vi "TCE.vi"() -> (11 "placeholder image":T1(plugin-control))   [LabVIEW 2022 SP3]
uses:
  DataCluster_TCAL.ctl
  <vilib>/vision/Image Controls.llb/IMAQ Image.ctl
  TCE_Config.ctl
  <vilib>/Utility/file.llb/Read Delimited Spreadsheet (string).vi
  <vilib>/Utility/file.llb/Write Delimited Spreadsheet (string).vi
  <vilib>/Analysis/NI_AALBase.lvlib
panel:
  out "FreezeFract Concatinated":dbl[](array[numeric])
  in  "Correct Data":bool
  out "Offset Applied?":bool
  out "recentPaths":path[](array[path])=[path "D:/OneDrive/OneDrive - Aarhus Universitet/Data/D20_4/Result Data.csv"]
  out "version":string="version 0.0.0.1" caption="Version"
  out "Title":string="Thermal Camera Evaluation" caption="Version"
  in  "Remove_Correction":bool
  out "Offsets":dbl[](array[numeric])
  in  "Calc_All":bool
  in  "Well":i32=251
  in  "ImageIdx":u32(slide)=98 scale=0.0..527.0
  in  "Path":path
  out "MeltTemps":dbl[](array[numeric])=[-5.408275862068933, -5.766551724137912, -5.134827586206882, -4.684827586206836, -7.485172413793066, -5.2834482758620425, -5.345517241379298, -6.320689655172373, -3.992413793103424, -3.7082758620689447, -3.4782758620689265, -5.388275862068895, -5.597241379310333, -4.740689655172389, -4.031034482758571, -4.187241379310308, -6.245172413793114, -4.773793103448213, -4.427586206896535, -3.742413793103424, -4.568965517241338, -5.621379310344764, -4.7503448275861615, -5.029999999999973, -5.895517241379309, -4.551379310344771, -4.0196551724137635, -4.698965517241334, -4.126551724137926, -2.993448275862022, -4.383448275862065, -4.888965517241331, -5.901724137931012, -8.037586206896549, -3.918275862068924, -4.438620689655181, -5.749655172413782, -4.38241379310341, -4.932758620689583, -4.997586206896528, -4.125862068965489, -3.4279310344827536, -5.144482758620654, -2.891379310344803, -2.92999999999995, -3.1620689655172214, -3.216206896551739, -4.3248275862068795, -1.3320689655172373, -2.026551724137903, 0.5675862068965785, -0.5103448275861524, 0.4782758620689833, -1.9634482758620493, -0.1275862068965239, -0.1651724137930728, -0.9937931034482403, -0.6210344827586027, 0.2934482758620902, 0.6917241379310894, 1.3537931034483108, -1.852758620689599, -1.3782758620689037, 1.2606896551724844, -0.0275862068965012, -2.2548275862068294, -1.0710344827585914, -1.4565517241379098, -0.7220689655172237, -0.853793103448254, -0.2686206896551653, -0.5562068965517142, 0.0324137931034443, -0.2768965517241213, 1.1982758620689538, 1.2775862068966148, -0.6427586206896194, 0.5986206896552062, -0.3313793103448006, -0.6034482758620356, -2.0755172413792593, -2.182758620689583, -1.6548275862068635, -0.7234482758620402, -0.6872413793103078, -0.9086206896551516, -0.5427586206895967, -0.0527586206895876, 1.211379310344853, 0.2365517241379393, -0.526551724137903, -0.1537931034482085, 1.1865517241379848, 0.7089655172413813, -1.8837931034482267, 0.5872413793103988, -2.0686206896551766, -2.519310344827545, -2.2079310344827263, -2.2441379310344587, -2.0355172413792957, -2.3782758620689037, -2.0879310344827218, -1.998965517241345, -2.0948275862068613, -2.1227586206896376, -2.195517241379264, -1.969655172413752, -2.0175862068965102, -2.061724137931037, -2.028275862068938, -1.7403448275861706, -2.1765517241378802, -2.432758620689583, -2.186551724137928, -2.063448275862015, -2.331724137931019, -2.1351724137931, -2.0499999999999545, -2.1537931034482085, -2.235172413793066, -2.213793103448211, -2.082758620689617, -2.1703448275861774, -2.0434482758620334, -2.173448275862029, -1.9048275862068635, -1.683793103448238, -1.8931034482758378, -2.165172413793073, -2.068965517241338, -2.1862068965517096, -2.161034482758623, -2.085517241379307, -2.0631034482758537, -2.134137931034445, -2.104827586206852, -2.1775862068965353, -2.2255172413792934, -2.161724137931003, -2.0251724137930864, -2.0106896551724276, -2.211379310344796, -1.9093103448275315, -2.3158620689654867, -1.9827586206895944, -2.258275862068899, -2.2927586206895967, -2.0868965517241236, -2.0810344827585823, -2.17931034482757, -2.134137931034445, -2.151379310344794, -2.101034482758621, -2.2465517241379303, -2.339999999999975, -2.061379310344819, -2.082413793103399, -2.220689655172407, -2.0658620689654867, -2.1337931034482267, -2.0158620689654754, -2.1179310344827513, -2.1999999999999886, -2.130344827586157, -2.0489655172413563, -2.0534482758620243, -2.0851724137930887, -2.1079310344827036, -2.0241379310344882, -2.0693103448275565, -2.1348275862068817, -2.1431034482758378, -2.0268965517241213, -2.0317241379310076, -1.6172413793103146, -2.02103448275858, -2.331724137931019, -2.4068965517241168, -2.2337931034482494, -2.383103448275847, -2.1417241379310212, -2.1768965517240986, -2.2579310344827377, -2.1786206896551334, -2.032068965517226, -2.1162068965517165, -2.2706896551724185, -1.9220689655172123, -2.174482758620684, -2.11206896551721, -2.0858620689654686, -0.1458620689654708, -0.1541379310344837, -0.0103448275861524, -0.2106896551724162, -0.2299999999999613, -0.243448275862022, -0.2624137931034056, -0.2906896551724003, -0.3306896551724208, -0.3089655172413472, -0.2099999999999795, -0.276551724137903, -0.15896551724137, -0.0637931034482335, -0.2572413793103578, 0.1706896551724526, -0.0779310344827309, -0.0958620689654595, 0.0658620689655436, -0.1041379310344723, -0.4631034482758308, -0.1158620689654981, -0.1268965517240872, -0.3313793103448006, -0.2803448275861911, -0.1562068965517369, -0.06793103448274, -0.131379310344812, -0.0282758620689378, 0.0079310344827945, 0.0748275862069363, 0.2665517241379689, 0.0537931034482995, -0.2062068965516914, -0.1179310344827513, -0.3424137931033897, -0.0275862068965012, -0.2003448275861501, -0.1096551724137953, -0.0944827586206429, -0.4137931034482563, -0.5093103448275542, 0.0627586206896922, -0.1789655172413518, -0.0096551724137726, 0.0068965517241395, -0.0334482758620425, 0.2120689655172896, -0.1099999999999568, -0.2282758620689265, -0.1213793103447642, -0.1482758620689424, -0.2106896551724162, -0.0927586206896081, -0.1093103448275201, -0.076206896551696, -0.1593103448275315, -0.0886206896551585, -0.1924137931034124, -0.0558620689654958, -0.0313793103447892, -0.0799999999999841, -0.1262068965517074, 0.2117241379310713, -0.1141379310344632, -0.1796551724137885, -0.2003448275861501, -0.0327586206896058, 0.0655172413793252, -0.1886206896551812, -0.0327586206896058, -0.1424137931034011, -0.2406896551723889, -0.034827586206859, -0.1527586206896103, -0.1848275862068363, -0.0313793103447892, -0.0158620689654754, -0.0372413793103306, 0.2079310344827832, -0.2451724137931137, -0.6586206896551516, -0.0858620689654686, -0.2462068965517119, -0.2631034482758423, -0.0217241379310167, -0.2486206896551266, 0.0455172413793434, -0.2441379310344587, -0.1786206896551334, -0.230689655172398, -0.0131034482758423, -0.2613793103448074, -0.4093103448275315, -0.0124137931034056, 0.1572413793103919, 0.0, 0.0, 0.0, 1.7110344827586346, 1.5944827586206998, 1.9227586206896488, 0.1648275862069113, 1.3268965517241327, 0.0, 0.0, 0.0, 1.441379310344871, 0.8996551724138158, 2.017586206896567, 1.1068965517241622, 2.3413793103448484, 1.119655172413843, 1.9251724137931205, 1.484482758620743, 1.7410344827586641, 1.624137931034511, 1.9227586206896488, 1.88793103448279, 1.3758620689655459, -0.8037931034482426, 1.6562068965517938, 1.90758620689661, 2.0327586206896626, 1.5831034482758923, 2.1006896551724594, 2.216206896551796, 2.153448275862104, 1.9158620689655093, 2.1862068965517665, 1.9189655172414175, 2.0968965517241713, 1.4434482758620675, 1.914482758620693, 1.868620689655188, 1.9841379310345246, 2.0734482758621198, 1.9231034482759242, 1.7982758620689765, 1.852068965517276, 2.086551724137962, 2.055172413793173, 1.9510344827586437, 2.1220689655172578, 2.108620689655197, 2.3431034482758832, 0.0, 1.7272413793103851, 2.039655172413859, 1.9255172413793389, 2.2200000000000273, 1.5868965517241804, 1.914482758620693, 1.9610344827586343, 2.145517241379366, 1.9279310344828102, 1.8203448275862115, 2.199310344827609, 2.312413793103474, 2.407931034482772, 2.4206896551724526, 1.8224137931034647, 2.3637931034483017, 1.6882758620689629, 1.8193103448276133, 1.7324137931034898, 2.3037931034482995, 1.794137931034527, 2.011034482758646, 2.0013793103448734, 1.7558620689655413, 1.8893103448276065, 2.1520689655172873, 1.9962068965517685, 2.3103448275862206, 2.1217241379310963, 1.863103448275922, 1.9231034482759242, 1.5434482758620902, 1.6648275862069113, 1.8944827586207111, 1.63793103448279, 1.8379310344827786, 1.948620689655229, 2.157241379310392, 1.835517241379364, 1.950344827586207, 2.018275862069004, 1.9565517241379666, 1.7651724137931524, 2.068965517241395, 2.168275862068981]
  out "FreezeArray":bool[](array[boolean])=[TRUE, TRUE, TRUE, TRUE, TRUE, TRUE, TRUE, TRUE, TRUE, TRUE, TRUE, TRUE, TRUE, TRUE, TRUE, TRUE, TRUE, TRUE, TRUE, TRUE, TRUE, TRUE, TRUE, TRUE, TRUE, TRUE, TRUE, TRUE, TRUE, TRUE, TRUE, TRUE, TRUE, TRUE, TRUE, TRUE, TRUE, TRUE, TRUE, TRUE, TRUE, TRUE, TRUE, TRUE, TRUE, TRUE, TRUE, TRUE, TRUE, TRUE, TRUE, TRUE, TRUE, TRUE, TRUE, TRUE, TRUE, TRUE, TRUE, TRUE, TRUE, TRUE, TRUE, TRUE, TRUE, TRUE, TRUE, TRUE, TRUE, TRUE, TRUE, TRUE, TRUE, TRUE, TRUE, TRUE, TRUE, TRUE, TRUE, TRUE, TRUE, TRUE, TRUE, TRUE, TRUE, TRUE, TRUE, TRUE, TRUE, TRUE, TRUE, TRUE, TRUE, TRUE, TRUE, TRUE, TRUE, TRUE, TRUE, TRUE, TRUE, TRUE, TRUE, TRUE, TRUE, TRUE, TRUE, TRUE, TRUE, TRUE, TRUE, TRUE, TRUE, TRUE, TRUE, TRUE, TRUE, TRUE, TRUE, TRUE, TRUE, TRUE, TRUE, TRUE, TRUE, TRUE, TRUE, TRUE, TRUE, TRUE, TRUE, TRUE, TRUE, TRUE, TRUE, TRUE, TRUE, TRUE, TRUE, TRUE, TRUE, TRUE, TRUE, TRUE, TRUE, TRUE, TRUE, TRUE, TRUE, TRUE, TRUE, TRUE, TRUE, TRUE, TRUE, TRUE, TRUE, TRUE, TRUE, TRUE, TRUE, TRUE, TRUE, TRUE, TRUE, TRUE, TRUE, TRUE, TRUE, TRUE, TRUE, TRUE, TRUE, TRUE, TRUE, TRUE, TRUE, TRUE, TRUE, TRUE, TRUE, TRUE, TRUE, TRUE, TRUE, TRUE, TRUE, TRUE, TRUE, TRUE, TRUE, TRUE, TRUE, TRUE, TRUE, TRUE, TRUE, TRUE, TRUE, TRUE, TRUE, TRUE, TRUE, TRUE, TRUE, TRUE, TRUE, TRUE, TRUE, TRUE, TRUE, TRUE, TRUE, TRUE, TRUE, TRUE, TRUE, TRUE, TRUE, TRUE, TRUE, TRUE, TRUE, TRUE, TRUE, TRUE, TRUE, TRUE, TRUE, TRUE, TRUE, TRUE, TRUE, TRUE, TRUE, TRUE, TRUE, TRUE, TRUE, TRUE, TRUE, TRUE, TRUE, TRUE, TRUE, TRUE, TRUE, TRUE, TRUE, TRUE, TRUE, TRUE, TRUE, TRUE, TRUE, TRUE, TRUE, TRUE, TRUE, TRUE, TRUE, TRUE, TRUE, TRUE, TRUE, TRUE, TRUE, TRUE, TRUE, TRUE, TRUE, TRUE, TRUE, TRUE, TRUE, TRUE, TRUE, TRUE, TRUE, TRUE, TRUE, TRUE, TRUE, TRUE, TRUE, TRUE, TRUE, TRUE, FALSE, FALSE, FALSE, TRUE, TRUE, TRUE, TRUE, TRUE, FALSE, FALSE, FALSE, TRUE, TRUE, TRUE, TRUE, TRUE, TRUE, TRUE, TRUE, TRUE, TRUE, TRUE, TRUE, TRUE, TRUE, TRUE, TRUE, TRUE, TRUE, TRUE, TRUE, TRUE, TRUE, TRUE, TRUE, TRUE, TRUE, TRUE, TRUE, TRUE, TRUE, TRUE, TRUE, TRUE, TRUE, TRUE, TRUE, TRUE, TRUE, TRUE, FALSE, TRUE, TRUE, TRUE, TRUE, TRUE, TRUE, TRUE, TRUE, TRUE, TRUE, TRUE, TRUE, TRUE, TRUE, TRUE, TRUE, TRUE, TRUE, TRUE, TRUE, TRUE, TRUE, TRUE, TRUE, TRUE, TRUE, TRUE, TRUE, TRUE, TRUE, TRUE, TRUE, TRUE, TRUE, TRUE, TRUE, TRUE, TRUE, TRUE, TRUE, TRUE, TRUE, TRUE, TRUE, TRUE]
  out "ThermTemps":dbl[](array[numeric])
  out "PartitionArray":string[](array[string])=["A, MQ unfiltered", "A, MQ unfiltered", "A, MQ unfiltered", "A, MQ unfiltered", "A, MQ unfiltered", "A, MQ unfiltered", "A, MQ unfiltered", "A, MQ unfiltered", "A, MQ unfiltered", "A, MQ unfiltered", "A, MQ unfiltered", "A, MQ unfiltered", "A, MQ unfiltered", "A, MQ unfiltered", "A, MQ unfiltered", "A, MQ unfiltered", "A, MQ unfiltered", "A, MQ unfiltered", "A, MQ unfiltered", "A, MQ unfiltered", "A, MQ unfiltered", "A, MQ unfiltered", "A, MQ unfiltered", "A, MQ unfiltered", "A, MQ unfiltered", "A, MQ unfiltered", "A, MQ unfiltered", "A, MQ unfiltered", "A, MQ unfiltered", "A, MQ unfiltered", "A, MQ unfiltered", "A, MQ unfiltered", "A, MQ unfiltered", "A, MQ unfiltered", "A, MQ unfiltered", "A, MQ unfiltered", "A, MQ unfiltered", "A, MQ unfiltered", "A, MQ unfiltered", "A, MQ unfiltered", "A, MQ unfiltered", "A, MQ unfiltered", "A, MQ unfiltered", "A, MQ unfiltered", "A, MQ unfiltered", "A, MQ unfiltered", "A, MQ unfiltered", "A, MQ unfiltered", "B, D2O unfiltered", "B, D2O unfiltered", "B, D2O unfiltered", "B, D2O unfiltered", "B, D2O unfiltered", "B, D2O unfiltered", "B, D2O unfiltered", "B, D2O unfiltered", "B, D2O unfiltered", "B, D2O unfiltered", "B, D2O unfiltered", "B, D2O unfiltered", "B, D2O unfiltered", "B, D2O unfiltered", "B, D2O unfiltered", "B, D2O unfiltered", "B, D2O unfiltered", "B, D2O unfiltered", "B, D2O unfiltered", "B, D2O unfiltered", "B, D2O unfiltered", "B, D2O unfiltered", "B, D2O unfiltered", "B, D2O unfiltered", "B, D2O unfiltered", "B, D2O unfiltered", "B, D2O unfiltered", "B, D2O unfiltered", "B, D2O unfiltered", "B, D2O unfiltered", "B, D2O unfiltered", "B, D2O unfiltered", "B, D2O unfiltered", "B, D2O unfiltered", "B, D2O unfiltered", "B, D2O unfiltered", "B, D2O unfiltered", "B, D2O unfiltered", "B, D2O unfiltered", "B, D2O unfiltered", "B, D2O unfiltered", "B, D2O unfiltered", "B, D2O unfiltered", "B, D2O unfiltered", "B, D2O unfiltered", "B, D2O unfiltered", "B, D2O unfiltered", "B, D2O unfiltered", "C, 1mg/ml Snomax in MQ", "C, 1mg/ml Snomax in MQ", "C, 1mg/ml Snomax in MQ", "C, 1mg/ml Snomax in MQ", "C, 1mg/ml Snomax in MQ", "C, 1mg/ml Snomax in MQ", "C, 1mg/ml Snomax in MQ", "C, 1mg/ml Snomax in MQ", "C, 1mg/ml Snomax in MQ", "C, 1mg/ml Snomax in MQ", "C, 1mg/ml Snomax in MQ", "C, 1mg/ml Snomax in MQ", "C, 1mg/ml Snomax in MQ", "C, 1mg/ml Snomax in MQ", "C, 1mg/ml Snomax in MQ", "C, 1mg/ml Snomax in MQ", "C, 1mg/ml Snomax in MQ", "C, 1mg/ml Snomax in MQ", "C, 1mg/ml Snomax in MQ", "C, 1mg/ml Snomax in MQ", "C, 1mg/ml Snomax in MQ", "C, 1mg/ml Snomax in MQ", "C, 1mg/ml Snomax in MQ", "C, 1mg/ml Snomax in MQ", "C, 1mg/ml Snomax in MQ", "C, 1mg/ml Snomax in MQ", "C, 1mg/ml Snomax in MQ", "C, 1mg/ml Snomax in MQ", "C, 1mg/ml Snomax in MQ", "C, 1mg/ml Snomax in MQ", "C, 1mg/ml Snomax in MQ", "C, 1mg/ml Snomax in MQ", "C, 1mg/ml Snomax in MQ", "C, 1mg/ml Snomax in MQ", "C, 1mg/ml Snomax in MQ", "C, 1mg/ml Snomax in MQ", "C, 1mg/ml Snomax in MQ", "C, 1mg/ml Snomax in MQ", "C, 1mg/ml Snomax in MQ", "C, 1mg/ml Snomax in MQ", "C, 1mg/ml Snomax in MQ", "C, 1mg/ml Snomax in MQ", "C, 1mg/ml Snomax in MQ", "C, 1mg/ml Snomax in MQ", "C, 1mg/ml Snomax in MQ", "C, 1mg/ml Snomax in MQ", "C, 1mg/ml Snomax in MQ", "C, 1mg/ml Snomax in MQ", "C, 1mg/ml Snomax in MQ", "C, 1mg/ml Snomax in MQ", "C, 1mg/ml Snomax in MQ", "C, 1mg/ml Snomax in MQ", "C, 1mg/ml Snomax in MQ", "C, 1mg/ml Snomax in MQ", "C, 1mg/ml Snomax in MQ", "C, 1mg/ml Snomax in MQ", "C, 1mg/ml Snomax in MQ", "C, 1mg/ml Snomax in MQ", "C, 1mg/ml Snomax in MQ", "C, 1mg/ml Snomax in MQ", "C, 1mg/ml Snomax in MQ", "C, 1mg/ml Snomax in MQ", "C, 1mg/ml Snomax in MQ", "C, 1mg/ml Snomax in MQ", "C, 1mg/ml Snomax in MQ", "C, 1mg/ml Snomax in MQ", "C, 1mg/ml Snomax in MQ", "C, 1mg/ml Snomax in MQ", "C, 1mg/ml Snomax in MQ", "C, 1mg/ml Snomax in MQ", "C, 1mg/ml Snomax in MQ", "C, 1mg/ml Snomax in MQ", "C, 1mg/ml Snomax in MQ", "C, 1mg/ml Snomax in MQ", "C, 1mg/ml Snomax in MQ", "C, 1mg/ml Snomax in MQ", "C, 1mg/ml Snomax in MQ", "C, 1mg/ml Snomax in MQ", "C, 1mg/ml Snomax in MQ", "C, 1mg/ml Snomax in MQ", "C, 1mg/ml Snomax in MQ", "C, 1mg/ml Snomax in MQ", "C, 1mg/ml Snomax in MQ", "C, 1mg/ml Snomax in MQ", "C, 1mg/ml Snomax in MQ", "C, 1mg/ml Snomax in MQ", "C, 1mg/ml Snomax in MQ", "C, 1mg/ml Snomax in MQ", "C, 1mg/ml Snomax in MQ", "C, 1mg/ml Snomax in MQ", "C, 1mg/ml Snomax in MQ", "C, 1mg/ml Snomax in MQ", "C, 1mg/ml Snomax in MQ", "C, 1mg/ml Snomax in MQ", "C, 1mg/ml Snomax in MQ", "C, 1mg/ml Snomax in MQ", "D, 1mg/ml Snomax in 1:1 MQ:D2O", "D, 1mg/ml Snomax in 1:1 MQ:D2O", "D, 1mg/ml Snomax in 1:1 MQ:D2O", "D, 1mg/ml Snomax in 1:1 MQ:D2O", "D, 1mg/ml Snomax in 1:1 MQ:D2O", "D, 1mg/ml Snomax in 1:1 MQ:D2O", "D, 1mg/ml Snomax in 1:1 MQ:D2O", "D, 1mg/ml Snomax in 1:1 MQ:D2O", "D, 1mg/ml Snomax in 1:1 MQ:D2O", "D, 1mg/ml Snomax in 1:1 MQ:D2O", "D, 1mg/ml Snomax in 1:1 MQ:D2O", "D, 1mg/ml Snomax in 1:1 MQ:D2O", "D, 1mg/ml Snomax in 1:1 MQ:D2O", "D, 1mg/ml Snomax in 1:1 MQ:D2O", "D, 1mg/ml Snomax in 1:1 MQ:D2O", "D, 1mg/ml Snomax in 1:1 MQ:D2O", "D, 1mg/ml Snomax in 1:1 MQ:D2O", "D, 1mg/ml Snomax in 1:1 MQ:D2O", "D, 1mg/ml Snomax in 1:1 MQ:D2O", "D, 1mg/ml Snomax in 1:1 MQ:D2O", "D, 1mg/ml Snomax in 1:1 MQ:D2O", "D, 1mg/ml Snomax in 1:1 MQ:D2O", "D, 1mg/ml Snomax in 1:1 MQ:D2O", "D, 1mg/ml Snomax in 1:1 MQ:D2O", "D, 1mg/ml Snomax in 1:1 MQ:D2O", "D, 1mg/ml Snomax in 1:1 MQ:D2O", "D, 1mg/ml Snomax in 1:1 MQ:D2O", "D, 1mg/ml Snomax in 1:1 MQ:D2O", "D, 1mg/ml Snomax in 1:1 MQ:D2O", "D, 1mg/ml Snomax in 1:1 MQ:D2O", "D, 1mg/ml Snomax in 1:1 MQ:D2O", "D, 1mg/ml Snomax in 1:1 MQ:D2O", "D, 1mg/ml Snomax in 1:1 MQ:D2O", "D, 1mg/ml Snomax in 1:1 MQ:D2O", "D, 1mg/ml Snomax in 1:1 MQ:D2O", "D, 1mg/ml Snomax in 1:1 MQ:D2O", "D, 1mg/ml Snomax in 1:1 MQ:D2O", "D, 1mg/ml Snomax in 1:1 MQ:D2O", "D, 1mg/ml Snomax in 1:1 MQ:D2O", "D, 1mg/ml Snomax in 1:1 MQ:D2O", "D, 1mg/ml Snomax in 1:1 MQ:D2O", "D, 1mg/ml Snomax in 1:1 MQ:D2O", "D, 1mg/ml Snomax in 1:1 MQ:D2O", "D, 1mg/ml Snomax in 1:1 MQ:D2O", "D, 1mg/ml Snomax in 1:1 MQ:D2O", "D, 1mg/ml Snomax in 1:1 MQ:D2O", "D, 1mg/ml Snomax in 1:1 MQ:D2O", "D, 1mg/ml Snomax in 1:1 MQ:D2O", "D, 1mg/ml Snomax in 1:1 MQ:D2O", "D, 1mg/ml Snomax in 1:1 MQ:D2O", "D, 1mg/ml Snomax in 1:1 MQ:D2O", "D, 1mg/ml Snomax in 1:1 MQ:D2O", "D, 1mg/ml Snomax in 1:1 MQ:D2O", "D, 1mg/ml Snomax in 1:1 MQ:D2O", "D, 1mg/ml Snomax in 1:1 MQ:D2O", "D, 1mg/ml Snomax in 1:1 MQ:D2O", "D, 1mg/ml Snomax in 1:1 MQ:D2O", "D, 1mg/ml Snomax in 1:1 MQ:D2O", "D, 1mg/ml Snomax in 1:1 MQ:D2O", "D, 1mg/ml Snomax in 1:1 MQ:D2O", "D, 1mg/ml Snomax in 1:1 MQ:D2O", "D, 1mg/ml Snomax in 1:1 MQ:D2O", "D, 1mg/ml Snomax in 1:1 MQ:D2O", "D, 1mg/ml Snomax in 1:1 MQ:D2O", "D, 1mg/ml Snomax in 1:1 MQ:D2O", "D, 1mg/ml Snomax in 1:1 MQ:D2O", "D, 1mg/ml Snomax in 1:1 MQ:D2O", "D, 1mg/ml Snomax in 1:1 MQ:D2O", "D, 1mg/ml Snomax in 1:1 MQ:D2O", "D, 1mg/ml Snomax in 1:1 MQ:D2O", "D, 1mg/ml Snomax in 1:1 MQ:D2O", "D, 1mg/ml Snomax in 1:1 MQ:D2O", "D, 1mg/ml Snomax in 1:1 MQ:D2O", "D, 1mg/ml Snomax in 1:1 MQ:D2O", "D, 1mg/ml Snomax in 1:1 MQ:D2O", "D, 1mg/ml Snomax in 1:1 MQ:D2O", "D, 1mg/ml Snomax in 1:1 MQ:D2O", "D, 1mg/ml Snomax in 1:1 MQ:D2O", "D, 1mg/ml Snomax in 1:1 MQ:D2O", "D, 1mg/ml Snomax in 1:1 MQ:D2O", "D, 1mg/ml Snomax in 1:1 MQ:D2O", "D, 1mg/ml Snomax in 1:1 MQ:D2O", "D, 1mg/ml Snomax in 1:1 MQ:D2O", "D, 1mg/ml Snomax in 1:1 MQ:D2O", "D, 1mg/ml Snomax in 1:1 MQ:D2O", "D, 1mg/ml Snomax in 1:1 MQ:D2O", "D, 1mg/ml Snomax in 1:1 MQ:D2O", "D, 1mg/ml Snomax in 1:1 MQ:D2O", "D, 1mg/ml Snomax in 1:1 MQ:D2O", "D, 1mg/ml Snomax in 1:1 MQ:D2O", "D, 1mg/ml Snomax in 1:1 MQ:D2O", "D, 1mg/ml Snomax in 1:1 MQ:D2O", "D, 1mg/ml Snomax in 1:1 MQ:D2O", "D, 1mg/ml Snomax in 1:1 MQ:D2O", "D, 1mg/ml Snomax in 1:1 MQ:D2O", "D, 1mg/ml Snomax in 1:1 MQ:D2O", "E, 1mg/ml Snomax in D2O", "E, 1mg/ml Snomax in D2O", "E, 1mg/ml Snomax in D2O", "E, 1mg/ml Snomax in D2O", "E, 1mg/ml Snomax in D2O", "E, 1mg/ml Snomax in D2O", "E, 1mg/ml Snomax in D2O", "E, 1mg/ml Snomax in D2O", "E, 1mg/ml Snomax in D2O", "E, 1mg/ml Snomax in D2O", "E, 1mg/ml Snomax in D2O", "E, 1mg/ml Snomax in D2O", "E, 1mg/ml Snomax in D2O", "E, 1mg/ml Snomax in D2O", "E, 1mg/ml Snomax in D2O", "E, 1mg/ml Snomax in D2O", "E, 1mg/ml Snomax in D2O", "E, 1mg/ml Snomax in D2O", "E, 1mg/ml Snomax in D2O", "E, 1mg/ml Snomax in D2O", "E, 1mg/ml Snomax in D2O", "E, 1mg/ml Snomax in D2O", "E, 1mg/ml Snomax in D2O", "E, 1mg/ml Snomax in D2O", "E, 1mg/ml Snomax in D2O", "E, 1mg/ml Snomax in D2O", "E, 1mg/ml Snomax in D2O", "E, 1mg/ml Snomax in D2O", "E, 1mg/ml Snomax in D2O", "E, 1mg/ml Snomax in D2O", "E, 1mg/ml Snomax in D2O", "E, 1mg/ml Snomax in D2O", "E, 1mg/ml Snomax in D2O", "E, 1mg/ml Snomax in D2O", "E, 1mg/ml Snomax in D2O", "E, 1mg/ml Snomax in D2O", "E, 1mg/ml Snomax in D2O", "E, 1mg/ml Snomax in D2O", "E, 1mg/ml Snomax in D2O", "E, 1mg/ml Snomax in D2O", "E, 1mg/ml Snomax in D2O", "E, 1mg/ml Snomax in D2O", "E, 1mg/ml Snomax in D2O", "E, 1mg/ml Snomax in D2O", "E, 1mg/ml Snomax in D2O", "E, 1mg/ml Snomax in D2O", "E, 1mg/ml Snomax in D2O", "E, 1mg/ml Snomax in D2O", "E, 1mg/ml Snomax in D2O", "E, 1mg/ml Snomax in D2O", "E, 1mg/ml Snomax in D2O", "E, 1mg/ml Snomax in D2O", "E, 1mg/ml Snomax in D2O", "E, 1mg/ml Snomax in D2O", "E, 1mg/ml Snomax in D2O", "E, 1mg/ml Snomax in D2O", "E, 1mg/ml Snomax in D2O", "E, 1mg/ml Snomax in D2O", "E, 1mg/ml Snomax in D2O", "E, 1mg/ml Snomax in D2O", "E, 1mg/ml Snomax in D2O", "E, 1mg/ml Snomax in D2O", "E, 1mg/ml Snomax in D2O", "E, 1mg/ml Snomax in D2O", "E, 1mg/ml Snomax in D2O", "E, 1mg/ml Snomax in D2O", "E, 1mg/ml Snomax in D2O", "E, 1mg/ml Snomax in D2O", "E, 1mg/ml Snomax in D2O", "E, 1mg/ml Snomax in D2O", "E, 1mg/ml Snomax in D2O", "E, 1mg/ml Snomax in D2O", "E, 1mg/ml Snomax in D2O", "E, 1mg/ml Snomax in D2O", "E, 1mg/ml Snomax in D2O", "E, 1mg/ml Snomax in D2O", "E, 1mg/ml Snomax in D2O", "E, 1mg/ml Snomax in D2O", "E, 1mg/ml Snomax in D2O", "E, 1mg/ml Snomax in D2O", "E, 1mg/ml Snomax in D2O", "E, 1mg/ml Snomax in D2O", "E, 1mg/ml Snomax in D2O", "E, 1mg/ml Snomax in D2O", "E, 1mg/ml Snomax in D2O", "E, 1mg/ml Snomax in D2O", "E, 1mg/ml Snomax in D2O", "E, 1mg/ml Snomax in D2O", "E, 1mg/ml Snomax in D2O", "E, 1mg/ml Snomax in D2O", "E, 1mg/ml Snomax in D2O", "E, 1mg/ml Snomax in D2O", "E, 1mg/ml Snomax in D2O", "E, 1mg/ml Snomax in D2O", "E, 1mg/ml Snomax in D2O", "E, 1mg/ml Snomax in D2O"]
  out "FreezeTemps":dbl[](array[numeric])=[-17.102413793103437, -16.14275862068962, -19.01724137931032, -15.683103448275858, -25.12241379310342, -20.5310344827586, -21.968275862068907, -23.725862068965483, -16.464137931034486, -13.113793103448245, -11.636206896551698, -22.81517241379308, -23.049655172413765, -15.513103448275842, -18.779655172413783, -15.36448275862068, -23.218620689655154, -14.564137931034452, -14.352413793103437, -11.641724137931021, -17.657241379310335, -21.99793103448272, -23.813103448275854, -20.459310344827543, -22.592068965517228, -22.526206896551713, -16.890344827586148, -17.801724137931018, -17.235862068965474, -11.44310344827585, -16.035862068965457, -17.472413793103414, -17.914827586206854, -25.26724137931032, -15.10206896551722, -15.265862068965474, -22.079999999999984, -18.58586206896547, -20.5106896551724, -21.002758620689605, -21.88206896551722, -14.302068965517208, -23.049655172413765, -11.56448275862067, -9.727586206896547, -10.574482758620661, -10.471724137931005, -14.189999999999998, -18.853448275862036, -20.565517241379297, -14.187241379310308, -14.840344827586193, -14.906206896551737, -21.08172413793102, -19.829655172413766, -16.151379310344794, -20.792413793103407, -21.82482758620685, -14.474482758620638, -8.87551724137927, -5.148275862068942, -22.100689655172403, -21.813103448275854, -5.387931034482733, -13.19965517241377, -22.069655172413775, -20.66206896551722, -20.594137931034453, -19.319655172413775, -20.309999999999974, -16.707241379310346, -21.968275862068907, -18.70620689655172, -18.623448275862046, -6.637931034482733, -7.056206896551714, -22.052068965517208, -9.618275862068913, -16.901724137931012, -13.387241379310353, -20.70034482758618, -21.344137931034453, -21.40620689655171, -16.127241379310362, -20.572413793103408, -19.566206896551705, -19.49379310344824, -16.083448275862054, -5.782758620689606, -14.221034482758569, -19.863103448275837, -17.482068965517215, -5.9048275862068635, -8.006896551724083, -20.81793103448271, -11.433103448275858, -5.199999999999989, -5.525862068965466, -5.633448275862065, -5.417241379310326, -5.608965517241359, -5.6537931034482085, -5.74655172413793, -5.684482758620675, -5.691379310344814, -5.6758620689655, -5.808620689655129, -5.717586206896556, -5.676206896551719, -5.526896551724121, -5.435517241379273, -5.398620689655161, -5.285172413793077, -5.59172413793101, -5.664482758620636, -5.389999999999986, -5.610344827586175, -5.809999999999945, -5.582413793103399, -5.736896551724101, -5.824482758620661, -5.701379310344805, -5.67655172413788, -5.683103448275858, -5.648965517241322, -5.654482758620645, -5.394482758620654, -5.2789655172413745, -5.4324137931034215, -5.434482758620675, -5.513448275862061, -5.627931034482742, -5.778275862068938, -5.713103448275831, -5.601034482758621, -5.630689655172375, -5.699310344827552, -5.584482758620652, -5.70379310344822, -5.636896551724078, -5.628275862068904, -5.4948275862068385, -5.689310344827561, -5.402413793103392, -5.240689655172389, -5.448275862068897, -5.5555172413792775, -5.998965517241345, -5.548965517241356, -5.420689655172396, -5.645862068965471, -5.577931034482731, -5.6520689655172305, -5.590344827586193, -5.699999999999989, -5.640689655172423, -5.6299999999999955, -5.599310344827529, -5.45034482758615, -5.28793103448271, -5.263793103448222, -5.557931034482749, -5.471034482758569, -5.670344827586177, -5.626551724137926, -5.3606896551723935, -5.553448275862024, -5.736206896551721, -5.485517241379284, -5.536206896551732, -5.615862068965498, -5.4589655172413245, -5.904137931034484, -5.572413793103408, -5.5565517241379325, -5.072413793103408, -5.54482758620685, -5.425172413793064, -5.9865517241378825, -5.601724137931001, -5.816551724137923, -5.833448275862054, -5.495517241379275, -5.722068965517224, -5.5058620689654845, -5.552758620689588, -5.644137931034493, -5.5610344827586005, -5.523793103448213, -5.626551724137926, -5.5406896551724, -5.328275862068949, -2.799310344827518, -3.109999999999957, -3.088965517241377, -3.2558620689654845, -3.3810344827585936, -3.349310344827529, -3.327931034482731, -3.3241379310344428, -3.2679310344827286, -3.4796551724138, -3.1096551724137953, -3.299655172413793, -3.301379310344771, -3.1603448275861865, -2.941034482758596, -2.9506896551724253, -2.8889655172413313, -3.0858620689654686, -2.980689655172398, -3.146896551724126, -3.077931034482731, -3.2044827586206566, -3.164482758620636, -3.3927586206896194, -3.373103448275856, -3.2824137931033874, -3.2603448275861524, -3.264482758620659, -3.188275862068906, -3.086206896551687, -2.978965517241363, -2.9113793103447847, -2.8717241379310394, -3.0813793103448006, -3.0013793103448165, -2.8927586206896194, -3.1879310344827445, -3.2431034482758605, -3.254482758620668, -3.1889655172413427, -3.319655172413775, -3.3893103448275497, -3.1068965517241054, -2.8872413793103533, -2.9982758620689083, -3.2041379310344382, -3.2024137931034033, -2.812413793103417, -2.790344827586182, -3.00068965517238, -3.1693103448275224, -3.193103448275849, -3.195862068965482, -3.1141379310344632, -3.326896551724076, -3.2120689655172328, -3.224137931034477, -3.285862068965457, -3.215862068965464, -3.0582758620689106, -3.1924137931034124, -3.149655172413759, -3.17999999999995, -2.8662068965517165, -2.9058620689654617, -3.0134482758620607, -3.161724137931003, -3.131379310344812, -3.0813793103448006, -3.0351724137930773, -2.9986206896551266, -3.1968965517240804, -3.164482758620636, -3.0810344827585823, -3.220689655172407, -2.9931034482758605, -2.964137931034486, -3.17999999999995, -2.9920689655172055, -2.764827586206877, -2.886896551724078, -3.1758620689655004, -3.071724137931028, -3.196551724137919, -3.2237931034482585, -2.905172413793082, -3.262068965517244, -3.1627586206896012, -3.283793103448261, -3.164482758620636, -3.142413793103401, -3.1089655172413586, -3.034137931034479, -3.277586206896558, -3.0720689655172464, -2.629655172413777, 0.0, 0.0, 0.0, -0.7296551724137998, -1.1386206896551698, -1.0558620689654958, -1.305172413793116, -1.1862068965517096, 0.0, 0.0, 0.0, -1.1282758620689037, -1.1682758620689242, -0.5724137931034079, -1.1765517241378802, -0.2555172413792661, -1.0703448275861547, -0.7648275862068772, -1.057931034482749, -1.016551724137912, -0.9627586206896126, -1.0337931034482608, -0.9872413793103192, -1.2451724137931137, -1.3141379310344519, -1.0437931034482517, -1.0199999999999818, -0.95310344827584, -0.9817241379309962, -0.8799999999999955, -0.7527586206896331, -0.5689655172413381, -0.6779310344827536, -0.7651724137930955, -0.8879310344827331, -0.8582758620689219, -1.0286206896551562, -0.8986206896551607, -1.072413793103408, -0.8858620689654799, -0.9524137931034033, -0.9465517241379189, -0.9465517241379189, -0.6958620689654822, -0.9386206896551812, -0.6879310344827445, -0.8244827586206611, -0.540344827586182, -0.5341379310344792, -0.6255172413792707, 0.0, -0.8917241379310212, -0.8031034482758628, -0.7927586206895967, -0.3927586206896194, -1.0141379310344405, -0.7241379310344769, -0.8258620689654776, -0.8099999999999454, -0.7320689655172146, -0.8993103448275406, -0.6624137931034397, -0.5572413793103124, -0.355517241379289, 0.0244827586207066, -0.6931034482758491, -0.113103448275865, -0.8486206896551494, -0.581724137931019, -0.4658620689654641, -0.1306896551723753, -0.9151724137930728, -0.8689655172413495, -0.5741379310344428, -0.8624137931034284, -0.8899999999999864, -0.8365517241379052, -0.7541379310344496, -0.5631034482758537, -0.4710344827585686, -0.3586206896551403, -0.4551724137930933, -0.7186206896551539, -0.8586206896551403, -0.6134482758620265, -0.6841379310344564, -0.6020689655172191, -0.8358620689654686, -0.6906896551723776, -0.8324137931033988, -0.900689655172414, -0.5879310344827218, -0.8486206896551494, -0.6179310344827513, -0.4758620689654549, -0.4237931034482472]
  out "FreezeIdx":i32[](array[numeric])=[255, 242, 272, 236, 335, 287, 303, 320, 243, 209, 191, 311, 316, 234, 271, 238, 322, 225, 219, 192, 254, 301, 321, 283, 307, 309, 248, 257, 253, 193, 240, 259, 264, 335, 231, 232, 302, 265, 285, 291, 301, 219, 312, 192, 172, 182, 181, 221, 271, 285, 224, 228, 233, 290, 279, 240, 286, 296, 218, 162, 122, 305, 300, 128, 213, 302, 285, 284, 271, 280, 243, 297, 267, 262, 143, 147, 302, 170, 248, 214, 293, 293, 293, 240, 287, 272, 273, 236, 129, 217, 278, 252, 135, 153, 288, 192, 124, 131, 130, 125, 127, 127, 126, 129, 124, 127, 126, 126, 129, 126, 124, 128, 126, 126, 135, 125, 133, 136, 126, 131, 132, 131, 126, 125, 129, 132, 125, 128, 128, 127, 124, 126, 136, 130, 125, 129, 125, 134, 131, 126, 130, 125, 133, 128, 125, 130, 133, 137, 127, 124, 126, 124, 127, 126, 133, 130, 124, 133, 132, 124, 124, 129, 126, 128, 128, 123, 132, 131, 125, 127, 125, 124, 136, 126, 129, 126, 129, 126, 135, 126, 133, 130, 124, 126, 124, 124, 126, 123, 125, 125, 124, 129, 98, 100, 98, 105, 99, 102, 98, 100, 97, 104, 97, 98, 100, 99, 97, 99, 99, 105, 99, 106, 107, 99, 108, 104, 104, 100, 100, 98, 103, 98, 98, 99, 102, 106, 108, 96, 100, 108, 104, 99, 100, 108, 98, 97, 97, 99, 98, 98, 99, 99, 99, 110, 108, 100, 111, 100, 99, 107, 99, 98, 101, 99, 99, 99, 98, 98, 99, 99, 101, 107, 98, 99, 100, 98, 104, 98, 98, 99, 99, 98, 98, 99, 98, 100, 101, 100, 106, 101, 100, 99, 100, 99, 98, 102, 99, 98, 0, 0, 0, 71, 80, 75, 84, 81, 0, 0, 0, 74, 77, 72, 78, 75, 81, 73, 76, 80, 77, 76, 76, 82, 88, 77, 78, 79, 74, 74, 81, 78, 76, 75, 75, 77, 76, 82, 75, 74, 76, 83, 81, 72, 74, 73, 74, 74, 73, 79, 0, 79, 74, 75, 82, 76, 73, 80, 75, 73, 82, 73, 75, 79, 80, 77, 77, 74, 73, 73, 89, 77, 75, 71, 76, 76, 74, 74, 75, 73, 74, 71, 76, 78, 74, 74, 72, 75, 75, 75, 75, 73, 77, 73, 73, 75]
  out "maxSize":i32=527
  out "img":i32
  out "Slide":u8(slide) scale=0.0..100.0
  in  "Help":bool
  out "Tutorial":string="Load Image"
  out "Points":T2[](array[typedef])=[{"X"=62.0, "Y"=65.0}, {"X"=62.333332, "Y"=80.6}, {"X"=62.666668, "Y"=96.2}, {"X"=63.0, "Y"=111.8}, {"X"=63.333332, "Y"=127.4}, {"X"=63.666668, "Y"=143.0}, {"X"=64.0, "Y"=158.6}, {"X"=64.333336, "Y"=174.20001}, {"X"=64.666664, "Y"=189.8}, {"X"=65.0, "Y"=205.40001}, {"X"=65.333336, "Y"=221.0}, {"X"=65.666664, "Y"=236.6}, {"X"=66.0, "Y"=252.20001}, {"X"=66.333336, "Y"=267.8}, {"X"=66.666664, "Y"=283.40002}, {"X"=67.0, "Y"=299.0}, {"X"=77.565216, "Y"=64.695656}, {"X"=77.89855, "Y"=80.295654}, {"X"=78.23188, "Y"=95.89565}, {"X"=78.565216, "Y"=111.49565}, {"X"=78.89855, "Y"=127.09566}, {"X"=79.23188, "Y"=142.69565}, {"X"=79.565216, "Y"=158.29565}, {"X"=79.89855, "Y"=173.89566}, {"X"=80.23188, "Y"=189.49567}, {"X"=80.565216, "Y"=205.09566}, {"X"=80.89855, "Y"=220.69565}, {"X"=81.23188, "Y"=236.29565}, {"X"=81.565216, "Y"=251.89566}, {"X"=81.89855, "Y"=267.49567}, {"X"=82.23188, "Y"=283.09564}, {"X"=82.565216, "Y"=298.69565}, {"X"=93.13043, "Y"=64.391304}, {"X"=93.46377, "Y"=79.9913}, {"X"=93.797104, "Y"=95.59131}, {"X"=94.13043, "Y"=111.19131}, {"X"=94.46377, "Y"=126.791306}, {"X"=94.797104, "Y"=142.3913}, {"X"=95.13043, "Y"=157.9913}, {"X"=95.46377, "Y"=173.59131}, {"X"=95.797104, "Y"=189.19131}, {"X"=96.13043, "Y"=204.79132}, {"X"=96.46377, "Y"=220.39131}, {"X"=96.797104, "Y"=235.99132}, {"X"=97.13043, "Y"=251.59132}, {"X"=97.46377, "Y"=267.1913}, {"X"=97.797104, "Y"=282.79132}, {"X"=98.13043, "Y"=298.3913}, {"X"=108.69565, "Y"=64.08696}, {"X"=109.028984, "Y"=79.68696}, {"X"=109.36232, "Y"=95.28696}, {"X"=109.695656, "Y"=110.88696}, {"X"=110.028984, "Y"=126.48695}, {"X"=110.36232, "Y"=142.08696}, {"X"=110.695656, "Y"=157.68697}, {"X"=111.028984, "Y"=173.28696}, {"X"=111.36232, "Y"=188.88696}, {"X"=111.695656, "Y"=204.48697}, {"X"=112.028984, "Y"=220.08696}, {"X"=112.36232, "Y"=235.68697}, {"X"=112.695656, "Y"=251.28697}, {"X"=113.028984, "Y"=266.88696}, {"X"=113.36232, "Y"=282.48697}, {"X"=113.695656, "Y"=298.08698}, {"X"=124.260864, "Y"=63.782608}, {"X"=124.5942, "Y"=79.38261}, {"X"=124.927536, "Y"=94.982605}, {"X"=125.26087, "Y"=110.58261}, {"X"=125.5942, "Y"=126.18261}, {"X"=125.927536, "Y"=141.78261}, {"X"=126.26087, "Y"=157.38261}, {"X"=126.5942, "Y"=172.9826}, {"X"=126.927536, "Y"=188.58261}, {"X"=127.26087, "Y"=204.18262}, {"X"=127.5942, "Y"=219.78261}, {"X"=127.927536, "Y"=235.38261}, {"X"=128.26086, "Y"=250.98262}, {"X"=128.59421, "Y"=266.5826}, {"X"=128.92754, "Y"=282.18262}, {"X"=129.26086, "Y"=297.7826}, {"X"=139.82608, "Y"=63.47826}, {"X"=140.15942, "Y"=79.07826}, {"X"=140.49275, "Y"=94.67826}, {"X"=140.8261, "Y"=110.27826}, {"X"=141.15942, "Y"=125.878265}, {"X"=141.49275, "Y"=141.47827}, {"X"=141.8261, "Y"=157.07828}, {"X"=142.15942, "Y"=172.67827}, {"X"=142.49275, "Y"=188.27826}, {"X"=142.8261, "Y"=203.87827}, {"X"=143.15942, "Y"=219.47826}, {"X"=143.49275, "Y"=235.07826}, {"X"=143.8261, "Y"=250.67827}, {"X"=144.15942, "Y"=266.27826}, {"X"=144.49275, "Y"=281.87827}, {"X"=144.8261, "Y"=297.47827}, {"X"=155.3913, "Y"=63.173912}, {"X"=155.72464, "Y"=78.77391}, {"X"=156.05797, "Y"=94.37392}, {"X"=156.39131, "Y"=109.973915}, {"X"=156.72464, "Y"=125.57391}, {"X"=157.05797, "Y"=141.17392}, {"X"=157.39131, "Y"=156.77393}, {"X"=157.72464, "Y"=172.37392}, {"X"=158.05797, "Y"=187.9739}, {"X"=158.39131, "Y"=203.57393}, {"X"=158.72464, "Y"=219.17392}, {"X"=159.05797, "Y"=234.77393}, {"X"=159.39131, "Y"=250.37393}, {"X"=159.72464, "Y"=265.97394}, {"X"=160.05797, "Y"=281.5739}, {"X"=160.39131, "Y"=297.17392}, {"X"=170.95651, "Y"=62.869564}, {"X"=171.28986, "Y"=78.46957}, {"X"=171.62318, "Y"=94.069565}, {"X"=171.95653, "Y"=109.66957}, {"X"=172.28986, "Y"=125.26956}, {"X"=172.62318, "Y"=140.86957}, {"X"=172.95653, "Y"=156.46957}, {"X"=173.28986, "Y"=172.06958}, {"X"=173.62318, "Y"=187.66957}, {"X"=173.95653, "Y"=203.26958}, {"X"=174.28986, "Y"=218.86957}, {"X"=174.62318, "Y"=234.46957}, {"X"=174.95653, "Y"=250.06958}, {"X"=175.28986, "Y"=265.66956}, {"X"=175.62318, "Y"=281.2696}, {"X"=175.95653, "Y"=296.86957}, {"X"=186.52173, "Y"=62.565216}, {"X"=186.85507, "Y"=78.16522}, {"X"=187.1884, "Y"=93.76522}, {"X"=187.52174, "Y"=109.36522}, {"X"=187.85507, "Y"=124.96522}, {"X"=188.1884, "Y"=140.56522}, {"X"=188.52174, "Y"=156.16522}, {"X"=188.85507, "Y"=171.76523}, {"X"=189.1884, "Y"=187.36522}, {"X"=189.52174, "Y"=202.96523}, {"X"=189.85507, "Y"=218.56522}, {"X"=190.1884, "Y"=234.16522}, {"X"=190.52174, "Y"=249.76523}, {"X"=190.85507, "Y"=265.36523}, {"X"=191.1884, "Y"=280.9652}, {"X"=191.52174, "Y"=296.56522}, {"X"=202.08696, "Y"=62.260868}, {"X"=202.42029, "Y"=77.86087}, {"X"=202.75363, "Y"=93.46087}, {"X"=203.08696, "Y"=109.06087}, {"X"=203.42029, "Y"=124.66087}, {"X"=203.75363, "Y"=140.26086}, {"X"=204.08696, "Y"=155.86087}, {"X"=204.42029, "Y"=171.46088}, {"X"=204.75363, "Y"=187.06088}, {"X"=205.08696, "Y"=202.66087}, {"X"=205.42029, "Y"=218.26086}, {"X"=205.75363, "Y"=233.86087}, {"X"=206.08696, "Y"=249.46088}, {"X"=206.42029, "Y"=265.06085}, {"X"=206.75363, "Y"=280.6609}, {"X"=207.08696, "Y"=296.26086}, {"X"=217.65218, "Y"=61.95652}, {"X"=217.9855, "Y"=77.55652}, {"X"=218.31885, "Y"=93.156525}, {"X"=218.65218, "Y"=108.75652}, {"X"=218.9855, "Y"=124.35652}, {"X"=219.31885, "Y"=139.95651}, {"X"=219.65218, "Y"=155.55652}, {"X"=219.9855, "Y"=171.15652}, {"X"=220.31885, "Y"=186.75653}, {"X"=220.65218, "Y"=202.35654}, {"X"=220.9855, "Y"=217.95653}, {"X"=221.31885, "Y"=233.55653}, {"X"=221.65218, "Y"=249.15654}, {"X"=221.9855, "Y"=264.75653}, {"X"=222.31885, "Y"=280.35654}, {"X"=222.65218, "Y"=295.95654}, {"X"=233.21739, "Y"=61.652176}, {"X"=233.55072, "Y"=77.252174}, {"X"=233.88406, "Y"=92.85217}, {"X"=234.21739, "Y"=108.45218}, {"X"=234.55072, "Y"=124.05218}, {"X"=234.88406, "Y"=139.65218}, {"X"=235.21739, "Y"=155.25218}, {"X"=235.55072, "Y"=170.85217}, {"X"=235.88406, "Y"=186.45218}, {"X"=236.21739, "Y"=202.05219}, {"X"=236.55072, "Y"=217.65218}, {"X"=236.88406, "Y"=233.25218}, {"X"=237.21739, "Y"=248.85219}, {"X"=237.55072, "Y"=264.45218}, {"X"=237.88406, "Y"=280.0522}, {"X"=238.21739, "Y"=295.65216}, {"X"=248.78261, "Y"=61.347828}, {"X"=249.11594, "Y"=76.94783}, {"X"=249.44928, "Y"=92.54783}, {"X"=249.78261, "Y"=108.14783}, {"X"=250.11594, "Y"=123.74783}, {"X"=250.44928, "Y"=139.34782}, {"X"=250.78261, "Y"=154.94783}, {"X"=251.11594, "Y"=170.54782}, {"X"=251.44928, "Y"=186.14783}, {"X"=251.78261, "Y"=201.74783}, {"X"=252.11594, "Y"=217.34782}, {"X"=252.44928, "Y"=232.94783}, {"X"=252.78261, "Y"=248.54784}, {"X"=253.11594, "Y"=264.14783}, {"X"=253.44928, "Y"=279.74783}, {"X"=253.78261, "Y"=295.34784}, {"X"=264.34784, "Y"=61.04348}, {"X"=264.68115, "Y"=76.64348}, {"X"=265.0145, "Y"=92.24348}, {"X"=265.34784, "Y"=107.84348}, {"X"=265.68115, "Y"=123.44348}, {"X"=266.0145, "Y"=139.04349}, {"X"=266.34784, "Y"=154.6435}, {"X"=266.68115, "Y"=170.24348}, {"X"=267.0145, "Y"=185.84348}, {"X"=267.34784, "Y"=201.44348}, {"X"=267.68115, "Y"=217.04347}, {"X"=268.0145, "Y"=232.64348}, {"X"=268.34784, "Y"=248.24348}, {"X"=268.68115, "Y"=263.84348}, {"X"=269.0145, "Y"=279.44348}, {"X"=269.34784, "Y"=295.04346}, {"X"=279.91302, "Y"=60.739132}, {"X"=280.24637, "Y"=76.33913}, {"X"=280.5797, "Y"=91.93913}, {"X"=280.91306, "Y"=107.53914}, {"X"=281.24637, "Y"=123.13913}, {"X"=281.5797, "Y"=138.73914}, {"X"=281.91306, "Y"=154.33914}, {"X"=282.24637, "Y"=169.93913}, {"X"=282.5797, "Y"=185.53912}, {"X"=282.91306, "Y"=201.13914}, {"X"=283.24637, "Y"=216.73914}, {"X"=283.5797, "Y"=232.33914}, {"X"=283.91306, "Y"=247.93915}, {"X"=284.24637, "Y"=263.53912}, {"X"=284.5797, "Y"=279.13916}, {"X"=284.91306, "Y"=294.73914}, {"X"=295.47827, "Y"=60.434784}, {"X"=295.81158, "Y"=76.03478}, {"X"=296.14493, "Y"=91.63478}, {"X"=296.47827, "Y"=107.23479}, {"X"=296.81158, "Y"=122.834785}, {"X"=297.14493, "Y"=138.43478}, {"X"=297.47827, "Y"=154.03479}, {"X"=297.81158, "Y"=169.6348}, {"X"=298.14493, "Y"=185.23479}, {"X"=298.47827, "Y"=200.8348}, {"X"=298.81158, "Y"=216.43478}, {"X"=299.14493, "Y"=232.03479}, {"X"=299.47827, "Y"=247.6348}, {"X"=299.81158, "Y"=263.2348}, {"X"=300.14493, "Y"=278.83478}, {"X"=300.47827, "Y"=294.43478}, {"X"=311.04346, "Y"=60.130436}, {"X"=311.3768, "Y"=75.73044}, {"X"=311.71014, "Y"=91.33044}, {"X"=312.0435, "Y"=106.930435}, {"X"=312.3768, "Y"=122.53044}, {"X"=312.71014, "Y"=138.13043}, {"X"=313.0435, "Y"=153.73044}, {"X"=313.3768, "Y"=169.33044}, {"X"=313.71014, "Y"=184.93044}, {"X"=314.0435, "Y"=200.53044}, {"X"=314.3768, "Y"=216.13043}, {"X"=314.71014, "Y"=231.73044}, {"X"=315.0435, "Y"=247.33044}, {"X"=315.3768, "Y"=262.93042}, {"X"=315.71014, "Y"=278.53046}, {"X"=316.0435, "Y"=294.13043}, {"X"=326.6087, "Y"=59.826088}, {"X"=326.94205, "Y"=75.42609}, {"X"=327.27536, "Y"=91.02609}, {"X"=327.6087, "Y"=106.62609}, {"X"=327.94205, "Y"=122.22609}, {"X"=328.27536, "Y"=137.82608}, {"X"=328.6087, "Y"=153.42609}, {"X"=328.94205, "Y"=169.0261}, {"X"=329.27536, "Y"=184.6261}, {"X"=329.6087, "Y"=200.22609}, {"X"=329.94205, "Y"=215.82608}, {"X"=330.27536, "Y"=231.42609}, {"X"=330.6087, "Y"=247.0261}, {"X"=330.94205, "Y"=262.6261}, {"X"=331.27536, "Y"=278.22607}, {"X"=331.6087, "Y"=293.82608}, {"X"=342.17392, "Y"=59.52174}, {"X"=342.50726, "Y"=75.12174}, {"X"=342.84058, "Y"=90.72174}, {"X"=343.17392, "Y"=106.32175}, {"X"=343.50726, "Y"=121.92174}, {"X"=343.84058, "Y"=137.52173}, {"X"=344.17392, "Y"=153.12173}, {"X"=344.50726, "Y"=168.72174}, {"X"=344.84058, "Y"=184.32175}, {"X"=345.17392, "Y"=199.92175}, {"X"=345.50726, "Y"=215.52174}, {"X"=345.84058, "Y"=231.12175}, {"X"=346.17392, "Y"=246.72176}, {"X"=346.50726, "Y"=262.32175}, {"X"=346.84058, "Y"=277.92175}, {"X"=347.17392, "Y"=293.52173}, {"X"=357.73914, "Y"=59.217392}, {"X"=358.07248, "Y"=74.81739}, {"X"=358.4058, "Y"=90.41739}, {"X"=358.73914, "Y"=106.017395}, {"X"=359.07248, "Y"=121.61739}, {"X"=359.4058, "Y"=137.21739}, {"X"=359.73914, "Y"=152.8174}, {"X"=360.07248, "Y"=168.41739}, {"X"=360.4058, "Y"=184.0174}, {"X"=360.73914, "Y"=199.6174}, {"X"=361.07248, "Y"=215.21739}, {"X"=361.4058, "Y"=230.8174}, {"X"=361.73914, "Y"=246.4174}, {"X"=362.07248, "Y"=262.0174}, {"X"=362.4058, "Y"=277.6174}, {"X"=362.73914, "Y"=293.2174}, {"X"=373.30435, "Y"=58.913044}, {"X"=373.6377, "Y"=74.51305}, {"X"=373.971, "Y"=90.113045}, {"X"=374.30435, "Y"=105.71304}, {"X"=374.6377, "Y"=121.31305}, {"X"=374.971, "Y"=136.91304}, {"X"=375.30435, "Y"=152.51305}, {"X"=375.6377, "Y"=168.11305}, {"X"=375.971, "Y"=183.71304}, {"X"=376.30435, "Y"=199.31305}, {"X"=376.6377, "Y"=214.91304}, {"X"=376.971, "Y"=230.51305}, {"X"=377.30435, "Y"=246.11305}, {"X"=377.6377, "Y"=261.71304}, {"X"=377.971, "Y"=277.31305}, {"X"=378.30435, "Y"=292.91302}, {"X"=388.86957, "Y"=58.608696}, {"X"=389.2029, "Y"=74.208694}, {"X"=389.53622, "Y"=89.8087}, {"X"=389.86957, "Y"=105.4087}, {"X"=390.2029, "Y"=121.0087}, {"X"=390.53622, "Y"=136.6087}, {"X"=390.86957, "Y"=152.20871}, {"X"=391.2029, "Y"=167.8087}, {"X"=391.53622, "Y"=183.40869}, {"X"=391.86957, "Y"=199.0087}, {"X"=392.2029, "Y"=214.6087}, {"X"=392.53622, "Y"=230.20871}, {"X"=392.86957, "Y"=245.80872}, {"X"=393.2029, "Y"=261.4087}, {"X"=393.53622, "Y"=277.0087}, {"X"=393.86957, "Y"=292.6087}, {"X"=404.43478, "Y"=58.304348}, {"X"=404.76813, "Y"=73.90435}, {"X"=405.10144, "Y"=89.50435}, {"X"=405.43478, "Y"=105.104355}, {"X"=405.76813, "Y"=120.704346}, {"X"=406.10144, "Y"=136.30435}, {"X"=406.43478, "Y"=151.90436}, {"X"=406.76813, "Y"=167.50435}, {"X"=407.10144, "Y"=183.10435}, {"X"=407.43478, "Y"=198.70436}, {"X"=407.76813, "Y"=214.30435}, {"X"=408.10144, "Y"=229.90436}, {"X"=408.43478, "Y"=245.50436}, {"X"=408.76813, "Y"=261.10437}, {"X"=409.10144, "Y"=276.70435}, {"X"=409.43478, "Y"=292.30435}, {"X"=420.0, "Y"=58.0}, {"X"=420.33334, "Y"=73.6}, {"X"=420.66666, "Y"=89.2}, {"X"=421.0, "Y"=104.8}, {"X"=421.33334, "Y"=120.4}, {"X"=421.66666, "Y"=136.0}, {"X"=422.0, "Y"=151.6}, {"X"=422.33334, "Y"=167.20001}, {"X"=422.66666, "Y"=182.8}, {"X"=423.0, "Y"=198.40001}, {"X"=423.33334, "Y"=214.0}, {"X"=423.66666, "Y"=229.6}, {"X"=424.0, "Y"=245.20001}, {"X"=424.33334, "Y"=260.8}, {"X"=424.66666, "Y"=276.40002}, {"X"=425.0, "Y"=292.0}] {"Y" format="%.2f"; "X" format="%.2f"}
  out "Image":T1(plugin-control)
  out "MeltTemp":dbl=-0.0558620689654958 caption="Melt temp" format="%.3g °C"
  out "FreezeTemp":dbl=-3.0582758620689106 caption="Froze at" format="%.3g °C"
  out "Title 2":string="Well Data" caption="Version"
  out "Well":string="L16"
  out "CurTemp":dbl=-0.9882758620689174 caption="Temp" format="%.3g °C"
  out "Contents":string="D, 1mg/ml Snomax in 1:1 MQ:D2O"
  out "Temps":dbl[][](graph)
  out "Temps single":dbl[](graph)
  out "Fraction Single":dbl[](graph)=[0.0, 0.0, 0.0, 0.0, 0.0, 0.0, 0.0, 0.0, 0.0, 0.0, 0.0, 0.0, 0.0, 0.0, 0.0, 0.0, 0.0, 0.0, 0.0, 0.0, 0.0, 0.0, 0.0, 0.0, 0.0, 0.0, 0.0, 0.0, 0.0, 0.0, 0.0, 0.0, 0.0, 0.0, 0.0, 0.0, 0.0, 0.0, 0.0, 0.0, 0.0, 0.0, 0.0, 0.0, 0.0, 0.0, 0.0, 0.0, 0.0, 0.0, 0.0, 0.0, 0.0, 0.0, 0.0, 0.0, 0.0, 0.0, 0.0, 0.0, 0.0, 0.0, 0.0, 0.0, 0.0, 0.0, 0.0, 0.0, 0.0, 0.0, 0.0, 0.0, 0.0, 0.0, 0.0, 0.0, 0.0, 0.0, 0.0, 0.0, 0.0, 0.0, 0.0, 0.0, 0.0, 0.0, 0.0, 0.0, 0.0, 0.0, 0.0, 0.0, 0.0, 0.0, 0.0, 0.0, 0.0, 0.05263157894736842, 0.28421052631578947, 0.5578947368421052, 0.7052631578947368, 0.7473684210526316, 0.7789473684210526, 0.7894736842105263, 0.8421052631578947, 0.8631578947368421, 0.8947368421052632, 0.9263157894736842, 0.9789473684210527, 0.9789473684210527, 0.9894736842105263, 1.0, 1.0, 1.0, 1.0, 1.0, 1.0, 1.0, 1.0, 1.0, 1.0, 1.0, 1.0, 1.0, 1.0, 1.0, 1.0, 1.0, 1.0, 1.0, 1.0, 1.0, 1.0, 1.0, 1.0, 1.0, 1.0, 1.0, 1.0, 1.0, 1.0, 1.0, 1.0, 1.0, 1.0, 1.0, 1.0, 1.0, 1.0, 1.0, 1.0, 1.0, 1.0, 1.0, 1.0, 1.0, 1.0, 1.0, 1.0, 1.0, 1.0, 1.0, 1.0, 1.0, 1.0, 1.0, 1.0, 1.0, 1.0, 1.0, 1.0, 1.0, 1.0, 1.0, 1.0, 1.0, 1.0, 1.0, 1.0, 1.0, 1.0, 1.0, 1.0, 1.0, 1.0, 1.0, 1.0, 1.0, 1.0, 1.0, 1.0, 1.0, 1.0, 1.0, 1.0, 1.0, 1.0, 1.0, 1.0, 1.0, 1.0, 1.0, 1.0, 1.0, 1.0, 1.0, 1.0, 1.0, 1.0, 1.0, 1.0, 1.0, 1.0, 1.0, 1.0, 1.0, 1.0, 1.0, 1.0, 1.0, 1.0, 1.0, 1.0, 1.0, 1.0, 1.0, 1.0, 1.0, 1.0, 1.0, 1.0, 1.0, 1.0, 1.0, 1.0, 1.0, 1.0, 1.0, 1.0, 1.0, 1.0, 1.0, 1.0, 1.0, 1.0, 1.0, 1.0, 1.0, 1.0, 1.0, 1.0, 1.0, 1.0, 1.0, 1.0, 1.0, 1.0, 1.0, 1.0, 1.0, 1.0, 1.0, 1.0, 1.0, 1.0, 1.0, 1.0, 1.0, 1.0, 1.0, 1.0, 1.0, 1.0, 1.0, 1.0, 1.0, 1.0, 1.0, 1.0, 1.0, 1.0, 1.0, 1.0, 1.0, 1.0, 1.0, 1.0, 1.0, 1.0, 1.0, 1.0, 1.0, 1.0, 1.0, 1.0, 1.0, 1.0, 1.0, 1.0, 1.0, 1.0, 1.0, 1.0, 1.0, 1.0, 1.0, 1.0, 1.0, 1.0, 1.0, 1.0, 1.0, 1.0, 1.0, 1.0, 1.0, 1.0, 1.0, 1.0, 1.0, 1.0, 1.0, 1.0, 1.0, 1.0, 1.0, 1.0, 1.0, 1.0, 1.0, 1.0, 1.0, 1.0, 1.0, 1.0, 1.0, 1.0, 1.0, 1.0, 1.0, 1.0, 1.0, 1.0, 1.0, 1.0, 1.0, 1.0, 1.0, 1.0, 1.0, 1.0, 1.0, 1.0, 1.0, 1.0, 1.0, 1.0, 1.0, 1.0, 1.0, 1.0, 1.0, 1.0, 1.0, 1.0, 1.0, 1.0, 1.0, 1.0, 1.0, 1.0, 1.0, 1.0, 1.0, 1.0, 1.0, 1.0, 1.0, 1.0, 1.0, 1.0, 1.0, 1.0, 1.0, 1.0, 1.0, 1.0, 1.0, 1.0, 1.0, 1.0, 1.0, 1.0, 1.0, 1.0, 1.0, 1.0, 1.0, 1.0, 1.0, 1.0, 1.0, 1.0, 1.0, 1.0, 1.0, 1.0, 1.0, 1.0, 1.0, 1.0, 1.0, 1.0, 1.0, 1.0, 1.0, 1.0, 1.0, 1.0, 1.0, 1.0, 1.0, 1.0, 1.0, 1.0, 1.0, 1.0, 1.0, 1.0, 1.0, 1.0, 1.0, 1.0, 1.0, 1.0, 1.0, 1.0, 1.0, 1.0, 1.0, 1.0, 1.0, 1.0, 1.0, 1.0, 1.0, 1.0, 1.0, 1.0, 1.0, 1.0, 1.0, 1.0, 1.0, 1.0, 1.0, 1.0, 1.0, 1.0, 1.0, 1.0, 1.0, 1.0, 1.0, 1.0, 1.0, 1.0, 1.0, 1.0, 1.0, 1.0, 1.0, 1.0, 1.0, 1.0, 1.0, 1.0, 1.0, 1.0, 1.0, 1.0, 1.0, 1.0, 1.0, 1.0, 1.0, 1.0, 1.0, 1.0, 1.0, 1.0, 1.0, 1.0, 1.0, 1.0, 1.0, 1.0, 1.0, 1.0, 1.0, 1.0, 1.0, 1.0, 1.0, 1.0, 1.0, 1.0, 1.0, 1.0, 1.0, 1.0, 1.0, 1.0, 1.0, 1.0, 1.0, 1.0, 1.0, 1.0, 1.0, 1.0, 1.0, 1.0, 1.0, 1.0, 1.0, 1.0, 1.0]
  out "FrozenFractionGraph":dbl[][](graph)
  out "Temps single grad":dbl[](graph)
  out "Temps grads":dbl[][](graph)
  # "hints: \nUse the Mouse Wheel to zoom in and out"
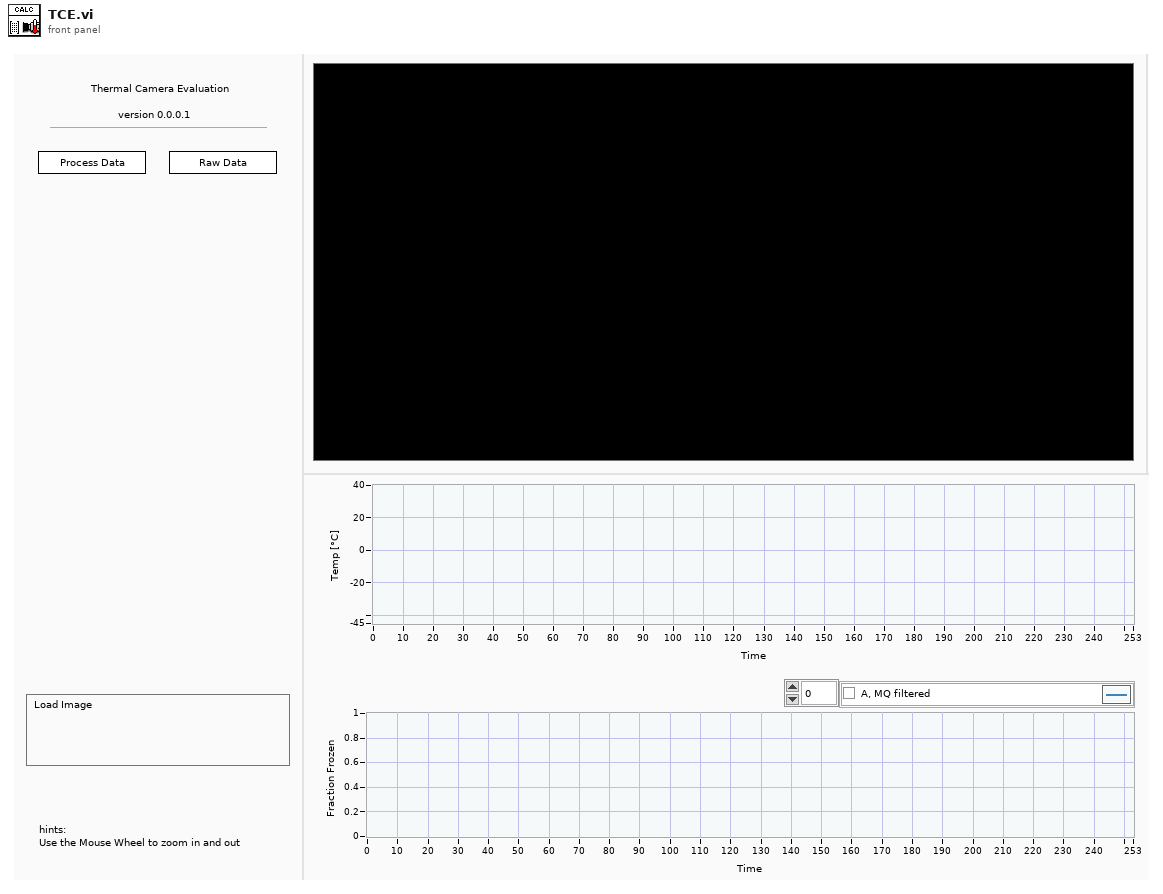
[diagram p1: front panel]
types:
  T1 = typedef "IMAQ Image.ctl" = refnum<image>
  T2 = typedef "IMAQ Point" = cluster{"X":sgl, "Y":sgl}
  T3 = typedef "TCE_Config.ctl" = cluster{"Freezing":cluster{"Cutoff":dbl, "EndIndex":i32}}
  T4 = typedef "DataCluster_TCAL.ctl" = cluster{"Core":cluster{"Current VI Reference":refnum<vi>, "Close Panel on Exit?":bool}, "Image Out":T1, "State":i32, "Points":cluster{"Top Left":T2, "Top Right":T2, "Bottom Left":T2, "Bottom Right":T2, "x space 2":dbl, "y space 2":sgl, "x_space":sgl, "y_space":sgl, "Pixels":cluster{"X":i32, "Y":i32}[][], "Fixpoint":T2}, "img_array":T1[], "Temps":dbl[], "Temps_Array":dbl[][], "Scan Area":dbl, "Fixpoint Area":dbl, "Config":T3, "PCR Size":u16, "ImageCount":i32, "ShowGradient":bool}
  T5 = enum32{"Invalid", "Standard", "Closed", "Hidden", "Minimized", "Maximized"}
  T6 = enum32{"invalid app kind", "Development System", "Run Time System", "Student Edition", "Embedded LabVIEW", "Evaluation", "Custom"}
  T7 = cluster{"Global Rectangle":i32[], "Contours":cluster{"Contour Type":u32, "ROI Type":u32, "Points":i32[]}[]}
  T8 = enum8{"Enabled", "Disabled", "Disabled and Grayed Out"}
  T9 = cluster{"Desired Font (Application)":enum16{"User-specified Font", "Application Font", "System Font", "Dialog Font"}, "[User-specified Font]":cluster{"Font Name":string, "Size":i16, "Strikeout?":bool, "Italic?":bool, "Underline?":bool, "Outline?":bool, "Shadow?":bool, "Bold?":bool, "Rotation Angle":dbl}, "Horizontal Alignment":i16, "Vertical Alignment":i16}
  T10 = typedef "ROI Descriptor" = cluster{"Global Rectangle":i32[], "Contours":cluster{"ID":enum32{"External", "Internal"}, "Type":u32, "Coordinates":i32[]}[]}
  T11 = cluster{"Current VI Reference":refnum<vi>, "Close Panel on Exit?":bool}
  T12 = typedef "Image Type" = u32
  T13 = cluster{"Top Left":T2, "Top Right":T2, "Bottom Left":T2, "Bottom Right":T2, "x space 2":dbl, "y space 2":sgl, "x_space":sgl, "y_space":sgl, "Pixels":cluster{"X":i32, "Y":i32}[][], "Fixpoint":T2}
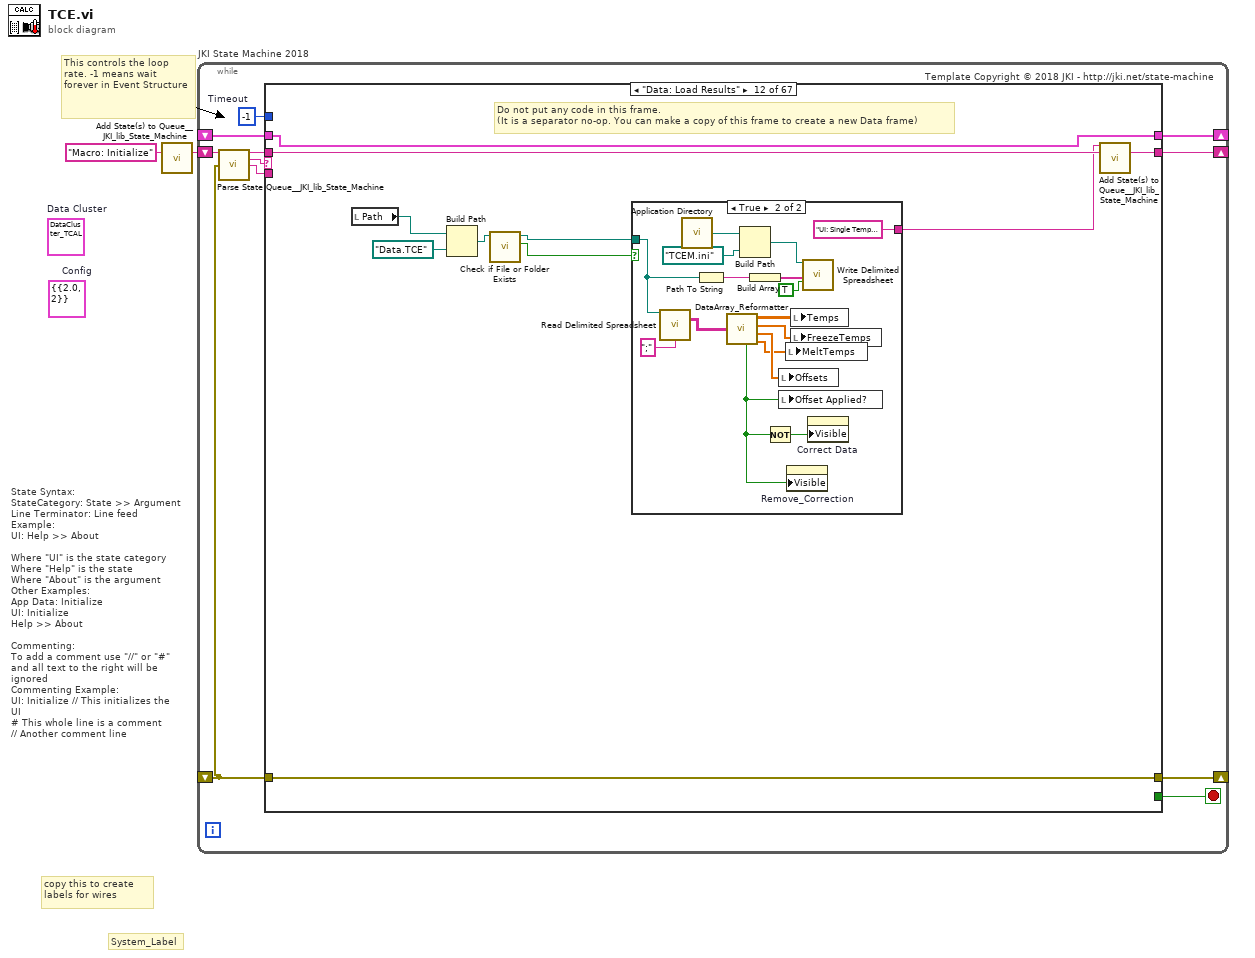
[diagram p0: block diagram]
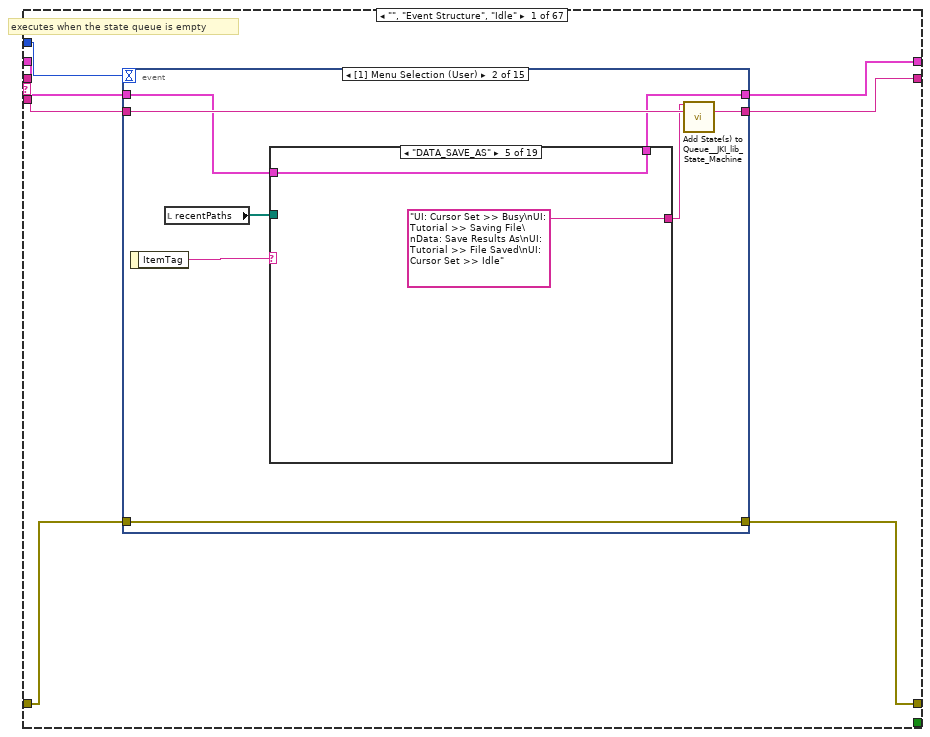
[diagram p2: hidden frame]
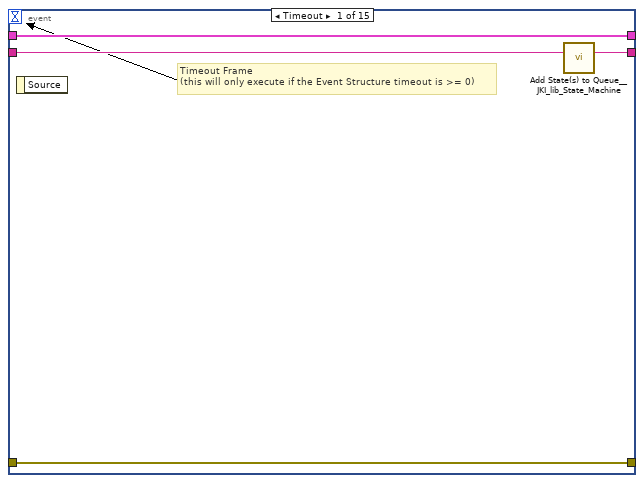
[diagram p3: hidden frame]
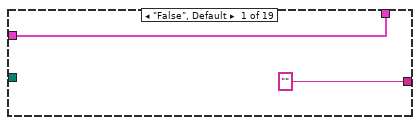
[diagram p4: hidden frame]
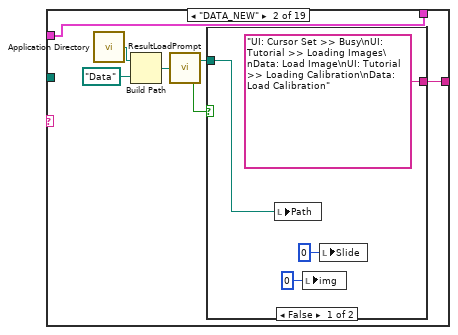
[diagram p5: hidden frame]
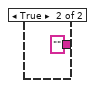
[diagram p6: hidden frame]
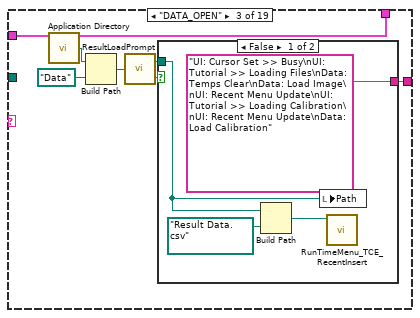
[diagram p7: hidden frame]
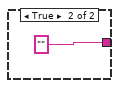
[diagram p8: hidden frame]
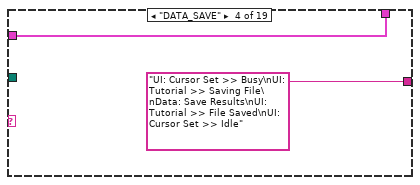
[diagram p9: hidden frame]
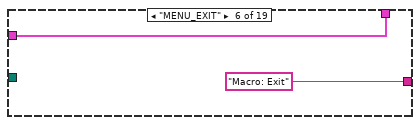
[diagram p10: hidden frame]
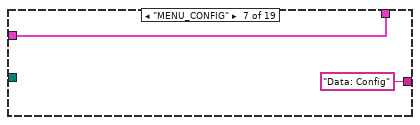
[diagram p11: hidden frame]
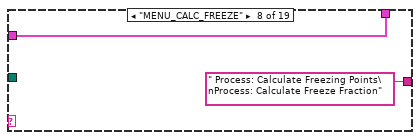
[diagram p12: hidden frame]
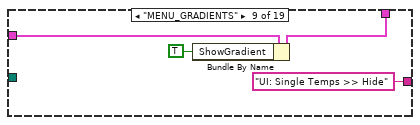
[diagram p13: hidden frame]
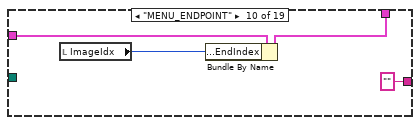
[diagram p14: hidden frame]
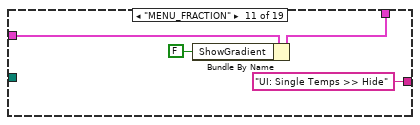
[diagram p15: hidden frame]
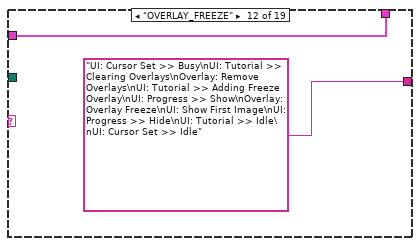
[diagram p16: hidden frame]
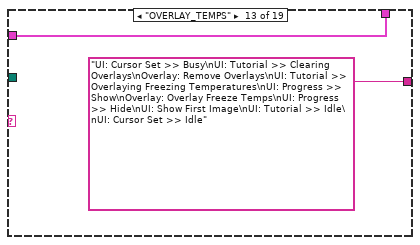
[diagram p17: hidden frame]
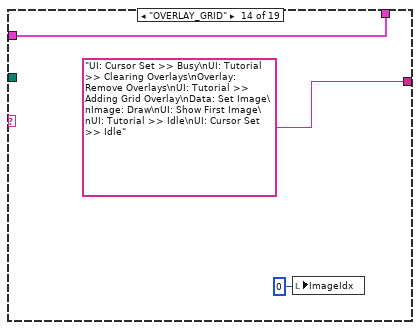
[diagram p18: hidden frame]
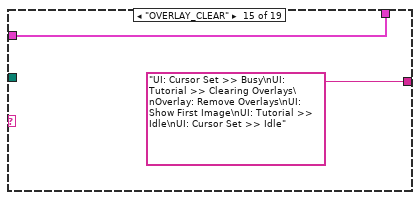
[diagram p19: hidden frame]
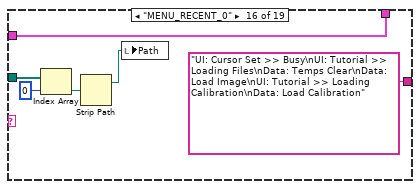
[diagram p20: hidden frame]
diagram:
  (unwired) T3 {"Freezing"={"Cutoff"=2.0, "EndIndex"=2}}  # Config
  (unwired) T4 {"Core"={"Current VI Reference"=refnum, "Close Panel on Exit?"=FALSE}, "Image Out"=refnum, "State"=0, "Points"={"Top Left"={"X"=0.0, "Y"=0.0}, "Top Right"={"X"=0.0, "Y"=0.0}, "Bottom Left"={"X"=0.0, "Y"=0.0}, "Bottom Right"={"X"=0.0, "Y"=0.0}, "x space 2"=0.0, "y space 2"=0.0, "x_space"=0.0, "y_space"=0.0, "Pixels"=[], "Fixpoint"={"X"=0.0, "Y"=0.0}}, "img_array"=[], "Temps"=[], "Temps_Array"=[], "Scan Area"=0.0, "Fixpoint Area"=0.0, "Config"={"Freezing"={"Cutoff"=2.0, "EndIndex"=2}}, "PCR Size"=0, "ImageCount"=0, "ShowGradient"=FALSE}  # Data Cluster
  # "State Syntax:\nStateCategory: State >> Argument\nLine Terminator: Line feed\nExample:\nUI: Help >> About\n\nWhere \"UI\" is the state category\nWhere \"Help\" is the state\nWhere \"About\" is the argument\nOther Examples:\nApp Data: Initialize\nUI: Initialize\nHelp >> About\n\nCommenting:\nTo add a comment use \"//\" or \"#\" and all text to the right will be ignored\nCommenting Example:\nUI: Initialize // This initializes the UI\n# This whole line is a comment\n// Another comment line"
  # "copy this to create labels for wires"
  # "This controls the loop rate. -1 means wait forever in Event Structure"
  # "System_Label"
  n1 = call <vilib>:"Add State(s) to Queue__JKI_lib_State_Machine.vi"("State(s) in (\"\")"="Macro: Initialize") -> ("States Out"=w2:string)  [unwired: 14 in]
  n2 = while "JKI State Machine 2018" {
    shift-right: [w6] -> _
    shift-left: _ -> [w5]
    shift-right: [w9] -> _
    shift-left: _ -> [w3]
    shift-right: [w8] -> _
    shift-left: w2 -> [w10]
    stop <- w7 stop-if-true
    w4 = -1  # Timeout
    # "Template Copyright © 2018 JKI - http://jki.net/state-machine"
    n3 = call <vilib>:"Parse State Queue__JKI_lib_State_Machine.vi"("State Queue"=w10, "Error In (no error)"=w3) -> ("Remaining States"=w12:string, "Current State"=w13:string, "Arguments"=w11:string)  [unwired: 11 in]
    n4 = case shown="\"Data: Load Results\"" w13 {
      selector: w13 -> [_ _ w230 _ _ _ _ _ _ _ _ _ _ _ _ _ _ _ _ _ _ _ _ _ _ _ _ _ _ _ _ _ _ _ _ _ _ _ _ _ _ _ _ _ _ _ _ _ _ _ _ _ _ _ _ _ _ _ _ _ _ _ _ _ _ _ _]
      tunnel: w12 -> [w20 w229 w234 w253 w259 w264 w268 w285 w294 w302 w319 w375 w403 w433 w438 w445 w452 w468 w519 w548 w583 w591 w599 w606 w611 w618 w630 w642 w652 w662 w677 w694 w763 w768 w778 w782 w787 w792 w809 w831 w875 w904 w934 w960 w981 w989 w996 w1006 w1013 w1018 w1023 w1032 w1052 w1069 w1135 w1161 w1181 w1199 w1215 w1224 w1233 w1245 w1254 w1294 w1338 w1373 w1389]
      tunnel: w11 -> [_ _ _ _ _ _ _ _ _ _ _ _ _ _ _ _ _ _ _ _ _ w587 _ _ w607 w614 w625 w638 w648 w658 w674 w688 _ _ _ _ _ _ _ _ _ _ _ _ _ _ _ _ _ _ _ _ _ w1067 _ _ _ _ _ _ _ _ _ _ _ _ _]
      tunnel: w5 -> [w18 w226 w232 w246 w256 w262 w265 _ w292 w299 w306 w372 w396 w430 w434 w442 w449 w466 w510 w545 w581 w589 w597 w603 w609 w616 w628 w640 w650 w660 w671 w690 w760 w765 w775 w779 w784 w789 w798 w815 w861 w901 w927 w957 w978 w986 w993 w1003 w1010 w1015 w1020 w1029 w1033 w1065 w1122 w1152 w1172 w1190 w1204 w1222 w1228 w1242 w1251 w1291 w1333 w1370 w1380]
      tunnel: [w17 w227 w236 w250 errorcluster {"status"=FALSE, "code"=0, "source"=""} ("error out") w261 w266 w274 w291 w300 w308 w373 w401 w427 w436 w443 w450 w453 w504 w546 w580 w588 w596 w604 w608 w615 w626 w639 w649 w659 w675 w691 w761 w766 w776 w780 w785 w790 w807 w829 w873 w902 w932 w958 w979 w987 w994 w1004 w1011 w1016 w1021 w1030 w1050 w1062 w1132 w1159 w1179 w1197 w1213 w1219 w1225 w1243 w1252 w1292 w1336 w1371 w1387] -> w9
      tunnel: w3 -> [w16 w227 w235 w250 w255 w261 w266 w274 w288 w300 w315 w373 w401 w427 w436 w443 w450 w453 w504 w546 w580 w588 w596 w604 w608 w615 w627 w639 w649 w659 w675 w692 w761 w766 w776 w780 w785 w790 w807 w829 w873 w902 w932 w958 w979 w987 w994 w1004 w1011 w1016 w1021 w1030 w1050 w1063 w1132 w1159 w1179 w1197 w1213 w1220 w1227 w1243 w1252 w1292 w1336 w1371 w1387]
      tunnel: [w19 w228 w233 w252 w258 w263 w267 w284 w293 w301 w318 w374 w402 w432 w437 w444 w451 w467 w518 w547 w582 w590 w598 w605 w610 w617 w629 w641 w651 w661 w676 w693 w762 w767 w777 w781 w786 w791 w808 w830 w874 w903 w933 w959 w980 w988 w995 w1005 w1012 w1017 w1022 w1031 w1051 w1068 w1134 w1160 w1180 w1198 w1214 w1223 w1232 w1244 w1253 w1293 w1337 w1372 w1388] -> w8
      tunnel: [_ _ _ _ _ TRUE _ _ _ _ _ _ _ _ _ _ _ _ _ _ _ _ _ _ _ _ _ _ _ _ _ _ _ _ _ _ _ _ _ _ _ _ _ _ _ _ _ _ _ _ _ _ _ _ _ _ _ _ _ _ _ _ _ _ _ _ _] -> w7
      tunnel: [w15 w226 w232 w251 w256 w262 w265 w283 w292 w298 w317 w372 w395 w431 w434 w442 w448 w466 w510 w545 w581 w589 w597 w603 w609 w616 w628 w640 w650 w660 w671 w690 w760 w765 w775 w779 w784 w789 w798 w814 w861 w901 w927 w957 w978 w986 w993 w1003 w1010 w1015 w1020 w1029 w1033 w1065 w1121 w1151 w1171 w1189 w1204 w1222 w1228 w1242 w1251 w1291 w1333 w1370 w1380] -> w6
      tunnel: w4 -> [w14 _ _ _ _ _ _ _ _ _ _ _ _ _ _ _ _ _ _ _ _ _ _ _ _ _ _ _ _ _ _ _ _ _ _ _ _ _ _ _ _ _ _ _ _ _ _ _ _ _ _ _ _ _ _ _ _ _ _ _ _ _ _ _ _ _ _]
      frame "", "Event Structure", "Idle" {
        # "executes when the state queue is empty"
        n5 = event shown="[1] Menu Selection (User)" {
          selector: _ -> [_ _ _ _ _ _ _ _ _ _ _ _ _ _ _]
          dyn-events: _ -> [_ _ _ _ _ _ _ _ _ _ _ _ _ _ _]
          timeout: w14 -> [_ _ _ _ _ _ _ _ _ _ _ _ _ _ _]
          tunnel: w20 -> [w24 w32 w117 w129 w139 w145 w154 w163 w172 w181 w190 w199 w209 w217 w225]
          tunnel: [w23 w31 w116 w128 w138 w144 w153 w162 w171 w180 w189 w198 w208 w216 w224] -> w19
          tunnel: w18 -> [w21 w26 w114 w126 w136 w142 w151 w160 w169 w178 w187 w196 w206 w214 w222]
          tunnel: [w22 w30 w115 w127 w137 w143 w152 w161 w170 w179 w188 w197 w207 w215 w223] -> w17
          tunnel: w16 -> [w22 w30 w115 w127 w137 w143 w152 w161 w170 w179 w188 w197 w207 w215 w223]
          tunnel: [w21 w25 w114 w126 w136 w142 w151 w160 w169 w178 w187 w196 w206 w214 w222] -> w15
          event Timeout {
            # "Timeout Frame\n(this will only execute if the Event Structure timeout is >= 0)"
            n6 = event-data() -> ()  [unwired: 1 in, 1 out]
            n7 = call <vilib>:"Add State(s) to Queue__JKI_lib_State_Machine.vi"("State(s) in (\"\")"=w24) -> ("States Out"=w23:string)  [unwired: 14 in]
          }
          event Menu Selection (User) {
            n8 = event-data() -> ("ItemTag"=w29:string)  [unwired: 1 in]
            n9 = local read "recentPaths"() -> (w27:path[])
            n10 = case shown="\"DATA_SAVE_AS\"" w29 {
              tunnel: ["" w41 w53 "UI: Cursor Set >> Busy\nUI: Tutorial >> Saving File\nData: Save Results\nUI: Tutorial >> File Saved\nUI: Cursor Set >> Idle" "UI: Cursor Set >> Busy\nUI: Tutorial >> Saving File\nData: Save Results As\nUI: Tutorial >> File Saved\nUI: Cursor Set >> Idle" "Macro: Exit" "Data: Config" " Process: Calculate Freezing Points\nProcess: Calculate Freeze Fraction" "UI: Single Temps >> Hide" "" "UI: Single Temps >> Hide" "UI: Cursor Set >> Busy\nUI: Tutorial >> Clearing Overlays\nOverlay: Remove Overlays\nUI: Tutorial >> Adding Freeze Overlay\nUI: Progress >> Show\nOverlay: Overlay Freeze\nUI: Show First Image\nUI: Progress >> Hide\nUI: Tutorial >> Idle\nUI: Cursor Set >> Idle" "UI: Cursor Set >> Busy\nUI: Tutorial >> Clearing Overlays\nOverlay: Remove Overlays\nUI: Tutorial >> Overlaying Freezing Temperatures\nUI: Progress >> Show\nOverlay: Overlay Freeze Temps\nUI: Progress >> Hide\nUI: Show First Image\nUI: Tutorial >> Idle\nUI: Cursor Set >> Idle" "UI: Cursor Set >> Busy\nUI: Tutorial >> Clearing Overlays\nOverlay: Remove Overlays\nUI: Tutorial >> Adding Grid Overlay\nData: Set Image\nImage: Draw\nUI: Show First Image\nUI: Tutorial >> Idle\nUI: Cursor Set >> Idle" "UI: Cursor Set >> Busy\nUI: Tutorial >> Clearing Overlays\nOverlay: Remove Overlays\nUI: Show First Image\nUI: Tutorial >> Idle\nUI: Cursor Set >> Idle" "UI: Cursor Set >> Busy\nUI: Tutorial >> Loading Files\nData: Temps Clear\nData: Load Image\nUI: Tutorial >> Loading Calibration\nData: Load Calibration" "UI: Cursor Set >> Busy\nUI: Tutorial >> Loading Files\nData: Temps Clear\nData: Load Image\nUI: Tutorial >> Loading Calibration\nData: Load Calibration" "UI: Cursor Set >> Busy\nUI: Tutorial >> Loading Files\nData: Temps Clear\nData: Load Image\nUI: Tutorial >> Loading Calibration\nData: Load Calibration" "UI: Cursor Set >> Busy\nUI: Tutorial >> Loading Files\nData: Temps Clear\nData: Load Image\nUI: Tutorial >> Loading Calibration\nData: Load Calibration"] -> w28
              tunnel: w27 -> [_ _ _ _ _ _ _ _ _ _ _ _ _ _ _ w94 w100 w106 w112]
              tunnel: w26 -> [w33 w35 w47 w59 w61 w63 w65 w67 w71 w75 w79 w81 w83 w85 w88 w90 w96 w102 w108]
              tunnel: [w33 w35 w47 w59 w61 w63 w65 w67 w70 w74 w78 w81 w83 w85 w88 w90 w96 w102 w108] -> w25
              frame "False", Default {
              }
              frame "DATA_NEW" {
                n11 = call <vilib>:"Application Directory.vi"() -> ("Application Directory"=w40:path)
                n12 = Build Path(base path=w40, name or relative path=path "Data") -> (appended path=w39:path)
                n13 = call "ResultLoadPrompt.vi"("Path"=w39) -> ("selected path"=w36:path, "cancel?"=w37:bool)
                n14 = case shown="False" w37 {
                  tunnel: ["UI: Cursor Set >> Busy\nUI: Tutorial >> Loading Images\nData: Load Image\nUI: Tutorial >> Loading Calibration\nData: Load Calibration" ""] -> w41
                  tunnel: w36 -> [w42 _]
                  frame False {
                    n15 = local write "Path"(w42) -> ()
                    n16 = local write "img"(0 ("img")) -> ()
                    n17 = local write "Slide"(u8 0 ("Slide")) -> ()
                  }
                  frame True {
                  }
                }
              }
              frame "DATA_OPEN" {
                n18 = call <vilib>:"Application Directory.vi"() -> ("Application Directory"=w52:path)
                n19 = Build Path(base path=w52, name or relative path=path "Data") -> (appended path=w50:path)
                n20 = call "ResultLoadPrompt.vi"("Path"=w50) -> ("selected path"=w49:path, "cancel?"=w48:bool)
                n21 = case shown="False" w48 {
                  tunnel: ["UI: Cursor Set >> Busy\nUI: Tutorial >> Loading Files\nData: Temps Clear\nData: Load Image\nUI: Recent Menu Update\nUI: Tutorial >> Loading Calibration\nUI: Recent Menu Update\nData: Load Calibration" ""] -> w53
                  tunnel: w49 -> [w56 _]
                  frame False {
                    n22 = Build Path(base path=w56, name or relative path=path "Result Data.csv") -> (appended path=w54:path)
                    n23 = local write "Path"(w56) -> ()
                    n24 = call "RunTimeMenu_TCE_RecentInsert.vi"("NewPath"=w54) -> ()  [unwired: 11 in]
                  }
                  frame True {
                  }
                }
              }
              frame "DATA_SAVE" {
              }
              frame "DATA_SAVE_AS" {
              }
              frame "MENU_EXIT" {
              }
              frame "MENU_CONFIG" {
              }
              frame "MENU_CALC_FREEZE" {
              }
              frame "MENU_GRADIENTS" {
                n25 = Bundle By Name(cluster=w71, "ShowGradient"=TRUE) -> (w70:T4)
              }
              frame "MENU_ENDPOINT" {
                n26 = local read "ImageIdx"() -> (w73:u32)
                n27 = Bundle By Name(cluster=w75, "Config.Freezing.EndIndex"=w73) -> (w74:T4)
              }
              frame "MENU_FRACTION" {
                n28 = Bundle By Name(cluster=w79, "ShowGradient"=FALSE) -> (w78:T4)
              }
              frame "OVERLAY_FREEZE" {
              }
              frame "OVERLAY_TEMPS" {
              }
              frame "OVERLAY_GRID" {
                n29 = local write "ImageIdx"(0 ("img")) -> ()
              }
              frame "OVERLAY_CLEAR" {
              }
              frame "MENU_RECENT_0" {
                n30 = Index Array(array=w94, index=0) -> (element=w92:path)
                n31 = Strip Path(path=w92) -> (stripped path=w91:path)  [unwired: 1 out]
                n32 = local write "Path"(w91) -> ()
              }
              frame "MENU_RECENT_1" {
                n33 = Index Array(array=w100, index=1) -> (element=w98:path)
                n34 = Strip Path(path=w98) -> (stripped path=w97:path)  [unwired: 1 out]
                n35 = local write "Path"(w97) -> ()
              }
              frame "MENU_RECENT_2" {
                n36 = Index Array(array=w106, index=2) -> (element=w104:path)
                n37 = Strip Path(path=w104) -> (stripped path=w103:path)  [unwired: 1 out]
                n38 = local write "Path"(w103) -> ()
              }
              frame "MENU_RECENT_3" {
                n39 = Index Array(array=w112, index=3) -> (element=w110:path)
                n40 = Strip Path(path=w110) -> (stripped path=w109:path)  [unwired: 1 out]
                n41 = local write "Path"(w109) -> ()
              }
            }
            n42 = call <vilib>:"Add State(s) to Queue__JKI_lib_State_Machine.vi"("State(s) in Front (\"\")"=w28, "State(s) in (\"\")"=w32) -> ("States Out"=w31:string)  [unwired: 13 in]
          }
          event "Help": Value Change {
            # "Timeout Frame\n(this will only execute if the Event Structure timeout is >= 0)"
            n43 = event-data() -> ()  [unwired: 1 in, 6 out]
            n44 = call <vilib>:"Add State(s) to Queue__JKI_lib_State_Machine.vi"("State(s) in (\"\")"=w117) -> ("States Out"=w116:string)  [unwired: 14 in]
          }
          event "Image": Mouse Wheel {
            n45 = event-data() -> ("Delta"=w125:i32)  [unwired: 1 in, 1 out]
            n46 = property on="Image" class="ImageControl"() -> ("Last Mouse Position"=w119:cluster{"X":i32, "Y":i32}, "X Zoom"=w120:sgl)  [unwired: 2 in, 2 out]
            n47 = Greater Than 0?(x=w125) -> (x > 0?=w124:bool)
            n48 = Select(t=1.2, s=w124, f=0.8) -> (s? t:f=w121:dbl)
            n49 = Multiply(x=w121, y=w120) -> (x*y=w118:dbl)
            n50 = property on="Image" class="ImageControl"("X Zoom"=w118, "Y Zoom"=w118, "Image Center Position"=w119) -> ()  [unwired: 2 in, 2 out]
            n51 = call <vilib>:"Add State(s) to Queue__JKI_lib_State_Machine.vi"("State(s) in (\"\")"=w129) -> ("States Out"=w128:string)  [unwired: 14 in]
          }
          event "Image": Mouse Up {
            n52 = event-data() -> ()  [unwired: 1 in, 1 out]
            n53 = property on="Image" class="ImageControl"() -> ("Last Mouse Position"=w135:cluster{"X":i32, "Y":i32})  [unwired: 2 in, 2 out]
            n54 = local read "Temps"() -> (w130:dbl[][])
            n55 = local read "Points"() -> (w134:T2[])
            n56 = call "SingleWellUpdater.vi"("Temps"=w130, "Well Coordinates"=w134, "Last Mouse Position"=w135) -> ("Well idx"=w131:i32, "ROI Descriptor"=w132:T10, "State out"=w133:string)  [unwired: 6 in]
            n57 = property on="Image" class="ImageControl"("ROI"=w132) -> ()  [unwired: 2 in, 2 out]
            n58 = local write "Well"(w131) -> ()
            n59 = call <vilib>:"Add State(s) to Queue__JKI_lib_State_Machine.vi"("State(s) in Front (\"\")"=w133, "State(s) in (\"\")"=w139) -> ("States Out"=w138:string)  [unwired: 13 in]
          }
          event Panel Close? {
            # "Discard the event because we'll close the front panel ourselves in Macro: Exit"
            # "Close Panel button (pressed) Event\n(this executes Macro: Exit to terminate the VI)"
            n60 = event-data() -> ()  [unwired: 1 in, 1 out]
            n61 = call <vilib>:"Add State(s) to Queue__JKI_lib_State_Machine.vi"("State(s) in Front (\"\")"="Macro: Exit", "State(s) in (\"\")"=w145) -> ("States Out"=w144:string)  [unwired: 13 in]
            n62 = event-data("Discard?"=TRUE) -> ()  [unwired: 1 in, 1 out]
          }
          event "Temps single": Cursor Move {
            n63 = event-data() -> ()  [unwired: 1 in, 9 out]
            n64 = property on="Temps single" class="WFGraph (strict)"() -> ("Cursor.Cursor X"=w149:dbl)  [unwired: 2 in, 2 out]
            n65 = local read "maxSize"() -> (w148:i32)
            n66 = In Range and Coerce(upper limit=w148, x=w149, lower limit=0) -> (coerced(x)=w146:dbl)  [unwired: 1 out]
            n67 = local write "ImageIdx"(w146) -> ()
            n68 = call <vilib>:"Add State(s) to Queue__JKI_lib_State_Machine.vi"("State(s) in Front (\"\")"="Image: Set Cursors\nData: Set Image\nData: Show Img\nData: Update Well Temp", "State(s) in (\"\")"=w154) -> ("States Out"=w153:string)  [unwired: 13 in]
          }
          event "Temps": Cursor Move {
            n69 = event-data() -> ()  [unwired: 1 in, 1 out]
            n70 = property on="Temps" class="WFGraph (strict)"() -> ("Cursor.Cursor X"=w158:dbl)  [unwired: 2 in, 2 out]
            n71 = local read "maxSize"() -> (w156:i32)
            n72 = In Range and Coerce(upper limit=w156, x=w158, lower limit=0) -> (coerced(x)=w155:dbl)  [unwired: 1 out]
            n73 = local write "ImageIdx"(w155) -> ()
            n74 = call <vilib>:"Add State(s) to Queue__JKI_lib_State_Machine.vi"("State(s) in Front (\"\")"="Image: Set Cursors\nData: Set Image\nData: Show Img\nData: Update Well Temp", "State(s) in (\"\")"=w163) -> ("States Out"=w162:string)  [unwired: 13 in]
          }
          event "Temps single grad": Cursor Move {
            n75 = event-data() -> ()  [unwired: 1 in, 1 out]
            n76 = property on="Temps single grad" class="WFGraph (strict)"() -> ("Cursor.Cursor X"=w167:dbl)  [unwired: 2 in, 2 out]
            n77 = local read "maxSize"() -> (w165:i32)
            n78 = In Range and Coerce(upper limit=w165, x=w167, lower limit=0) -> (coerced(x)=w164:dbl)  [unwired: 1 out]
            n79 = local write "ImageIdx"(w164) -> ()
            n80 = call <vilib>:"Add State(s) to Queue__JKI_lib_State_Machine.vi"("State(s) in Front (\"\")"="Image: Set Cursors\nData: Set Image\nData: Show Img\nData: Update Well Temp", "State(s) in (\"\")"=w172) -> ("States Out"=w171:string)  [unwired: 13 in]
          }
          event "FrozenFractionGraph": Cursor Move {
            n81 = event-data() -> ()  [unwired: 1 in, 1 out]
            n82 = property on="FrozenFractionGraph" class="WFGraph (strict)"() -> ("Cursor.Cursor X"=w176:dbl)  [unwired: 2 in, 2 out]
            n83 = local read "maxSize"() -> (w174:i32)
            n84 = In Range and Coerce(upper limit=w174, x=w176, lower limit=0) -> (coerced(x)=w173:dbl)  [unwired: 1 out]
            n85 = local write "ImageIdx"(w173) -> ()
            n86 = call <vilib>:"Add State(s) to Queue__JKI_lib_State_Machine.vi"("State(s) in Front (\"\")"="Image: Set Cursors\nData: Set Image\nData: Show Img\nData: Update Well Temp", "State(s) in (\"\")"=w181) -> ("States Out"=w180:string)  [unwired: 13 in]
          }
          event "Fraction Single": Cursor Move {
            n87 = event-data() -> ()  [unwired: 1 in, 1 out]
            n88 = property on="Fraction Single" class="WFGraph (strict)"() -> ("Cursor.Cursor X"=w185:dbl)  [unwired: 2 in, 2 out]
            n89 = local read "maxSize"() -> (w183:i32)
            n90 = In Range and Coerce(upper limit=w183, x=w185, lower limit=0) -> (coerced(x)=w184:dbl)  [unwired: 1 out]
            n91 = local write "ImageIdx"(w184) -> ()
            n92 = call <vilib>:"Add State(s) to Queue__JKI_lib_State_Machine.vi"("State(s) in Front (\"\")"="Image: Set Cursors\nData: Set Image\nData: Show Img\nData: Update Well Temp", "State(s) in (\"\")"=w190) -> ("States Out"=w189:string)  [unwired: 13 in]
          }
          event "Temps grads": Cursor Move {
            n93 = event-data() -> ()  [unwired: 1 in, 9 out]
            n94 = property on="Temps grads" class="WFGraph (strict)"() -> ("Cursor.Cursor X"=w194:dbl)  [unwired: 2 in, 2 out]
            n95 = local read "maxSize"() -> (w193:i32)
            n96 = In Range and Coerce(upper limit=w193, x=w194, lower limit=0) -> (coerced(x)=w191:dbl)  [unwired: 1 out]
            n97 = local write "ImageIdx"(w191) -> ()
            n98 = call <vilib>:"Add State(s) to Queue__JKI_lib_State_Machine.vi"("State(s) in Front (\"\")"="Image: Set Cursors\nData: Set Image\nData: Show Img\nData: Update Well Temp", "State(s) in (\"\")"=w199) -> ("States Out"=w198:string)  [unwired: 13 in]
          }
          event "Calc_All": Value Change {
            w200 = FALSE ("Visible")
            w204 = u8 0 ("Slide")
            n99 = event-data() -> ()  [unwired: 1 in, 6 out]
            n100 = local write "ImageIdx"(w204) -> ()
            n101 = local write "img"(0 ("img")) -> ()
            n102 = local write "Slide"(w204) -> ()
            n103 = property on="Temps" class="WFGraph (strict)"("Visible"=TRUE) -> ()  [unwired: 2 in, 2 out]
            n104 = property on="Temps single" class="WFGraph (strict)"("Visible"=w200) -> ()  [unwired: 2 in, 2 out]
            n105 = property on="Temps single grad" class="WFGraph (strict)"("Visible"=w200) -> ()  [unwired: 2 in, 2 out]
            n106 = property on="Temp grads" class="WFGraph (strict)"("Visible"=w200) -> ()  [unwired: 2 in, 2 out]
            n107 = local write "Offset Applied?"(FALSE ("Offset Applied?")) -> ()
            n108 = call <vilib>:"Add State(s) to Queue__JKI_lib_State_Machine.vi"("State(s) in Front (\"\")"="Process: Calculate All", "State(s) in (\"\")"=w209) -> ("States Out"=w208:string)  [unwired: 13 in]
          }
          event "Correct Data": Value Change {
            n109 = event-data() -> ()  [unwired: 1 in, 6 out]
            n110 = property on="Correct Data" class="Bool"("Visible"=FALSE) -> ()  [unwired: 2 in, 2 out]
            n111 = property on="Remove_Correction" class="Bool"("Visible"=TRUE) -> ()  [unwired: 2 in, 2 out]
            n112 = call <vilib>:"Add State(s) to Queue__JKI_lib_State_Machine.vi"("State(s) in Front (\"\")"="UI: Cursor Set >> Busy\nUI: Tutorial >> Correcting Data\nProcess: Correct Offset\nProcess: Recalculate\nOverlay: Update Focus Well\nUI: Tutorial >> Done\nUI: Cursor Set >> Idle", "State(s) in (\"\")"=w217) -> ("States Out"=w216:string)  [unwired: 13 in]
            "Offset Applied?" <- TRUE ("Offset Applied?")
          }
          event "Remove_Correction": Value Change {
            n113 = event-data() -> ()  [unwired: 1 in, 6 out]
            n114 = property on="Remove_Correction" class="Bool"("Visible"=FALSE) -> ()  [unwired: 2 in, 2 out]
            n115 = property on="Correct Data" class="Bool"("Visible"=TRUE) -> ()  [unwired: 2 in, 2 out]
            n116 = local write "Offset Applied?"(FALSE ("Offset Applied?")) -> ()
            n117 = call <vilib>:"Add State(s) to Queue__JKI_lib_State_Machine.vi"("State(s) in Front (\"\")"="UI: Cursor Set >> Busy\nUI: Tutorial >> Correcting Data\nProcess: Remove Offset\nProcess: Recalculate\nOverlay: Update Focus Well\nUI: Tutorial >> Done\nUI: Cursor Set >> Idle", "State(s) in (\"\")"=w225) -> ("States Out"=w224:string)  [unwired: 13 in]
          }
        }
      }
      frame "---------- Core ----------" {
        # "Do not put any code in this frame.\n(it is a separator no-op)"
        n118 = call <vilib>:"Add State(s) to Queue__JKI_lib_State_Machine.vi"("State(s) in (\"\")"=w229) -> ("States Out"=w228:string)  [unwired: 14 in]
      }
      frame Default {
        w239 = 42 items=["No error", "Argument error", "Memory is full", "Out of zone", "End of file", "File already open", "Generic file I/O error", "File not found", "File permission error", "Disk is full", "Duplicate path", "Too many files open", "System feature not enabled", "Resource file not found", "Cannot add resource", "Resource not found", "Image not found", "Image memory error", "Pen does not exist", "Config type invalid", "Config token not found", "Config parse error", "Config memory error", "Bad external code format", "Bad external code offset", "External code not present", "Null window", "Destroy window error", "Null menu", "Print aborted", "Bad print record", "Print driver error", "Windows error during printing", "Memory error during printing", "Print dialog error", "Generic print error", "Invalid device refnum", "Device not found", "Device parameter error", "Device unit error", "Cannot open device", "Device call aborted", "Generic error", "Cancelled by user", "Object ID too low", "Object ID too high", "Object not in heap", "Unknown heap", "Unknown object (invalid DefProc)", "Unknown object (DefProc not in table)", "Message out of range", "Invalid (null) method", "Unknown message", "Manager call not supported", "Bad address", "Network operation in progress", "Network operation timed out", "Connection is busy", "Network attribute not supported", "Network error", "Address in use", "System out of memory", "Connection aborted", "Connection refused", "Not connected", "Already connected", "Connection closed", "Initialization error (interapplication manager)", "Bad occurrence", "Wait on unbound occurrence handler", "Occurrence queue overflow", "Datalog type conflict", "Unused", "Unrecognized type (interapplication manager)", "Memory corrupt", "Failed to make temporary DLL", "Old CIN version", "Drag socket not found", "Failed to load drop-object", "Failed to register OLE object", "Failed to release OLE object", "Format specifier type mismatch", "Unknown format specifier", "Too few format specifiers", "Too many format specifiers", "Scan failed", "Newer CIN version", "Error converting to variant", "Runtime menu error", "Password tampered", "Variant attribute not found", "Incompatible variant data type", "Event data is not available", "Event Store is not present", "Occurrence is not found", "Event Queue is not created", "Event info is not available", "Refnum passed is NULL", "Error retrieving Class GUID", "Error retrieving CoClass GUID", "Error retrieving TypeLib GUID.", "Bad built application magic bytes.", "Specific driver is different from the specific driver associated with the Logical Name.", "There is no session opened to the class driver.", "Max Error", "MAX - Error with config objects", "MAX - Error loading configuration", "MAX - Group not supported"]
        # "Current State"
        # "Do not delete, rename, or modify this frame.\n(this is used to capture unhandled states and typos)"
        # "Handle mistyped state name (developer tool)"
        n119 = Format Into String(format string="Software Exception: Unhandled State \"%s\"." ("message"), error in=w235, w230) -> (resulting string=w238:string, error out=w237:errorcluster)  [unwired: 1 in]
        n120 = call <vilib>:"Error Cluster From Error Code.vi"("show call chain? (False)"=TRUE, "error in (no error)"=w237, "error message (\"\")"=w238, "error code (0)"=w239) -> ("error out"=w236:errorcluster)  [unwired: 5 in]
        n121 = call <vilib>:"Add State(s) to Queue__JKI_lib_State_Machine.vi"("State(s) in (\"\")"=w234) -> ("States Out"=w233:string)  [unwired: 14 in]
      }
      frame "Initialize Core Data" {
        # "Do not delete, rename, or modify this frame.\n(this is used to determine panel behavior on exit)"
        # "originally closed?"
        # "exe?"
        # "If panel starts closed or is an EXE, then close it when we exit"
        n122 = property class="App"() -> ("App.Kind"=w249:T6)  [unwired: 2 in, 2 out]
        n123 = control-ref of="Current VI Reference"() -> (w244:refnum<vi>)
        n124 = property class="VI"() -> ("FP.State"=w243:T5)  [unwired: 2 in, 2 out]
        n125 = Equal?(x=w243, y=T5."Closed" ("Front Panel Window:State")) -> (x = y?=w241:bool)
        n126 = Equal?(x=w249, y=T6."Run Time System" ("Application:Kind")) -> (x = y?=w247:bool)
        n127 = Or(x=w241, y=w247) -> (x .or. y?=w245:bool)
        n128 = Bundle By Name(cluster=w246, "Core.Current VI Reference"=w244, "Core.Close Panel on Exit?"=w245) -> (w251:T4)
        n129 = call <vilib>:"Add State(s) to Queue__JKI_lib_State_Machine.vi"("State(s) in (\"\")"=w253) -> ("States Out"=w252:string)  [unwired: 14 in]
      }
      frame "Error Handler" {
        # "Unhandled Error -- Display it"
        # "Handle any errors here.\nYou can also output any states to clean-up after errors occur"
        # "Clear error"
        n130 = call <vilib>:"General Error Handler.vi"("error in (no error)"=w255) -> ()  [unwired: 10 in, 5 out]
        n131 = call <vilib>:"Add State(s) to Queue__JKI_lib_State_Machine.vi"("State(s) in Front (\"\")"="/* Post Error States", "State(s) in (\"\")"=w259) -> ("States Out"=w258:string)  [unwired: 13 in]
      }
      frame "Exit" {
        # "Do not put any code in this frame.\n(No errors that occur here will be handled.)"
        n132 = call <vilib>:"Add State(s) to Queue__JKI_lib_State_Machine.vi"("State(s) in (\"\")"=w264) -> ("States Out"=w263:string)  [unwired: 14 in]
      }
      frame "---------- Data ----------" {
        # "Do not put any code in this frame.\n(It is a separator no-op. You can make a copy of this frame to create a new Data frame)"
        n133 = call <vilib>:"Add State(s) to Queue__JKI_lib_State_Machine.vi"("State(s) in (\"\")"=w268) -> ("States Out"=w267:string)  [unwired: 14 in]
      }
      frame "Data: Initialize" {
        w273 = dbl[] [] ("Offsets")
        w275 = dbl[][] []  # Temps_Array
        w276 = dbl[] []  # Temps
        w279 = T1[] []  # img_array
        w281 = u32 1 items=["Zoom Tool"=8, "Selection Tool"=0, "Pan Tool"=9, "Point Tool"=1, "Line Tool"=2, "Rectangle Tool"=3, "Rotated Rectangle Tool"=12, "Polyline Tool"=10, "Polygon Tool"=5, "Freehand Tool"=11, "Closed Freehand Tool"=6, "Ellipse Tool"=4, "Annulus Tool"=7] ("Current ROI Tool")
        w278 = 0  # State
        w282 = T11 {"Current VI Reference"=refnum, "Close Panel on Exit?"=FALSE}  # Core
        # "Initialize the shift-register data, here.\n(data names are defined by what you wire into the bundle function)"
        n134 = property on="Image" class="ImageControl"("Current ROI Tool"=w281) -> ()  [unwired: 2 in, 2 out]
        n135 = local write "Offsets"(w273) -> ()
        n136 = local write "FreezeFract Concatinated"(w273) -> ()
        n137 = local write "ThermTemps"(w273) -> ()
        n138 = local write "Slide"(w278) -> ()
        n139 = call "TCE_Config_Load.vi"() -> ("error out"=w270:errorcluster, "Config"=w272:T3)  [unwired: 10 in]
        n140 = call "TCE_Config_Save.vi"("error in"=w270, "Config"=w272) -> ("Config dup"=w271:T3)  [unwired: 8 in, 1 out]
        n141 = Bundle By Name(cluster=T4 {"Core"={"Current VI Reference"=refnum, "Close Panel on Exit?"=FALSE}, "Image Out"=refnum, "State"=0, "Points"={"Top Left"={"X"=0.0, "Y"=0.0}, "Top Right"={"X"=0.0, "Y"=0.0}, "Bottom Left"={"X"=0.0, "Y"=0.0}, "Bottom Right"={"X"=0.0, "Y"=0.0}, "x space 2"=0.0, "y space 2"=0.0, "x_space"=0.0, "y_space"=0.0, "Pixels"=[], "Fixpoint"={"X"=0.0, "Y"=0.0}}, "img_array"=[], "Temps"=[], "Temps_Array"=[], "Scan Area"=0.0, "Fixpoint Area"=0.0, "Config"={"Freezing"={"Cutoff"=2.0, "EndIndex"=2}}, "PCR Size"=0, "ImageCount"=0, "ShowGradient"=FALSE} ("Cluster"), "Core"=w282, "Image Out"=T1 refnum, "State"=w278, "img_array"=w279, "Temps"=w276, "Temps_Array"=w275, "Config"=w271, "ShowGradient"=FALSE) -> (w283:T4)
        n142 = call <vilib>:"Add State(s) to Queue__JKI_lib_State_Machine.vi"("State(s) in (\"\")"=w285) -> ("States Out"=w284:string)  [unwired: 14 in]
      }
      frame "Data: Cleanup" {
        # "Cleanup any data and references, here.\n(this is called automatically, by the Macro: Exit)"
        n143 = Unbundle By Name(w292) -> ("Config"=w286:T3, "img_array"=w290:T1[], "Image Out"=w289:T1)
        n144 = call "TCE_Config_Save.vi"("Config"=w286) -> ()  [unwired: 9 in, 2 out]
        n145 = call "IMAQ Dispose"("Image"=w289, "error in (no error)"=w288) -> ("error out"=w287:errorcluster)  [unwired: 4 in]
        n146 = for {
          shift-right: [w296] -> w291
          shift-left: w287 -> [w297]
          tunnel: w290 -> [w295] mode=indexing
          n147 = call "IMAQ Dispose"("Image"=w295, "error in (no error)"=w297) -> ("error out"=w296:errorcluster)  [unwired: 4 in]
        }
        n148 = call <vilib>:"Add State(s) to Queue__JKI_lib_State_Machine.vi"("State(s) in (\"\")"=w294) -> ("States Out"=w293:string)  [unwired: 14 in]
      }
      frame "Data: Config" {
        # "Do not put any code in this frame.\n(It is a separator no-op. You can make a copy of this frame to create a new Data frame)"
        n149 = call "TCE_Config.vi"("Cluster"=w299) -> ("Config out"=w298:T4)  [unwired: 9 in, 1 out]
        n150 = call <vilib>:"Add State(s) to Queue__JKI_lib_State_Machine.vi"("State(s) in (\"\")"=w302) -> ("States Out"=w301:string)  [unwired: 14 in]
      }
      frame "Data: Load Image" {
        # "Do not put any code in this frame.\n(It is a separator no-op. You can make a copy of this frame to create a new Data frame)"
        n151 = local write "img"(0 ("img")) -> ()
        n152 = local write "Slide"(u8 0 ("Slide")) -> ()
        n153 = Empty String/Path?(string/path="Path") -> (empty?=w313:bool)
        n154 = case shown="False" w313 {
          tunnel: [w334 _] -> w316
          tunnel: w315 -> [w331 w365]
          tunnel: [w335 w365] -> w309
          tunnel: "Path" -> [w323 _]
          tunnel: [w333 _] -> w311
          tunnel: w306 -> [w325 _]
          tunnel: [w320 0] -> w303
          frame False {
            n155 = Build Path(base path=w323, name or relative path=path "Images") -> (appended path=w326:path)
            n156 = List Folder(path=w326) -> (filenames=w321:string[])  [unwired: 3 in, 3 out]
            n157 = property on="Slide" class="Slide (strict)"(error in=w331, "Visible"=TRUE) -> (error out=w330:errorcluster)  [unwired: 1 in, 1 out]
            n158 = call "Partition_Extract.vi"("input cluster"=w325, "Path"=w323) -> ("PartitionArray"=→"PartitionArray":string[])
            n159 = call "Thermistor_Extract.vi"("Path"=w323, "filenames"=w321) -> ("ThermTemps"=→"ThermTemps":dbl[])
            n160 = Array Size(array=w321) -> (size(s)=w329:i32)
            n161 = Format Into String(w329) -> (resulting string=w328:string)  [unwired: 3 in, 1 out]
            n162 = for {
              tunnel: [w363] -> w337
              tunnel: [w347] -> w333 mode=indexing
              tunnel: [w350] -> _ mode=indexing
              tunnel: w321 -> [w355] mode=indexing
              tunnel: w326 -> [w354]
              tunnel: w329 -> [w349]
              tunnel: w330 -> [w350]
              workers-P: _ -> [_]
              tunnel: w328 -> [w339]
              i -> [w348]
              w358 = T12 7 items=["Grayscale (U8)", "Grayscale (I16)", "Grayscale (SGL)", "Complex (CSG)", "RGB (U32)", "HSL (U32)", "RGB (U64)", "Grayscale (U16)"] ("Image Type")
              n163 = Format Into String(w348) -> (resulting string=w356:string)  [unwired: 3 in, 1 out]
              n164 = local read "img"() -> (w346:i32)
              n165 = Concatenate Strings("img_" ("Image Name"), w356) -> (w357:string)
              n166 = Build Path(base path=w354, name or relative path=w355) -> (appended path=w353:path)
              n167 = Increment(x=w346) -> (x+1=w340:i32)
              n168 = call "IMAQ Create"("Image Name"=w357, "Image Type"=w358, "error in (no error)"=w350) -> ("New Image"=w361:T1, "error out"=w362:errorcluster)  [unwired: 2 in]
              n169 = Format Into String(w340) -> (resulting string=w343:string)  [unwired: 3 in, 1 out]
              n170 = local write "img"(w340) -> ()
              n171 = call "IMAQ ReadFile 2"("File Path"=w353, "error in (no error)"=w362, "Image"=w361) -> ("error out"=w360:errorcluster, "Image Out"=w338:T1)  [unwired: 4 in, 3 out]
              n172 = Divide(x=w340, y=w349) -> (x/y=w352:dbl)
              n173 = Concatenate Strings("Loading image " ("Tutorial"), w343, " of " ("Tutorial"), w339) -> (w344:string)
              n174 = Multiply(x=w352, y=100.0) -> (x*y=→"Slide":dbl)
              n175 = local write "Tutorial"(w344) -> ()
              n176 = call "IMAQ Clear Overlay"("error in (no error)"=w360, "Image"=w338) -> ("error out"=w363:errorcluster, "Image Out"=w347:T1)  [unwired: 8 in]
              n177 = local write "Image"(w347) -> ()
            }
            n178 = Decrement(x=w329) -> (x-1=w320:i32)
            "maxSize" <- w320
            n179 = Index Array(array=w333) -> (element=w334:T1)  [unwired: 1 in]
            "Image" <- w334
            n180 = property on="Image" class="ImageControl"(error in=w337, "ROI"=T7 {"Global Rectangle"=[], "Contours"=[]}) -> (error out=w335:errorcluster)  [unwired: 1 in, 1 out]
          }
          frame True {
            (unwired) FALSE ("Visible")
          }
        }
        n181 = property on="Slide" class="Slide (strict)"(error in=w309, "Visible"=FALSE) -> (error out=w308:errorcluster)  [unwired: 1 in, 1 out]
        n182 = Bundle By Name(cluster=w306, "Image Out"=w316, "img_array"=w311, "Config.Freezing.EndIndex"=w303, "ImageCount"=w303) -> (w317:T4)
        n183 = local write "ImageIdx"(u32 0 ("Image")) -> ()
        n184 = call <vilib>:"Add State(s) to Queue__JKI_lib_State_Machine.vi"("State(s) in Front (\"\")"="Image: Set Cursors\nImage: Draw" ("State(s) in Front (\"\")"), "State(s) in (\"\")"=w319) -> ("States Out"=w318:string)  [unwired: 13 in]
      }
      frame "Data: Load Results" {
        # "Do not put any code in this frame.\n(It is a separator no-op. You can make a copy of this frame to create a new Data frame)"
        n185 = local read "Path"() -> (w368:path)
        n186 = Build Path(base path=w368, name or relative path=path "Data.TCE") -> (appended path=w369:path)
        n187 = call <vilib>:"Check if File or Folder Exists.vi"("path"=w369) -> ("file or folder exists?"=w371:bool, "dup path"=w370:path)  [unwired: 8 in, 1 out]
        n188 = case shown="True" w371 {
          tunnel: w370 -> [_ w385]
          tunnel: ["" ("State(s) in Front (\"\")") "UI: Single Temps >> Hide" ("State(s) in Front (\"\")")] -> w366
          frame False {
          }
          frame True {
            n189 = call-poly <vilib>:"Read Delimited Spreadsheet.vi"("file path (dialog if empty)"=w385, "delimiter (\\t)"=";" ("delimiter (\\t)")) -> ("all rows"=w384:string[][])  [unwired: 8 in, 5 out]
            n190 = call <vilib>:"Application Directory.vi"() -> ("Application Directory"=w387:path)
            n191 = Path To String(path=w385) -> (string=w392:string)
            n192 = call "DataArray_Reformatter.vi"("Data Array"=w384) -> ("MeltTemps"=w377:dbl[], "Offsets"=w380:dbl[], "FreezeTemps"=w383:dbl[], "Temps"=w382:dbl[][], "Offset Applied"=w379:bool)
            n193 = Build Path(base path=w387, name or relative path=path "TCEM.ini" ("file path (dialog if empty)")) -> (appended path=w388:path)
            n194 = Build Array(w392) -> (w391:string[])
            n195 = Not(x=w379) -> (.not. x?=w378:bool)
            n196 = local write "Offsets"(w380) -> ()
            n197 = local write "Offset Applied?"(w379) -> ()
            n198 = local write "MeltTemps"(w377) -> ()
            n199 = property on="Remove_Correction" class="Bool"("Visible"=w379) -> ()  [unwired: 2 in, 2 out]
            n200 = local write "Temps"(w382) -> ()
            n201 = local write "FreezeTemps"(w383) -> ()
            n202 = call-poly <vilib>:"Write Delimited Spreadsheet.vi"("file path (dialog if empty)"=w388, "1D data"=w391, "append to file? (new file:F)"=TRUE) -> ()  [unwired: 11 in, 2 out]
            n203 = property on="Correct Data" class="Bool"("Visible"=w378) -> ()  [unwired: 2 in, 2 out]
          }
        }
        n204 = call <vilib>:"Add State(s) to Queue__JKI_lib_State_Machine.vi"("State(s) in Front (\"\")"=w366, "State(s) in (\"\")"=w375) -> ("States Out"=w374:string)  [unwired: 13 in]
      }
      frame "Data: Load Calibration" {
        # "Do not put any code in this frame.\n(It is a separator no-op. You can make a copy of this frame to create a new Data frame)"
        n205 = local read "Path"() -> (w394:path)
        n206 = Build Path(base path=w394, name or relative path=path "TCC.cal") -> (appended path=w399:path)
        n207 = call <vilib>:"Check if File or Folder Exists.vi"("path"=w399) -> ("file or folder exists?"=w400:bool, "dup path"=w397:path)  [unwired: 8 in, 1 out]
        n208 = case shown="True" w400 {
          tunnel: w397 -> [_ w425]
          tunnel: w396 -> [w405 w424]
          tunnel: [w406 w423] -> w395
          tunnel: w394 -> [w409 _]
          tunnel: [w404 "Image: Draw\nData: Load Results\nData: Set Image\nProcess: Recalculate\nUI: Calc >> True\nUI: Menu Overlay Grid >> True\nUI: Menu Overlay Temps >> True\nUI: Progress >> Hide\nUI: Cursor Set >> Idle\nUI: Tutorial >> Click on a Well to show single or click outside the plate to show all."] -> w393
          frame False {
            n209 = call "CalibrationLoadPrompt.vi"("Root Path"=w409) -> ("cancel?"=w407:bool, "selected path"=w408:path)  [unwired: 9 in]
            n210 = case shown="False" w407 {
              tunnel: w408 -> [w413 _]
              tunnel: [w411 w418] -> w406
              tunnel: w405 -> [w412 w418]
              tunnel: ["Image: Draw\nData: Load Results\nData: Set Image\nProcess: Recalculate\nUI: Menu Overlay Grid >> True\nUI: Menu Overlay Temps >> True\nUI: Calc >> True\nUI: Progress >> Hide\nUI: Cursor Set >> Idle\nUI: Tutorial >> Click on a Well to show single or click outside the plate to show all." "UI: Calc >> Disable\nUI: Progress >> Hide\nUI: Cursor Set >> Idle\nUI: Tutorial >> Error: Missing Calibration File!"] -> w404
              frame False {
                n211 = call "TCam_Calibration_LoadSettings.vi"("path"=w413) -> ("Fixpoint Area"=w414:dbl, "Scan Area"=w415:dbl, "Points"=w416:T13)  [unwired: 7 in, 1 out]
                n212 = Bundle By Name(cluster=w412, "Points"=w416, "Scan Area"=w415, "Fixpoint Area"=w414) -> (w411:T4)
              }
              frame True {
              }
            }
          }
          frame True {
            n213 = call "TCam_Calibration_LoadSettings.vi"("path"=w425) -> ("Fixpoint Area"=w421:dbl, "Scan Area"=w422:dbl, "Points"=w419:T13)  [unwired: 7 in, 1 out]
            n214 = Bundle By Name(cluster=w424, "Points"=w419, "Scan Area"=w422, "Fixpoint Area"=w421) -> (w423:T4)
          }
        }
        n215 = call <vilib>:"Add State(s) to Queue__JKI_lib_State_Machine.vi"("State(s) in Front (\"\")"=w393, "State(s) in (\"\")"=w403) -> ("States Out"=w402:string)  [unwired: 13 in]
      }
      frame "Data: Set Image" {
        # "Do not put any code in this frame.\n(It is a separator no-op. You can make a copy of this frame to create a new Data frame)"
        n216 = Unbundle By Name(w430) -> ("img_array"=w429:T1[])
        n217 = Index Array(array=w429, index="ImageIdx") -> (element=w426:T1)
        n218 = Bundle By Name(cluster=w430, "Image Out"=w426) -> (w431:T4)
        n219 = call <vilib>:"Add State(s) to Queue__JKI_lib_State_Machine.vi"("State(s) in (\"\")"=w433) -> ("States Out"=w432:string)  [unwired: 14 in]
      }
      frame "Data: Show Img" {
        # "Do not put any code in this frame.\n(It is a separator no-op. You can make a copy of this frame to create a new Data frame)"
        n220 = Unbundle By Name(w434) -> ("Image Out"=w435:T1)
        n221 = local write "Image"(w435) -> ()
        n222 = call <vilib>:"Add State(s) to Queue__JKI_lib_State_Machine.vi"("State(s) in (\"\")"=w438) -> ("States Out"=w437:string)  [unwired: 14 in]
      }
      frame "Data: Update Well Temp" {
        # "Initialize the shift-register data, here.\n(data names are defined by what you wire into the bundle function)"
        n223 = local read "Temps single"() -> (w440:dbl[])
        n224 = local read "ImageIdx"() -> (w441:u32)
        n225 = Index Array(array=w440, index=w441) -> (element=w439:dbl)
        n226 = local write "CurTemp"(w439) -> ()
        n227 = call <vilib>:"Add State(s) to Queue__JKI_lib_State_Machine.vi"("State(s) in (\"\")"=w445) -> ("States Out"=w444:string)  [unwired: 14 in]
      }
      frame "Data: Temps Clear" {
        w446 = dbl[][] [] ("Temps_Array")
        w447 = dbl[] []  # Temps
        # "Initialize the shift-register data, here.\n(data names are defined by what you wire into the bundle function)"
        n228 = local write "Temps single"(w447) -> ()
        n229 = local write "Temps grads"(w446) -> ()
        n230 = local write "Temps"(w446) -> ()
        n231 = local write "Temps single grad"(w447) -> ()
        n232 = Bundle By Name(cluster=w449, "Temps"=w447, "Temps_Array"=w446) -> (w448:T4)
        n233 = call <vilib>:"Add State(s) to Queue__JKI_lib_State_Machine.vi"("State(s) in (\"\")"=w452) -> ("States Out"=w451:string)  [unwired: 14 in]
      }
      frame "Data: Save Results" {
        # "Initialize the shift-register data, here.\n(data names are defined by what you wire into the bundle function)"
        n234 = local read "FreezeFract Concatinated"() -> (w463:dbl[])
        n235 = local read "Offset Applied?"() -> (w459:bool)
        n236 = local read "PartitionArray"() -> (w461:string[])
        n237 = local read "FreezeTemps"() -> (w464:dbl[])
        n238 = local read "MeltTemps"() -> (w462:dbl[])
        n239 = local read "Offsets"() -> (w460:dbl[])
        n240 = local read "Temps"() -> (w465:dbl[][])
        n241 = call "TCE_SaveConfiguration.vi"("input cluster"=w466, "Temps"=w465, "FreezeTemps"=w464, "MeltTemps"=w462, "FrozenFraction"=w463, "PartitionArray"=w461, "Offsets"=w460, "Offset Applied?"=w459) -> ("Save Array out"=w457:string[][], "Full Array"=w456:string[][], "Canceled"=w455:bool)  [unwired: 9 in]
        n242 = case shown="False" w455 {
          tunnel: w453 -> [w483 w503]
          tunnel: w457 -> [w476 _]
          tunnel: [w475 "" ("State(s) in Front (\"\")")] -> w458
          tunnel: w456 -> [w471 _]
          tunnel: [w470 w503] -> w454
          frame False {
            n243 = local read "Path"() -> (w473:path)
            n244 = Build Path(base path=w473, name or relative path=path "Result Data.csv") -> (appended path=w478:path)
            n245 = Build Path(base path=w473, name or relative path=path "Data.TCE") -> (appended path=w472:path)
            n246 = call <vilib>:"Check if File or Folder Exists.vi"("path"=w478) -> ("file or folder exists?"=w481:bool, "dup path"=w477:path)  [unwired: 8 in, 1 out]
            n247 = case shown="False" w481 {
              selector: w481 -> [_ w489]
              tunnel: w473 -> [w487 _]
              tunnel: [w486 w488] -> w480
              tunnel: [w484 w489] -> w479
              tunnel: w477 -> [_ w488]
              frame False {
                n248 = call "ResultSavePrompt.vi"("Path"=w487) -> ("selected path"=w486:path, "cancel?"=w485:bool)
                n249 = Not(x=w485) -> (.not. x?=w484:bool)
              }
              frame True {
              }
            }
            n250 = case shown="True" w479 {
              tunnel: w476 -> [_ w501]
              tunnel: w483 -> [w490 w500]
              tunnel: w480 -> [_ w499]
              tunnel: ["" ("State(s) in Front (\"\")") "UI: Recent Menu Update" ("State(s) in Front (\"\")")] -> w475
              tunnel: w472 -> [_ w497]
              tunnel: w471 -> [_ w496]
              tunnel: [w490 w493] -> w470
              frame False {
              }
              frame True {
                w495 = ";" ("delimiter (\\t)")
                n251 = call-poly <vilib>:"Write Delimited Spreadsheet.vi"("file path (dialog if empty)"=w499, "2D data"=w501, "error in (no error)"=w500, "delimiter (\\t)"=w495) -> ("error out"=w494:errorcluster)  [unwired: 10 in, 1 out]
                n252 = call-poly <vilib>:"Write Delimited Spreadsheet.vi"("file path (dialog if empty)"=w497, "2D data"=w496, "error in (no error)"=w494, "delimiter (\\t)"=w495) -> ("new file path (Not A Path if cancelled)"=w492:path, "error out"=w493:errorcluster)  [unwired: 10 in]
                n253 = call "RunTimeMenu_TCE_RecentInsert.vi"("NewPath"=w492) -> ()  [unwired: 11 in]
              }
            }
          }
          frame True {
          }
        }
        n254 = case shown="Error .." w454 {
          frame No Error {
          }
          frame Error {
            n255 = One Button Dialog(message="File Save Error!\nClose file if open.") -> ()  [unwired: 1 in, 1 out]
          }
        }
        n256 = call <vilib>:"Add State(s) to Queue__JKI_lib_State_Machine.vi"("State(s) in Front (\"\")"=w458, "State(s) in (\"\")"=w468) -> ("States Out"=w467:string)  [unwired: 13 in]
      }
      frame "Data: Save Results As" {
        # "Initialize the shift-register data, here.\n(data names are defined by what you wire into the bundle function)"
        n257 = local read "FreezeFract Concatinated"() -> (w515:dbl[])
        n258 = local read "Offset Applied?"() -> (w511:bool)
        n259 = local read "PartitionArray"() -> (w513:string[])
        n260 = local read "FreezeTemps"() -> (w516:dbl[])
        n261 = local read "MeltTemps"() -> (w514:dbl[])
        n262 = local read "Offsets"() -> (w512:dbl[])
        n263 = local read "Temps"() -> (w517:dbl[][])
        n264 = call "TCE_SaveConfiguration.vi"("input cluster"=w510, "Temps"=w517, "FreezeTemps"=w516, "MeltTemps"=w514, "FrozenFraction"=w515, "PartitionArray"=w513, "Offsets"=w512, "Offset Applied?"=w511) -> ("Save Array out"=w509:string[][], "Full Array"=w506:string[][], "Canceled"=w507:bool)  [unwired: 9 in]
        n265 = case shown="False" w507 {
          tunnel: w504 -> [w528 w543]
          tunnel: w509 -> [w525 _]
          tunnel: [w524 "" ("State(s) in Front (\"\")")] -> w508
          tunnel: [w522 w543] -> w505
          tunnel: w506 -> [w521 _]
          frame False {
            n266 = local read "Path"() -> (w523:path)
            n267 = call "ResultSavePrompt.vi"("Path"=w523) -> ("selected path"=w527:path, "cancel?"=w526:bool)
            n268 = case shown="False" w526 {
              tunnel: w525 -> [w540 _]
              tunnel: w528 -> [w539 w541]
              tunnel: w527 -> [w538 _]
              tunnel: ["UI: Recent Menu Update" ("State(s) in Front (\"\")") "" ("State(s) in Front (\"\")")] -> w524
              tunnel: w523 -> [w536 _]
              tunnel: [w532 w541] -> w522
              tunnel: w521 -> [w531 _]
              frame False {
                w530 = ";" ("delimiter (\\t)")
                n269 = call-poly <vilib>:"Write Delimited Spreadsheet.vi"("file path (dialog if empty)"=w538, "2D data"=w540, "error in (no error)"=w539, "delimiter (\\t)"=w530) -> ("error out"=w533:errorcluster)  [unwired: 10 in, 1 out]
                n270 = Build Path(base path=w536, name or relative path=path "Data.TCE") -> (appended path=w534:path)
                n271 = call-poly <vilib>:"Write Delimited Spreadsheet.vi"("file path (dialog if empty)"=w534, "2D data"=w531, "error in (no error)"=w533, "delimiter (\\t)"=w530) -> ("new file path (Not A Path if cancelled)"=w529:path, "error out"=w532:errorcluster)  [unwired: 10 in]
                n272 = call "RunTimeMenu_TCE_RecentInsert.vi"("NewPath"=w529) -> ()  [unwired: 11 in]
              }
              frame True {
              }
            }
          }
          frame True {
          }
        }
        n273 = case shown="Error .." w505 {
          frame No Error {
          }
          frame Error {
            n274 = One Button Dialog(message="File Save Error!\nClose file if open.") -> ()  [unwired: 1 in, 1 out]
          }
        }
        n275 = call <vilib>:"Add State(s) to Queue__JKI_lib_State_Machine.vi"("State(s) in Front (\"\")"=w508, "State(s) in (\"\")"=w519) -> ("States Out"=w518:string)  [unwired: 13 in]
      }
      frame "---------- UI ----------" {
        # "Do not put any code in this frame.\n(It is a separator no-op. You can make a copy of this frame to create a new UI frame)"
        n276 = call <vilib>:"Add State(s) to Queue__JKI_lib_State_Machine.vi"("State(s) in (\"\")"=w548) -> ("States Out"=w547:string)  [unwired: 14 in]
      }
      frame "UI: Initialize" {
        w557 = FALSE ("Visible")
        w568 = T12 4 items=["Grayscale (U8)", "Grayscale (I16)", "Grayscale (SGL)", "Complex (CSG)", "RGB (U32)", "HSL (U32)", "RGB (U64)", "Grayscale (U16)"] ("Image Type")
        w549 = FALSE ("Visible")
        w556 = TRUE ("Zoom to Fit Mode")
        w553 = 0.0 ("X Scale.Range:Minimum")
        w555 = dbl[] []
        w552 = 0.0 ("Cursor.Cursor Position:Cursor X")
        w554 = dbl[][] []
        # "Initialize the User Interface, here.\n(this is called automatically, by the Macro: Init)"
        n277 = property on="Temps grads" class="WFGraph (strict)"("Visible"=w557) -> ()  [unwired: 2 in, 2 out]
        n278 = property on="Temps single grad" class="WFGraph (strict)"("Visible"=w557) -> ()  [unwired: 2 in, 2 out]
        n279 = control-ref of="Splitter 4"() -> (w559:refnum<vi>)
        n280 = local write "Offset Applied?"(FALSE ("Offset Applied?")) -> ()
        n281 = property on="FrozenFractionGraph" class="WFGraph (strict)"("Active Plot"=u32 0, "Legend Visible"=FALSE ("Legend:Visible")) -> ()  [unwired: 2 in, 2 out]
        n282 = property on="Image" class="ImageControl"("Zoom to Fit Mode"=w556) -> ()  [unwired: 2 in, 2 out]
        n283 = property on="FrozenFractionGraph" class="WFGraph (strict)"("Visible"=w556) -> ()  [unwired: 2 in, 2 out]
        n284 = property on="Temps" class="WFGraph (strict)"("XScale.Minimum"=w553) -> ()  [unwired: 2 in, 2 out]
        n285 = property on="FrozenFractionGraph" class="WFGraph (strict)"("XScale.Minimum"=w553) -> ()  [unwired: 2 in, 2 out]
        n286 = call "ShowHideSplit.vi"("Splitter in"=w559, "Show Split"=w549) -> ()  [unwired: 1 in]
        n287 = property on="Contents" class="Str"("Visible"=w549) -> ()  [unwired: 2 in, 2 out]
        n288 = property on="Calc_All" class="Bool"("Visible"=w549) -> ()  [unwired: 2 in, 2 out]
        n289 = property on="CurTemp" class="DigNum (strict)"("Visible"=FALSE) -> ()  [unwired: 2 in, 2 out]
        n290 = property on="Fraction Single" class="WFGraph (strict)"("Visible"=w549) -> ()  [unwired: 2 in, 2 out]
        n291 = call <vilib>:"Application Directory.vi"() -> ("Application Directory"=w572:path)
        n292 = property on="Well" class="Str"("Visible"=w549) -> ()  [unwired: 2 in, 2 out]
        n293 = call "Read Exe Version.vi"("Application name"=path "TCE.exe") -> ("FileVersion"=w564:string)  [unwired: 7 in, 3 out]
        n294 = Path To String(path=w572) -> (string=w574:string)
        n295 = Concatenate Strings("version " ("string"), w564) -> (→"version":string)
        n296 = property on="Remove_Correction" class="Bool"("Visible"=w549) -> ()  [unwired: 2 in, 2 out]
        n297 = property on="Correct Data" class="Bool"("Visible"=w549) -> ()  [unwired: 2 in, 2 out]
        n298 = call "IMAQ Create"("Image Name"="placeholder_img_TCE", "Image Type"=w568) -> ("New Image"=w571:T1)  [unwired: 3 in, 1 out]
        n299 = Concatenate Strings(w574, "\\camera_placeholder.png") -> (w573:string)
        n300 = String To Path(string=w573) -> (path=w575:path)
        n301 = call "IMAQ ReadFile 2"("Use File Path Image Type"=FALSE, "File Path"=w575, "Image"=w571) -> ("Image Out"=w566:T1)  [unwired: 4 in, 4 out]
        "placeholder image" <- w566
        n302 = local write "FrozenFractionGraph"(w554) -> ()
        n303 = local write "Temps"(w554) -> ()
        n304 = local write "Temps single grad"(w555) -> ()
        n305 = local write "Temps grads"(w554) -> ()
        n306 = local write "Image"(w566) -> ()
        n307 = local write "Path"(path "" ("Path")) -> ()
        n308 = local write "Temps single"(w555) -> ()
        n309 = property on="Temps single" class="WFGraph (strict)"("Cursor.Cursor X"=w552) -> ()  [unwired: 2 in, 2 out]
        n310 = property on="Temps" class="WFGraph (strict)"("Cursor.Cursor X"=w552) -> ()  [unwired: 2 in, 2 out]
        n311 = property on="Temps grads" class="WFGraph (strict)"("Cursor.Cursor X"=w552) -> ()  [unwired: 2 in, 2 out]
        n312 = property on="Temps single grad" class="WFGraph (strict)"("Cursor.Cursor X"=w552) -> ()  [unwired: 2 in, 2 out]
        n313 = property on="FrozenFractionGraph" class="WFGraph (strict)"("Cursor.Cursor X"=w552) -> ()  [unwired: 2 in, 2 out]
        n314 = call <vilib>:"Add State(s) to Queue__JKI_lib_State_Machine.vi"("State(s) in Front (\"\")"="UI: Tutorial\nUI: Recent Menu Update\nUI: Progress >> Hide\nUI: Menu Save >> Hide\nUI: Menu Overlay Grid >> Hide\nUI: Menu Overlay Temps >> Hide" ("State(s) in Front (\"\")"), "State(s) in (\"\")"=w583) -> ("States Out"=w582:string)  [unwired: 13 in]
        "img" <- 0
        "Title" <- "Thermal Camera Evaluation" ("Title")
        "Title 2" <- "Well Data" ("Title 2")
      }
      frame "UI: Progress" {
        # "Initialize the User Interface, here.\n(this is called automatically, by the Macro: Init)"
        n315 = case shown="\"Show\"" w587 {
          tunnel: [FALSE ("Visible") TRUE ("Visible")] -> w586
          frame "Hide", Default {
          }
          frame "Show" {
          }
        }
        n316 = local write "img"(0 ("img")) -> ()
        n317 = local write "Slide"(u8 0 ("Slide")) -> ()
        n318 = property on="Slide" class="Slide (strict)"("Visible"=w586) -> ()  [unwired: 2 in, 2 out]
        n319 = call <vilib>:"Add State(s) to Queue__JKI_lib_State_Machine.vi"("State(s) in (\"\")"=w591) -> ("States Out"=w590:string)  [unwired: 14 in]
      }
      frame "UI: Recent Menu Update" {
        # "Initialize the User Interface, here.\n(this is called automatically, by the Macro: Init)"
        n320 = Current VI's Menubar() -> (w595:refnum<k9>)
        n321 = call "RunTimeMenu_Initialize_TCE.vi"("Menu in"=w595) -> ("paths"=→"recentPaths":path[])  [unwired: 9 in, 1 out]
        n322 = call <vilib>:"Add State(s) to Queue__JKI_lib_State_Machine.vi"("State(s) in (\"\")"=w599) -> ("States Out"=w598:string)  [unwired: 14 in]
      }
      frame "UI: Show First Image" {
        w600 = 0.0 ("Cursor.Cursor Position:Cursor X")
        # "Initialize the User Interface, here.\n(this is called automatically, by the Macro: Init)"
        n323 = Unbundle By Name(w603) -> ("img_array"=w602:T1[])
        n324 = property on="Temps" class="WFGraph (strict)"("Cursor.Cursor X"=w600) -> ()  [unwired: 2 in, 2 out]
        n325 = property on="Temps grads" class="WFGraph (strict)"("Cursor.Cursor X"=w600) -> ()  [unwired: 2 in, 2 out]
        n326 = property on="Temps single grad" class="WFGraph (strict)"("Cursor.Cursor X"=w600) -> ()  [unwired: 2 in, 2 out]
        n327 = property on="Temps single" class="WFGraph (strict)"("Cursor.Cursor X"=w600) -> ()  [unwired: 2 in, 2 out]
        n328 = property on="FrozenFractionGraph" class="WFGraph (strict)"("Cursor.Cursor X"=w600) -> ()  [unwired: 2 in, 2 out]
        n329 = property on="Fraction Single" class="WFGraph (strict)"("Cursor.Cursor X"=w600) -> ()  [unwired: 2 in, 2 out]
        n330 = Index Array(array=w602) -> (element=w601:T1)  [unwired: 1 in]
        n331 = local write "Image"(w601) -> ()
        n332 = call <vilib>:"Add State(s) to Queue__JKI_lib_State_Machine.vi"("State(s) in (\"\")"=w606) -> ("States Out"=w605:string)  [unwired: 14 in]
      }
      frame "UI: Tutorial" {
        # "Initialize the User Interface, here.\n(this is called automatically, by the Macro: Init)"
        n333 = call <vilib>:"Add State(s) to Queue__JKI_lib_State_Machine.vi"("State(s) in (\"\")"=w611) -> ("States Out"=w610:string)  [unwired: 14 in]
        "Tutorial" <- w607
      }
      frame "UI: Calc" {
        # "Initialize the User Interface, here.\n(this is called automatically, by the Macro: Init)"
        n334 = case shown="\"Hidden\", \"Hide\"" w614 {
          tunnel: [T8."Disabled and Grayed Out" ("Disabled") T8."Disabled and Grayed Out" ("Disabled") T8."Enabled" ("Disabled")] -> w613
          tunnel: [TRUE FALSE TRUE] -> w612
          frame "Disable", "False", Default {
          }
          frame "Hidden", "Hide" {
          }
          frame "True" {
          }
        }
        n335 = property on="Calc_All" class="Bool"("DisabledEnum"=w613) -> ()  [unwired: 2 in, 2 out]
        n336 = property on="Calc_All" class="Bool"("Visible"=w612) -> ()  [unwired: 2 in, 2 out]
        n337 = call <vilib>:"Add State(s) to Queue__JKI_lib_State_Machine.vi"("State(s) in (\"\")"=w618) -> ("States Out"=w617:string)  [unwired: 14 in]
      }
      frame "UI: Cursor Set" {
        # "Argument"
        # "Set and Unset Cursor Busy.\n(Usage: \"UI: Cursor Set >> Busy|Idle\")"
        n338 = case shown="\"Busy\"" w625 {
          tunnel: w627 -> [w632 w634]
          tunnel: [w631 w633] -> w626
          frame "Idle", Default {
            n339 = call <vilib>:"Unset Busy.vi"("error in (no error)"=w632) -> ("error out"=w631:errorcluster)  [unwired: 10 in]
          }
          frame "Busy" {
            n340 = call <vilib>:"Set Busy.vi"("error in (no error)"=w634) -> ("error out"=w633:errorcluster)  [unwired: 9 in, 1 out]
          }
        }
        n341 = call <vilib>:"Add State(s) to Queue__JKI_lib_State_Machine.vi"("State(s) in (\"\")"=w630) -> ("States Out"=w629:string)  [unwired: 14 in]
      }
      frame "UI: Menu Save" {
        # "Argument"
        # "Set and Unset Cursor Busy.\n(Usage: \"UI: Cursor Set >> Busy|Idle\")"
        n342 = case shown="\"Active\", \"Show\", \"True\"" w638 {
          tunnel: [FALSE TRUE] -> w636
          frame "Disable", "False", Default {
          }
          frame "Active", "Show", "True" {
          }
        }
        n343 = Current VI's Menubar() -> (w637:refnum<k9>)
        n344 = call "RunTimeMenu_Save_State_TCE.vi"("enabled"=w636, "item tag"=string[] ["DATA_SAVE", "DATA_SAVE_AS"], "Menu in"=w637) -> ()  [unwired: 8 in, 1 out]
        n345 = call <vilib>:"Add State(s) to Queue__JKI_lib_State_Machine.vi"("State(s) in (\"\")"=w642) -> ("States Out"=w641:string)  [unwired: 14 in]
      }
      frame "UI: Menu Overlay Grid" {
        # "Argument"
        # "Set and Unset Cursor Busy.\n(Usage: \"UI: Cursor Set >> Busy|Idle\")"
        n346 = case shown="\"Active\", \"Show\", \"True\"" w648 {
          tunnel: [FALSE TRUE] -> w646
          frame "Disable", "False", Default {
          }
          frame "Active", "Show", "True" {
          }
        }
        n347 = Current VI's Menubar() -> (w647:refnum<k9>)
        n348 = call "RunTimeMenu_Save_State_TCE.vi"("enabled"=w646, "item tag"=string[] ["OVERLAY_GRID", "OVERLAY_CLEAR"], "Menu in"=w647) -> ()  [unwired: 8 in, 1 out]
        n349 = call <vilib>:"Add State(s) to Queue__JKI_lib_State_Machine.vi"("State(s) in (\"\")"=w652) -> ("States Out"=w651:string)  [unwired: 14 in]
      }
      frame "UI: Menu Overlay Temps" {
        # "Argument"
        # "Set and Unset Cursor Busy.\n(Usage: \"UI: Cursor Set >> Busy|Idle\")"
        n350 = case shown="\"Active\", \"Show\", \"True\"" w658 {
          tunnel: [FALSE TRUE] -> w656
          frame "Disable", "False", Default {
          }
          frame "Active", "Show", "True" {
          }
        }
        n351 = Current VI's Menubar() -> (w657:refnum<k9>)
        n352 = call "RunTimeMenu_Save_State_TCE.vi"("enabled"=w656, "item tag"=string[] ["OVERLAY_TEMPS", "OVERLAY_FREEZE"], "Menu in"=w657) -> ()  [unwired: 8 in, 1 out]
        n353 = call <vilib>:"Add State(s) to Queue__JKI_lib_State_Machine.vi"("State(s) in (\"\")"=w662) -> ("States Out"=w661:string)  [unwired: 14 in]
      }
      frame "UI: Single Temps" {
        # "Argument"
        # "Set and Unset Cursor Busy.\n(Usage: \"UI: Cursor Set >> Busy|Idle\")"
        n354 = control-ref of="Splitter 4"() -> (w673:refnum<vi>)
        n355 = Unbundle By Name(w671) -> ("ShowGradient"=w670:bool)
        n356 = case shown="\"Disable\", \"False\", Default" w674 {
          tunnel: [w684 w687] -> w667
          tunnel: w673 -> [w685 w686]
          frame "Disable", "False", Default {
            w684 = FALSE
            n357 = call "ShowHideSplit.vi"("Splitter in"=w685, "Show Split"=w684) -> ()  [unwired: 1 in]
          }
          frame "Active", "Show", "True" {
            w687 = TRUE
            n358 = call "ShowHideSplit.vi"("Splitter in"=w686, "Show Split"=w687) -> ()  [unwired: 1 in]
          }
        }
        n359 = case shown="False" w670 {
          tunnel: [w680 w683] -> w669
          tunnel: [w679 w683] -> w668
          tunnel: [w678 w682] -> w666
          tunnel: w667 -> [w680 w682]
          tunnel: [w678 w681] -> w665
          frame False {
            w678 = FALSE
            n360 = Not(x=w680) -> (.not. x?=w679:bool)
          }
          frame True {
            w683 = FALSE
            n361 = Not(x=w682) -> (.not. x?=w681:bool)
          }
        }
        n362 = Not(x=w667) -> (.not. x?=w672:bool)
        n363 = property on="Temps single" class="WFGraph (strict)"("Visible"=w667) -> ()  [unwired: 2 in, 2 out]
        n364 = property on="Temps" class="WFGraph (strict)"("Visible"=w672) -> ()  [unwired: 2 in, 2 out]
        n365 = property on="Fraction Single" class="WFGraph (strict)"("Visible"=w669) -> ()  [unwired: 2 in, 2 out]
        n366 = property on="FrozenFractionGraph" class="WFGraph (strict)"("Visible"=w668) -> ()  [unwired: 2 in, 2 out]
        n367 = property on="Temps grads" class="WFGraph (strict)"("Visible"=w665) -> ()  [unwired: 2 in, 2 out]
        n368 = property on="Temps single grad" class="WFGraph (strict)"("Visible"=w666) -> ()  [unwired: 2 in, 2 out]
        n369 = property on="CurTemp" class="DigNum (strict)"("Visible"=w667) -> ()  [unwired: 2 in, 2 out]
        n370 = property on="Contents" class="Str"("Visible"=w667) -> ()  [unwired: 2 in, 2 out]
        n371 = property on="Well" class="Str"("Visible"=w667) -> ()  [unwired: 2 in, 2 out]
        n372 = call <vilib>:"Add State(s) to Queue__JKI_lib_State_Machine.vi"("State(s) in (\"\")"=w677) -> ("States Out"=w676:string)  [unwired: 14 in]
      }
      frame "UI: Front Panel State" {
        # "Argument"
        # "Set Front Panel Open or Closed\n(Usage: \"UI: Front Panel State >> Open|Close\")"
        n373 = Unbundle By Name(w690) -> ("Core.Current VI Reference"=w689:refnum<vi>)
        n374 = case shown="\"Minimize\", \"Minimized\"" w688 {
          tunnel: w692 -> [w700 w715 w726 w739 w752]
          tunnel: [w702 w716 w728 w741 w754] -> w691
          tunnel: w689 -> [w701 w713 w727 w740 w753]
          frame "Open", "Standard", Default {
            w695 = T5."Standard" ("State")
            n375 = property class="VI"(reference=w701, error in=w700) -> (reference out=w698:refnum<vi>, error out=w699:errorcluster, "FP.State"=w697:T5)
            n376 = Not Equal?(x=w697, y=w695) -> (x != y?=w696:bool)
            n377 = case shown="True" w696 {
              tunnel: [w706 w708] -> w702
              tunnel: w699 -> [w705 w708]
              tunnel: w698 -> [w704 _]
              tunnel: w695 -> [w703 _]
              frame True {
                n378 = invoke class="VI" method="FP.Open"(reference=w704, error in=w705, "Activate"=TRUE, "State"=w703) -> (error out=w706:errorcluster)  [unwired: 1 in, 4 out]
              }
              frame False {
              }
            }
          }
          frame "Close", "Closed" {
            n379 = property class="VI"(reference=w713, error in=w715) -> (reference out=w712:refnum<vi>, error out=w714:errorcluster, "FP.State"=w710:T5)
            n380 = Not Equal?(x=w710, y=T5."Closed" ("Front Panel Window:State")) -> (x != y?=w709:bool)
            n381 = case shown="True" w709 {
              tunnel: [w717 w720] -> w716
              tunnel: w714 -> [w717 w719]
              tunnel: w712 -> [_ w718]
              frame False {
              }
              frame True {
                n382 = invoke class="VI" method="FP.Close"(reference=w718, error in=w719) -> (error out=w720:errorcluster)  [unwired: 1 in, 2 out]
              }
            }
          }
          frame "Hidden", "Hide" {
            w721 = T5."Hidden" ("State")
            n383 = property class="VI"(reference=w727, error in=w726) -> (reference out=w724:refnum<vi>, error out=w725:errorcluster, "FP.State"=w723:T5)
            n384 = Not Equal?(x=w723, y=w721) -> (x != y?=w722:bool)
            n385 = case shown="True" w722 {
              tunnel: [w732 w733] -> w728
              tunnel: w725 -> [w731 w733]
              tunnel: w724 -> [w730 _]
              tunnel: w721 -> [w729 _]
              frame True {
                n386 = invoke class="VI" method="FP.Open"(reference=w730, error in=w731, "State"=w729) -> (error out=w732:errorcluster)  [unwired: 2 in, 4 out]
              }
              frame False {
              }
            }
          }
          frame "Minimize", "Minimized" {
            w734 = T5."Minimized" ("State")
            n387 = property class="VI"(reference=w740, error in=w739) -> (reference out=w737:refnum<vi>, error out=w738:errorcluster, "FP.State"=w736:T5)
            n388 = Not Equal?(x=w736, y=w734) -> (x != y?=w735:bool)
            n389 = case shown="True" w735 {
              tunnel: [w745 w746] -> w741
              tunnel: w738 -> [w744 w746]
              tunnel: w737 -> [w743 _]
              tunnel: w734 -> [w742 _]
              frame True {
                n390 = invoke class="VI" method="FP.Open"(reference=w743, error in=w744, "State"=w742) -> (error out=w745:errorcluster)  [unwired: 2 in, 4 out]
              }
              frame False {
              }
            }
          }
          frame "Maximize", "Maximized" {
            w747 = T5."Maximized" ("State")
            n391 = property class="VI"(reference=w753, error in=w752) -> (reference out=w750:refnum<vi>, error out=w751:errorcluster, "FP.State"=w749:T5)
            n392 = Not Equal?(x=w749, y=w747) -> (x != y?=w748:bool)
            n393 = case shown="True" w748 {
              tunnel: [w758 w759] -> w754
              tunnel: w751 -> [w757 w759]
              tunnel: w750 -> [w756 _]
              tunnel: w747 -> [w755 _]
              frame True {
                n394 = invoke class="VI" method="FP.Open"(reference=w756, error in=w757, "State"=w755) -> (error out=w758:errorcluster)  [unwired: 2 in, 4 out]
              }
              frame False {
              }
            }
          }
        }
        n395 = call <vilib>:"Add State(s) to Queue__JKI_lib_State_Machine.vi"("State(s) in (\"\")"=w694) -> ("States Out"=w693:string)  [unwired: 14 in]
      }
      frame "---------- Macro ----------" {
        # "Do not put any code in this frame.\n(It is a separator no-op. You can make a copy of this frame to create a new Macro frame)"
        n396 = call <vilib>:"Add State(s) to Queue__JKI_lib_State_Machine.vi"("State(s) in (\"\")"=w763) -> ("States Out"=w762:string)  [unwired: 14 in]
      }
      frame "Macro: Initialize" {
        w764 = "// UI: Cursor Set >> Busy\nData: Initialize\nInitialize Core Data\nUI: Initialize\nUI: Front Panel State >> Show\nUI: Tutorial >> Load Image\n// Image: Draw\n// UI: Cursor Set >> Idle"  # // UI: Cursor Set >> Busy Data: Initialize Initialize Core Data UI: Initialize UI: Front Panel State >> Show UI: Tutorial >> Load Image // Image: Draw // UI: Cursor Set >> Idle
        # "Initialization Macro\n(This is called once, when the VI starts)"
        n397 = call <vilib>:"Add State(s) to Queue__JKI_lib_State_Machine.vi"("State(s) in Front (\"\")"=w764, "State(s) in (\"\")"=w768) -> ("States Out"=w767:string)  [unwired: 13 in]
      }
      frame "Macro: Exit" {
        # "Exit Macro\n(This is called once, when the VI exits)"
        n398 = Unbundle By Name(w775) -> ("Core.Close Panel on Exit?"=w774:bool)
        n399 = Select(t="UI: Front Panel State >> Close", s=w774, f="") -> (s? t:f=w771:string)
        n400 = call <vilib>:"Add State(s) to Queue__JKI_lib_State_Machine.vi"("State(s) in (\"\")"=w771, "State(s) at Back (\"\")"="Data: Cleanup\nExit") -> ("States Out"=w769:string)  [unwired: 13 in]
        n401 = call <vilib>:"Add State(s) to Queue__JKI_lib_State_Machine.vi"("State(s) in Front (\"\")"=w769, "State(s) in (\"\")"=w778) -> ("States Out"=w777:string)  [unwired: 13 in]
      }
      frame "---------- Process ----------" {
        # "Template Separator\n(You can make a copy of, or modify, this frame)"
        n402 = call <vilib>:"Add State(s) to Queue__JKI_lib_State_Machine.vi"("State(s) in (\"\")"=w782) -> ("States Out"=w781:string)  [unwired: 14 in]
      }
      frame "Process: Calculate All" {
        # "Template Separator\n(You can make a copy of, or modify, this frame)"
        n403 = call <vilib>:"Add State(s) to Queue__JKI_lib_State_Machine.vi"("State(s) in Front (\"\")"="Data: Temps Clear\nData: Set Image\nUI: Cursor Set >> Busy\nUI: Progress >> Show\nProcess: Calculate All Temps\nProcess: Calculate Gradients\nProcess: Calculate Freezing Points\nProcess: Calculate Offset\nProcess: Calculate Melt Temp\nProcess: Calculate Freeze Fraction\nUI: Progress >> Hide\nUI: Cursor Set >> Idle\nUI: Tutorial >> Click on a Well to show single or click outside the plate to show all." ("State(s) in Front (\"\")"), "State(s) in (\"\")"=w787) -> ("States Out"=w786:string)  [unwired: 13 in]
      }
      frame "Process: Recalculate" {
        # "Template Separator\n(You can make a copy of, or modify, this frame)"
        n404 = call <vilib>:"Add State(s) to Queue__JKI_lib_State_Machine.vi"("State(s) in Front (\"\")"="Process: Calculate Gradients\nProcess: Calculate Freezing Points\nProcess: Calculate Melt Temp\nProcess: Calculate Freeze Fraction" ("State(s) in Front (\"\")"), "State(s) in (\"\")"=w792) -> ("States Out"=w791:string)  [unwired: 13 in]
      }
      frame "Process: Calculate Temps" {
        # "Your code here.\n(You can make a copy of, or modify, this frame)"
        n405 = Unbundle By Name(w798) -> ("Image Out"=w796:T1, "Points.Pixels"=w795:cluster{"X":i32, "Y":i32}[][], "Points.Top Left.X"=w806:sgl, "Points.Top Right.X"=w805:sgl, "Points.Bottom Left.X"=w804:sgl, "Points.Bottom Right.X"=w803:sgl)
        n406 = Equal To 0?(x=w806) -> (x = 0?=w802:bool)
        n407 = Equal To 0?(x=w805) -> (x = 0?=w801:bool)
        n408 = Equal To 0?(x=w804) -> (x = 0?=w800:bool)
        n409 = Equal To 0?(x=w803) -> (x = 0?=w799:bool)
        n410 = local read "Points"() -> (w794:T2[])
        n411 = Compound Arithmetic op=OR(w802, w801, w800, w799) -> (w797:bool)
        n412 = case shown="False" w797 {
          tunnel: w796 -> [w812 w813]
          tunnel: w795 -> [w811 _]
          tunnel: w794 -> [_ _]
          tunnel: [w810 w813] -> w793
          frame False {
            n413 = call "TCam_WellTemp.vi"("Pixels"=w811, "Image in"=w812) -> ("Image Out"=w810:T1)  [unwired: 7 in, 2 out]
          }
          frame True {
          }
        }
        n414 = local write "Image"(w793) -> ()
        n415 = call <vilib>:"Add State(s) to Queue__JKI_lib_State_Machine.vi"("State(s) in (\"\")"=w809) -> ("States Out"=w808:string)  [unwired: 14 in]
      }
      frame "Process: Calculate Well" {
        # "Your code here.\n(You can make a copy of, or modify, this frame)"
        n416 = Unbundle By Name(w815) -> ("Image Out"=w820:T1, "Points.Pixels"=w819:cluster{"X":i32, "Y":i32}[][], "Points.Top Left.X"=w828:sgl, "Points.Top Right.X"=w827:sgl, "Points.Bottom Left.X"=w826:sgl, "Points.Bottom Right.X"=w825:sgl)
        n417 = local read "Points"() -> (w818:T2[])
        n418 = Equal To 0?(x=w828) -> (x = 0?=w824:bool)
        n419 = Equal To 0?(x=w827) -> (x = 0?=w823:bool)
        n420 = Equal To 0?(x=w826) -> (x = 0?=w822:bool)
        n421 = Equal To 0?(x=w825) -> (x = 0?=w821:bool)
        n422 = Compound Arithmetic op=OR(w824, w823, w822, w821) -> (w817:bool)
        n423 = case shown="False" w817 {
          tunnel: w820 -> [w853 _]
          tunnel: w819 -> [w852 _]
          tunnel: w818 -> [w851 _]
          tunnel: [w846 _] -> w816
          tunnel: w815 -> [w839 _]
          tunnel: w815 -> [w837 w858]
          tunnel: [w836 w858] -> w814
          frame False {
            n424 = local read "ImageIdx"() -> (w833:u32)
            n425 = property on="ImageIdx" class="Slide (strict)"() -> ("Scale.Maximum"=w841:dbl)  [unwired: 2 in, 2 out]
            n426 = call "TCam_WellCalculater.vi"("DrawTempOverlay"=TRUE, "Well Pos"=w851, "Pixels"=w852, "Image in"=w853, "index"="Well") -> ("Image Out"=w850:T1, "mean"=w835:dbl)  [unwired: 5 in]
            n427 = Increment(x=w833) -> (x+1=w847:u32)
            n428 = local write "Image"(w850) -> ()
            n429 = Greater?(x=w847, y=w841) -> (0:w849:bool)
            n430 = case shown="False" w849 {
              tunnel: w847 -> [_ w857]
              tunnel: [w856 w857] -> w848
              tunnel: w847 -> [w856 _]
              tunnel: ["Data: Set Image\nProcess: Calculate Well" ("State(s) in Front (\"\")") _] -> w846
              tunnel: [TRUE _] -> w845
              frame False {
              }
              frame True {
              }
            }
            n431 = Unbundle By Name(w839) -> ("Temps"=w838:dbl[])
            n432 = Divide(x=w833, y=w841) -> (x/y=w844:dbl)
            n433 = property on="Temps single" class="WFGraph (strict)"("Cursor.Cursor X"=w833) -> ()  [unwired: 2 in, 2 out]
            n434 = Multiply(x=w844, y=100.0) -> (x*y=w842:dbl)
            n435 = Build Array (concatenate)(w838, w835) -> (w834:dbl[])
            "Temps single" <- w834
            n436 = local write "Slide"(w842) -> ()
            n437 = Bundle By Name(cluster=w837, "Temps"=w834) -> (w836:T4)
            n438 = local write "ImageIdx"(w848) -> ()
            n439 = property on="Slide" class="Slide (strict)"("Visible"=w845) -> ()  [unwired: 2 in, 2 out]
          }
          frame True {
          }
        }
        n440 = call <vilib>:"Add State(s) to Queue__JKI_lib_State_Machine.vi"("State(s) in Front (\"\")"=w816, "State(s) in (\"\")"=w831) -> ("States Out"=w830:string)  [unwired: 13 in]
      }
      frame "Process: Calculate All Temps" {
        # "Your code here.\n(You can make a copy of, or modify, this frame)"
        n441 = Unbundle By Name(w861) -> ("img_array"=w864:T1[], "Points.Pixels"=w863:cluster{"X":i32, "Y":i32}[][], "Points.Top Left.X"=w872:sgl, "Points.Top Right.X"=w871:sgl, "Points.Bottom Left.X"=w870:sgl, "Points.Bottom Right.X"=w869:sgl)
        n442 = Equal To 0?(x=w872) -> (x = 0?=w868:bool)
        n443 = Equal To 0?(x=w871) -> (x = 0?=w867:bool)
        n444 = Equal To 0?(x=w870) -> (x = 0?=w866:bool)
        n445 = Equal To 0?(x=w869) -> (x = 0?=w865:bool)
        n446 = Compound Arithmetic op=OR(w868, w867, w866, w865) -> (w862:bool)
        n447 = case shown="False" w862 {
          tunnel: w864 -> [w878 _]
          tunnel: w863 -> [w880 _]
          tunnel: [TRUE ("Visible") FALSE ("Visible")] -> w859
          tunnel: [w876 dbl[][] []] -> w860
          frame False {
            n448 = for {
              N -> [w883]
              tunnel: w878 -> [w894] mode=indexing
              tunnel: w880 -> [w893]
              tunnel: [w892] -> w879 mode=indexing
              workers-P: _ -> [_]
              i -> [w881]
              n449 = call "TCam_WellTemp.vi"("Pixels"=w893, "Image in"=w894) -> ("Temps"=w892:dbl[])  [unwired: 7 in, 2 out]
              n450 = property on="ImageIdx" class="Slide (strict)"() -> ("Scale.Maximum"=w889:dbl)  [unwired: 2 in, 2 out]
              n451 = local read "img"() -> (w891:i32)
              n452 = property on="Temps" class="WFGraph (strict)"("Cursor.Cursor X"=w881) -> ()  [unwired: 2 in, 2 out]
              n453 = Increment(x=w891) -> (x+1=w882:i32)
              n454 = Divide(x=w882, y=w889) -> (x/y=w896:dbl)
              n455 = local write "img"(w882) -> ()
              n456 = Format Into String(w882) -> (resulting string=w888:string)  [unwired: 3 in, 1 out]
              n457 = Multiply(x=w896, y=100.0) -> (x*y=w890:dbl)
              n458 = property on="Temps grads" class="WFGraph (strict)"("Cursor.Cursor X"=w881) -> ()  [unwired: 2 in, 2 out]
              n459 = Format Into String(w883) -> (resulting string=w884:string)  [unwired: 3 in, 1 out]
              n460 = local write "Slide"(w890) -> ()
              n461 = Concatenate Strings("Processing image " ("Tutorial"), w888, " of " ("Tutorial"), w884) -> (w887:string)
              n462 = property on="FrozenFractionGraph" class="WFGraph (strict)"("Cursor.Cursor X"=w881) -> ()  [unwired: 2 in, 2 out]
              n463 = local write "Tutorial"(w887) -> ()
            }
            n464 = Transpose 2D Array(2D array=w879) -> (transposed array=w876:dbl[][])
          }
          frame True {
          }
        }
        "Temps" <- w860
        n465 = property on="Correct Data" class="Bool"("Visible"=w859) -> ()  [unwired: 2 in, 2 out]
        n466 = call <vilib>:"Add State(s) to Queue__JKI_lib_State_Machine.vi"("State(s) in (\"\")"=w875) -> ("States Out"=w874:string)  [unwired: 14 in]
      }
      frame "Process: Calculate Gradients" {
        # "Your code here.\n(You can make a copy of, or modify, this frame)"
        n467 = local read "Temps"() -> (w900:dbl[][])
        n468 = for {
          tunnel: w900 -> [w909] mode=indexing
          workers-P: _ -> [_]
          tunnel: [w905] -> w899 mode=indexing
          n469 = Array Size(array=w909) -> (size(s)=w908:i32)
          n470 = Decrement(x=w908) -> (x-1=w907:i32)
          n471 = for {
            N: w907 -> [_]
            tunnel: w909 -> [w917]
            shift-right: [w911] -> w905
            shift-left: dbl[] [0.0] -> [w910]
            i -> [w916]
            n472 = Increment(x=w916) -> (x+1=w915:i32)
            n473 = Index Array(array=w917, index=w916) -> (element=w913:dbl)
            n474 = Index Array(array=w917, index=w915) -> (element=w914:dbl)
            n475 = Subtract(x=w914, y=w913) -> (x-y=w912:dbl)
            n476 = Build Array (concatenate)(w910, w912) -> (w911:dbl[])
          }
        }
        "Temps grads" <- w899
        n477 = call <vilib>:"Add State(s) to Queue__JKI_lib_State_Machine.vi"("State(s) in (\"\")"=w904) -> ("States Out"=w903:string)  [unwired: 14 in]
      }
      frame "Process: Calculate Freezing Points" {
        # "Your code here.\n(You can make a copy of, or modify, this frame)"
        n478 = local read "Temps grads"() -> (w922:dbl[][])
        n479 = local read "Temps"() -> (w920:dbl[][])
        n480 = Unbundle By Name(w927) -> ("Config.Freezing.EndIndex"=w918:i32, "Config.Freezing.Cutoff"=w926:dbl)
        n481 = local write "FreezeTemps"(dbl[] []) -> ()
        n482 = local write "FreezeIdx"(i32[] []) -> ()
        n483 = local write "FreezeArray"(bool[] []) -> ()
        n484 = Array Subset(array=w920, length (col)=w918) -> (w919:dbl[][])  [unwired: 3 in]
        n485 = Array Subset(array=w922, length (col)=w918) -> (w921:dbl[][])  [unwired: 3 in]
        n486 = for {
          tunnel: w921 -> [w939] mode=indexing
          workers-P: _ -> [_]
          tunnel: w919 -> [w948] mode=indexing
          tunnel: [w943] -> w931 mode=indexing
          tunnel: [w941] -> w930 mode=indexing
          tunnel: [w937] -> w929 mode=indexing
          tunnel: w926 -> [w936]
          # "Gradient Check"
          n487 = call <vilib>:"Std Deviation and Variance.vi"("X"=w939) -> ("standard deviation"=w938:dbl)  [unwired: 1 in, 2 out]
          n488 = Array Max & Min(array=w939) -> (max value=w946:dbl, max index (indices)=w942:i32)  [unwired: 2 out]
          n489 = Multiply(x=w936, y=w938) -> (x*y=w945:dbl)
          n490 = Array Subset(array=w948, length=w942) -> (w947:dbl[])  [unwired: 1 in]
          n491 = Greater?(x=w946, y=w945) -> (0:w944:bool)
          n492 = Array Max & Min(array=w947) -> (min value=w940:dbl, min index (indices)=w935:i32)  [unwired: 2 out]
          n493 = case shown="True" w944 {
            selector: w944 -> [w950 w951]
            tunnel: [w949 w953] -> w943
            tunnel: w935 -> [_ w953]
            tunnel: [w949 w952] -> w941
            tunnel: w940 -> [_ w952]
            tunnel: [w950 w951] -> w937
            frame False {
              w949 = 0.0
            }
            frame True {
            }
          }
        }
        "FreezeIdx" <- w931
        "FreezeTemps" <- w930
        "FreezeArray" <- w929
        n494 = call <vilib>:"Add State(s) to Queue__JKI_lib_State_Machine.vi"("State(s) in Front (\"\")"="UI: Menu Save >> True\nUI: Menu Overlay Temps >> True" ("State(s) in Front (\"\")"), "State(s) in (\"\")"=w934) -> ("States Out"=w933:string)  [unwired: 13 in]
      }
      frame "Process: Calculate Melt Temp" {
        # "Your code here.\n(You can make a copy of, or modify, this frame)"
        n495 = local read "FreezeIdx"() -> (w956:i32[])
        n496 = local read "Temps"() -> (w955:dbl[][])
        n497 = for {
          tunnel: w956 -> [w961] mode=indexing
          workers-P: _ -> [_]
          tunnel: w955 -> [w966] mode=indexing
          tunnel: [w964] -> w954 mode=indexing
          n498 = Array Subset(array=w966, index=w961) -> (w965:dbl[])  [unwired: 1 in]
          n499 = Not Equal To 0?(x=w961) -> (x != 0?=w962:bool)
          n500 = Array Max & Min(array=w965) -> (max value=w963:dbl)  [unwired: 3 out]
          n501 = case shown="False" w962 {
            tunnel: [0.0 w968] -> w964
            tunnel: w963 -> [_ w968]
            frame False {
            }
            frame True {
            }
          }
        }
        "MeltTemps" <- w954
        n502 = call <vilib>:"Add State(s) to Queue__JKI_lib_State_Machine.vi"("State(s) in (\"\")"=w960) -> ("States Out"=w959:string)  [unwired: 14 in]
      }
      frame "Process: Calculate Freeze Fraction" {
        # "Your code here.\n(You can make a copy of, or modify, this frame)"
        n503 = property on="FrozenFractionGraph" class="WFGraph (strict)"("Active Plot"=u32 0, "Legend Visible"=TRUE ("Legend:Visible")) -> ()  [unwired: 2 in, 2 out]
        n504 = local read "PartitionArray"() -> (w972:string[])
        n505 = local read "FreezeTemps"() -> (w977:dbl[])
        n506 = local read "FreezeIdx"() -> (w975:i32[])
        n507 = local read "Temps"() -> (w976:dbl[][])
        n508 = call "FrozenFraction_Calcualte.vi"("FreezeIdx"=w975, "Temps"=w976, "FreezeTemps"=w977, "PartitionArray"=w972) -> ("FreezeFract Concatinated"=→"FreezeFract Concatinated":dbl[], "FrozenFractionGraph"=→"FrozenFractionGraph":dbl[][])  [unwired: 6 in]
        n509 = call "WellPartition_Index.vi"("PartitionArray"=w972) -> ("Unique Part Array"=w971:string[])  [unwired: 1 in, 1 out]
        n510 = for {
          tunnel: w971 -> [w983] mode=indexing
          i -> [w982]
          n511 = property on="FrozenFractionGraph" class="WFGraph (strict)"("Active Plot"=w982, "Plot.Plot Name"=w983) -> ()  [unwired: 2 in, 2 out]
        }
        n512 = call <vilib>:"Add State(s) to Queue__JKI_lib_State_Machine.vi"("State(s) in (\"\")"=w981) -> ("States Out"=w980:string)  [unwired: 14 in]
      }
      frame "Process: Calculate Offset" {
        # "Your code here.\n(You can make a copy of, or modify, this frame)"
        n513 = local read "ThermTemps"() -> (w985:dbl[])
        n514 = call "TCam_FixpointTemps.vi"("input cluster"=w986, "Therm_Temps"=w985) -> ("Offsets"=→"Offsets":dbl[])  [unwired: 1 out]
        n515 = call <vilib>:"Add State(s) to Queue__JKI_lib_State_Machine.vi"("State(s) in (\"\")"=w989) -> ("States Out"=w988:string)  [unwired: 14 in]
      }
      frame "Process: Correct Offset" {
        # "Your code here.\n(You can make a copy of, or modify, this frame)"
        n516 = local read "Temps"() -> (w992:dbl[][])
        n517 = local read "Offsets"() -> (w991:dbl[])
        n518 = for {
          tunnel: w992 -> [w999] mode=indexing
          tunnel: w991 -> [w998]
          tunnel: [w997] -> w990 mode=indexing
          n519 = Subtract(x=w999, y=w998) -> (x-y=w997:dbl[])
        }
        n520 = local write "Temps"(w990) -> ()
        n521 = call <vilib>:"Add State(s) to Queue__JKI_lib_State_Machine.vi"("State(s) in (\"\")"=w996) -> ("States Out"=w995:string)  [unwired: 14 in]
      }
      frame "Process: Remove Offset" {
        # "Your code here.\n(You can make a copy of, or modify, this frame)"
        n522 = local read "Temps"() -> (w1002:dbl[][])
        n523 = local read "Offsets"() -> (w1001:dbl[])
        n524 = for {
          tunnel: w1002 -> [w1009] mode=indexing
          tunnel: w1001 -> [w1008]
          tunnel: [w1007] -> w1000 mode=indexing
          n525 = Add(x=w1009, y=w1008) -> (x+y=w1007:dbl[])
        }
        n526 = local write "Temps"(w1000) -> ()
        n527 = call <vilib>:"Add State(s) to Queue__JKI_lib_State_Machine.vi"("State(s) in (\"\")"=w1006) -> ("States Out"=w1005:string)  [unwired: 14 in]
      }
      frame "---------- Image ----------" {
        # "Template Separator\n(You can make a copy of, or modify, this frame)"
        n528 = call <vilib>:"Add State(s) to Queue__JKI_lib_State_Machine.vi"("State(s) in (\"\")"=w1013) -> ("States Out"=w1012:string)  [unwired: 14 in]
      }
      frame "Image: Draw" {
        # "Template Separator\n(You can make a copy of, or modify, this frame)"
        n529 = call <vilib>:"Add State(s) to Queue__JKI_lib_State_Machine.vi"("State(s) in Front (\"\")"="UI: Cursor Set >> Busy\nImage: Clear ROI\nImage: Calculate BR\nImage: Calculate y space\nImage: Calculate x space\nImage: Calculate Positions\nImage: Drawlines\nImage: Draw Points\nUI: Cursor Set >> Idle" ("State(s) in Front (\"\")"), "State(s) in (\"\")"=w1018) -> ("States Out"=w1017:string)  [unwired: 13 in]
      }
      frame "Image: Redraw" {
        # "Template Separator\n(You can make a copy of, or modify, this frame)"
        n530 = call <vilib>:"Add State(s) to Queue__JKI_lib_State_Machine.vi"("State(s) in Front (\"\")"="UI: Cursor Set >> Busy\nImage: Clear ROI\nImage: Drawlines\nImage: Draw Points\nProcess: Calculate Temps\nUI: Cursor Set >> Idle" ("State(s) in Front (\"\")"), "State(s) in (\"\")"=w1023) -> ("States Out"=w1022:string)  [unwired: 13 in]
      }
      frame "Image: Set Cursors" {
        w1027 = -45.0 ("X Scale.Range:Minimum")
        w1028 = 40.0 ("Y Scale.Range:Maximum")
        w1024 = 0 ("lower limit")
        # "Template Separator\n(You can make a copy of, or modify, this frame)"
        n531 = local read "ImageIdx"() -> (w1026:u32)
        n532 = local read "maxSize"() -> (w1025:i32)
        n533 = property on="Temps grads" class="WFGraph (strict)"("Cursor.Cursor X"=w1026, "XScale.Maximum"=w1025, "XScale.Minimum"=w1024) -> ()  [unwired: 2 in, 2 out]
        n534 = property on="Temps single" class="WFGraph (strict)"("Cursor.Cursor X"=w1026, "XScale.Maximum"=w1025, "XScale.Minimum"=w1024, "YScale.Maximum"=w1028, "YScale.Minimum"=w1027) -> ()  [unwired: 2 in, 2 out]
        n535 = property on="Temps" class="WFGraph (strict)"("Cursor.Cursor X"=w1026, "XScale.Maximum"=w1025, "XScale.Minimum"=w1024, "YScale.Maximum"=w1028, "YScale.Minimum"=w1027) -> ()  [unwired: 2 in, 2 out]
        n536 = property on="FrozenFractionGraph" class="WFGraph (strict)"("Cursor.Cursor X"=w1026, "XScale.Maximum"=w1025, "XScale.Minimum"=w1024) -> ()  [unwired: 2 in, 2 out]
        n537 = property on="Fraction Single" class="WFGraph (strict)"("Cursor.Cursor X"=w1026, "XScale.Maximum"=w1025, "XScale.Minimum"=w1024) -> ()  [unwired: 2 in, 2 out]
        n538 = property on="Temps single grad" class="WFGraph (strict)"("Cursor.Cursor X"=w1026, "XScale.Maximum"=w1025, "XScale.Minimum"=w1024) -> ()  [unwired: 2 in, 2 out]
        n539 = property on="Temps" class="WFGraph (strict)"("Cursor.Cursor X"=w1026, "XScale.Maximum"=w1025, "XScale.Minimum"=w1024) -> ()  [unwired: 2 in, 2 out]
        n540 = call <vilib>:"Add State(s) to Queue__JKI_lib_State_Machine.vi"("State(s) in (\"\")"=w1032) -> ("States Out"=w1031:string)  [unwired: 14 in]
      }
      frame "Image: Drawlines" {
        # "Template Separator\n(You can make a copy of, or modify, this frame)"
        n541 = Unbundle By Name(w1033) -> ("Points.Top Left.X"=w1049:sgl, "Points.Top Right.X"=w1048:sgl, "Points.Bottom Left.X"=w1047:sgl, "Points.Bottom Right.X"=w1046:sgl)
        n542 = Equal To 0?(x=w1049) -> (x = 0?=w1045:bool)
        n543 = Equal To 0?(x=w1048) -> (x = 0?=w1044:bool)
        n544 = Equal To 0?(x=w1047) -> (x = 0?=w1035:bool)
        n545 = Equal To 0?(x=w1046) -> (x = 0?=w1036:bool)
        n546 = Or(x=w1035, y=w1036) -> (x .or. y?=w1034:bool)
        n547 = Select(t="", s=w1035, f="Image: Draw Line >> TL_BL\n") -> (s? t:f=w1041:string)
        n548 = Select(t="", s=w1034, f="Image: Draw Line >> TR_BR\nImage: Draw Line >> BL_BR\nImage: Draw Line >> Vertical\nImage: Draw Line >> Horizontal") -> (s? t:f=w1038:string)
        n549 = case shown="False" w1045 {
          tunnel: w1044 -> [w1056 _]
          tunnel: w1041 -> [w1055 _]
          tunnel: w1038 -> [w1054 _]
          tunnel: [w1053 _] -> w1037
          frame False {
            n550 = case shown="False" w1056 {
              tunnel: w1055 -> [w1059 _]
              tunnel: w1054 -> [w1058 _]
              tunnel: [w1057 _] -> w1053
              frame False {
                n551 = Concatenate Strings("Image: Draw Line >> TL_TR\n", w1059, w1058) -> (w1057:string)
              }
              frame True {
              }
            }
          }
          frame True {
          }
        }
        n552 = call <vilib>:"Add State(s) to Queue__JKI_lib_State_Machine.vi"("State(s) in Front (\"\")"=w1037, "State(s) in (\"\")"=w1052) -> ("States Out"=w1051:string)  [unwired: 13 in]
      }
      frame "Image: Draw Line" {
        w1061 = u32 2  # Width
        # "Your code here.\n(You can make a copy of, or modify, this frame)"
        n553 = Unbundle By Name(w1065) -> ("Image Out"=w1066:T1)
        n554 = case shown="\"Vertical\"" w1067 {
          tunnel: w1066 -> [w1071 w1079 w1088 w1095 w1101 w1106 w1115]
          tunnel: w1065 -> [_ w1080 w1089 w1090 w1096 w1110 w1119]
          tunnel: [w1071 w1074 w1087 w1094 w1100 w1102 w1111] -> w1064
          tunnel: w1063 -> [w1070 w1078 w1086 w1093 w1099 w1104 w1114]
          tunnel: [w1070 w1073 w1085 w1092 w1098 w1103 w1113] -> w1062
          tunnel: w1061 -> [_ w1072 w1081 _ _ w1105 w1112]
          frame "False", Default {
          }
          frame "TL_TR" {
            n555 = Unbundle By Name(w1080) -> ("Points.Top Left"=w1077:T2, "Points.Top Right"=w1076:T2)
            n556 = Build Array(w1077, w1076) -> (w1075:T2[])
            n557 = call "IMAQ Overlay Multiple Lines 2"("Image"=w1079, "Line End Points"=w1075, "error in (no error)"=w1078, "Width"=w1072) -> ("Image Out"=w1074:T1, "error out"=w1073:errorcluster)  [unwired: 10 in]
          }
          frame "TL_BL" {
            n558 = Unbundle By Name(w1089) -> ("Points.Top Left"=w1084:T2, "Points.Bottom Left"=w1083:T2)
            n559 = Build Array(w1084, w1083) -> (w1082:T2[])
            n560 = call "IMAQ Overlay Multiple Lines 2"("Image"=w1088, "Line End Points"=w1082, "error in (no error)"=w1086, "Width"=w1081) -> ("Image Out"=w1087:T1, "error out"=w1085:errorcluster)  [unwired: 10 in]
          }
          frame "Vertical" {
            n561 = call "TCam_VerticalLines.vi"("Width"=u32 1, "error in (no error)"=w1093, "Cluster"=w1090, "Refnum in"=w1095) -> ("error out"=w1092:errorcluster, "Refnum out"=w1094:T1)  [unwired: 6 in]
          }
          frame "Horizontal" {
            n562 = call "TCam_HorizontalLines.vi"("Width"=u32 1, "error in (no error)"=w1099, "Cluster"=w1096, "Refnum in"=w1101) -> ("error out"=w1098:errorcluster, "Refnum out"=w1100:T1)  [unwired: 6 in]
          }
          frame "TR_BR" {
            n563 = Unbundle By Name(w1110) -> ("Points.Top Right"=w1109:T2, "Points.Bottom Right"=w1108:T2)
            n564 = Build Array(w1109, w1108) -> (w1107:T2[])
            n565 = call "IMAQ Overlay Multiple Lines 2"("Image"=w1106, "Line End Points"=w1107, "error in (no error)"=w1104, "Width"=w1105) -> ("Image Out"=w1102:T1, "error out"=w1103:errorcluster)  [unwired: 10 in]
          }
          frame "BL_BR" {
            n566 = Unbundle By Name(w1119) -> ("Points.Bottom Left"=w1118:T2, "Points.Bottom Right"=w1117:T2)
            n567 = Build Array(w1118, w1117) -> (w1116:T2[])
            n568 = call "IMAQ Overlay Multiple Lines 2"("Image"=w1115, "Line End Points"=w1116, "error in (no error)"=w1114, "Width"=w1112) -> ("Image Out"=w1111:T1, "error out"=w1113:errorcluster)  [unwired: 10 in]
          }
        }
        n569 = local write "Image"(w1064) -> ()
        n570 = call <vilib>:"Add State(s) to Queue__JKI_lib_State_Machine.vi"("State(s) in (\"\")"=w1069) -> ("States Out"=w1068:string)  [unwired: 14 in]
      }
      frame "Image: Draw Points" {
        # "Your code here.\n(You can make a copy of, or modify, this frame)"
        n571 = Unbundle By Name(w1122) -> ("Points.Top Left.X"=w1131:sgl, "Points.Top Right.X"=w1130:sgl, "Points.Bottom Left.X"=w1129:sgl, "Points.Bottom Right.X"=w1128:sgl)
        n572 = Equal To 0?(x=w1131) -> (x = 0?=w1127:bool)
        n573 = Equal To 0?(x=w1130) -> (x = 0?=w1126:bool)
        n574 = Equal To 0?(x=w1129) -> (x = 0?=w1125:bool)
        n575 = Equal To 0?(x=w1128) -> (x = 0?=w1124:bool)
        n576 = Unbundle By Name(w1122) -> ("Image Out"=w1133:T1, "Scan Area"=w1120:dbl)
        n577 = Compound Arithmetic op=OR(w1127, w1126, w1125, w1124) -> (w1123:bool)
        n578 = case shown="False" w1123 {
          tunnel: w1133 -> [w1142 _]
          tunnel: w1122 -> [w1139 w1143]
          tunnel: [w1137 w1143] -> w1121
          tunnel: w1120 -> [w1136 _]
          frame False {
            n579 = local read "Points"() -> (w1141:T2[])
            n580 = call "TCam_CenterArray.vi"("Size"=w1136, "Point Array"=w1141, "Image in"=w1142) -> ("Array"=w1138:cluster{"X":i32, "Y":i32}[][], "Image"=w1140:T1)  [unwired: 3 in]
            n581 = local write "Image"(w1140) -> ()
            n582 = Bundle By Name(cluster=w1139, "Points.Pixels"=w1138) -> (w1137:T4)
          }
          frame True {
          }
        }
        n583 = call <vilib>:"Add State(s) to Queue__JKI_lib_State_Machine.vi"("State(s) in (\"\")"=w1135) -> ("States Out"=w1134:string)  [unwired: 14 in]
      }
      frame "Image: Calculate x space" {
        # "Your code here.\n(You can make a copy of, or modify, this frame)"
        n584 = Unbundle By Name(w1152) -> ("Points.Top Left"=w1158:T2, "Points.Top Right"=w1157:T2, "PCR Size"=w1144:u16)
        n585 = case shown="0, Default" w1144 {
          tunnel: [24 12] -> w1145
          frame 0, Default {
          }
          frame 1 {
          }
        }
        n586 = Unbundle(w1158) -> ("X"=w1155:sgl, "Y"=w1153:sgl)
        n587 = Unbundle(w1157) -> ("X"=w1156:sgl, "Y"=w1154:sgl)
        n588 = Subtract(x=w1156, y=w1155) -> (x-y=w1149:sgl)
        n589 = Subtract(x=w1154, y=w1153) -> (x-y=w1147:sgl)
        n590 = Decrement(x=w1145) -> (x-1=w1148:i32)
        n591 = Divide(x=w1149, y=w1148) -> (x/y=w1150:sgl)
        n592 = Divide(x=w1147, y=w1148) -> (x/y=w1146:sgl)
        n593 = Bundle By Name(cluster=w1152, "Points.x_space"=w1150, "Points.y_space"=w1146) -> (w1151:T4)
        n594 = call <vilib>:"Add State(s) to Queue__JKI_lib_State_Machine.vi"("State(s) in (\"\")"=w1161) -> ("States Out"=w1160:string)  [unwired: 14 in]
      }
      frame "Image: Calculate BR" {
        # "Your code here.\n(You can make a copy of, or modify, this frame)"
        n595 = Unbundle By Name(w1172) -> ("Points.Top Left"=w1178:T2, "Points.Top Right"=w1177:T2, "Points.Bottom Left"=w1170:T2)
        n596 = Unbundle(w1178) -> ("X"=w1175:sgl, "Y"=w1173:sgl)
        n597 = Unbundle(w1170) -> ("X"=w1169:sgl, "Y"=w1167:sgl)
        n598 = Unbundle(w1177) -> ("X"=w1176:sgl, "Y"=w1174:sgl)
        n599 = Subtract(x=w1176, y=w1175) -> (x-y=w1168:sgl)
        n600 = Add(x=w1169, y=w1168) -> (x+y=w1164:sgl)
        n601 = Subtract(x=w1174, y=w1173) -> (x-y=w1166:sgl)
        n602 = Add(x=w1166, y=w1167) -> (x+y=w1165:sgl)
        n603 = Bundle By Name(cluster=w1172, "Points.Bottom Right.X"=w1164, "Points.Bottom Right.Y"=w1165) -> (w1171:T4)
        n604 = call <vilib>:"Add State(s) to Queue__JKI_lib_State_Machine.vi"("State(s) in (\"\")"=w1181) -> ("States Out"=w1180:string)  [unwired: 14 in]
      }
      frame "Image: Calculate y space" {
        # "Your code here.\n(You can make a copy of, or modify, this frame)"
        n605 = Unbundle By Name(w1190) -> ("Points.Top Left"=w1196:T2, "Points.Bottom Left"=w1195:T2, "PCR Size"=w1182:u16)
        n606 = case shown="1" w1182 {
          tunnel: [16 8] -> w1183
          frame 0, Default {
          }
          frame 1 {
          }
        }
        n607 = Unbundle(w1196) -> ("X"=w1193:sgl, "Y"=w1191:sgl)
        n608 = Unbundle(w1195) -> ("X"=w1194:sgl, "Y"=w1192:sgl)
        n609 = Subtract(x=w1194, y=w1193) -> (x-y=w1187:sgl)
        n610 = Subtract(x=w1192, y=w1191) -> (x-y=w1185:sgl)
        n611 = Decrement(x=w1183) -> (x-1=w1186:i32)
        n612 = Divide(x=w1187, y=w1186) -> (x/y=w1188:sgl)
        n613 = Divide(x=w1185, y=w1186) -> (x/y=w1184:sgl)
        n614 = Bundle By Name(cluster=w1190, "Points.x space 2"=w1188, "Points.y space 2"=w1184) -> (w1189:T4)
        n615 = call <vilib>:"Add State(s) to Queue__JKI_lib_State_Machine.vi"("State(s) in (\"\")"=w1199) -> ("States Out"=w1198:string)  [unwired: 14 in]
      }
      frame "Image: Calculate Positions" {
        # "Your code here.\n(You can make a copy of, or modify, this frame)"
        n616 = Unbundle By Name(w1204) -> ("Scan Area"=w1202:dbl, "Points.Top Left.X"=w1212:sgl, "Points.Top Right.X"=w1211:sgl, "Points.Bottom Left.X"=w1210:sgl, "Points.Bottom Right.X"=w1209:sgl)
        n617 = Equal To 0?(x=w1212) -> (x = 0?=w1208:bool)
        n618 = Equal To 0?(x=w1211) -> (x = 0?=w1207:bool)
        n619 = Equal To 0?(x=w1210) -> (x = 0?=w1206:bool)
        n620 = Equal To 0?(x=w1209) -> (x = 0?=w1205:bool)
        n621 = Compound Arithmetic op=OR(w1208, w1207, w1206, w1205) -> (w1203:bool)
        n622 = case shown="False" w1203 {
          tunnel: w1204 -> [w1217 _]
          tunnel: w1202 -> [w1216 _]
          frame False {
            n623 = call "TCam_PointCalculator.vi"("Cluster"=w1217, "Size"=w1216) -> ("Points"=→"Points":T2[])  [unwired: 9 in]
          }
          frame True {
          }
        }
        n624 = call <vilib>:"Add State(s) to Queue__JKI_lib_State_Machine.vi"("State(s) in (\"\")"=w1215) -> ("States Out"=w1214:string)  [unwired: 14 in]
      }
      frame "Image: Clear ROI" {
        # "Your code here.\n(You can make a copy of, or modify, this frame)"
        n625 = Unbundle By Name(w1222) -> ("Image Out"=w1221:T1)
        n626 = call "IMAQ Clear Overlay"("error in (no error)"=w1220, "Image"=w1221) -> ("error out"=w1219:errorcluster)  [unwired: 8 in, 1 out]
        n627 = call <vilib>:"Add State(s) to Queue__JKI_lib_State_Machine.vi"("State(s) in (\"\")"=w1224) -> ("States Out"=w1223:string)  [unwired: 14 in]
      }
      frame "Image: Set ROI" {
        # "Your code here.\n(You can make a copy of, or modify, this frame)"
        n628 = Unbundle By Name(w1228) -> ("State"=w1230:i32)
        n629 = case shown="0, Default" w1230 {
          tunnel: [w1234 w1237 w1239 w1241] -> w1229
          tunnel: w1228 -> [w1235 w1236 w1238 w1240]
          frame 0, Default {
            n630 = Unbundle By Name(w1235) -> ("Points.Top Left"=w1234:T2)
          }
          frame 1 {
            n631 = Unbundle By Name(w1236) -> ("Points.Top Right"=w1237:T2)
          }
          frame 2 {
            n632 = Unbundle By Name(w1238) -> ("Points.Bottom Left"=w1239:T2)
          }
          frame 3 {
            n633 = Unbundle By Name(w1240) -> ("Points.Bottom Right"=w1241:T2)
          }
        }
        n634 = call "IMAQ Convert Point to ROI"("error in (no error)"=w1227, "Point"=w1229) -> ("error out"=w1226:errorcluster, "ROI Descriptor"=w1231:T10)  [unwired: 7 in]
        n635 = property on="Image" class="ImageControl"(error in=w1226, "ROI"=w1231) -> (error out=w1225:errorcluster)  [unwired: 1 in, 1 out]
        n636 = call <vilib>:"Add State(s) to Queue__JKI_lib_State_Machine.vi"("State(s) in (\"\")"=w1233) -> ("States Out"=w1232:string)  [unwired: 14 in]
      }
      frame "---------- Overlay ----------" {
        # "Template Separator\n(You can make a copy of, or modify, this frame)"
        n637 = call <vilib>:"Add State(s) to Queue__JKI_lib_State_Machine.vi"("State(s) in (\"\")"=w1245) -> ("States Out"=w1244:string)  [unwired: 14 in]
      }
      frame "Overlay: Overlay Freeze" {
        # "Your code here.\n(You can make a copy of, or modify, this frame)"
        n638 = local read "FreezeArray"() -> (w1247:bool[])
        n639 = local read "FreezeIdx"() -> (w1248:i32[])
        n640 = local read "Points"() -> (w1249:T2[])
        n641 = Unbundle By Name(w1251) -> ("img_array"=w1250:T1[])
        n642 = call "OverlayFreezeRange.vi"("FreezeIdx"=w1248, "FreezeArray"=w1247) -> ("Range"=w1246:i32)
        n643 = for {
          N -> [w1257]
          tunnel: w1248 -> [w1269] mode=indexing
          tunnel: w1250 -> [w1270]
          tunnel: w1249 -> [w1268] mode=indexing
          tunnel: w1247 -> [w1267] mode=indexing
          tunnel: w1246 -> [w1266]
          n644 = local read "img"() -> (w1258:i32)
          n645 = case shown="True" w1267 {
            tunnel: w1270 -> [_ w1278]
            tunnel: w1269 -> [_ w1271]
            tunnel: w1268 -> [_ w1276]
            tunnel: w1266 -> [_ w1273]
            frame False {
            }
            frame True {
              n646 = Divide(x=w1271, y=w1273) -> (x/y=w1275:dbl)
              n647 = Array Subset(array=w1278, index=w1271) -> (w1277:T1[])  [unwired: 1 in]
              n648 = Multiply(x=w1275, y=30.0) -> (x*y=w1272:dbl)
              n649 = for {
                tunnel: w1277 -> [w1284] mode=indexing
                tunnel: w1276 -> [w1283]
                workers-P: _ -> [_]
                tunnel: w1272 -> [w1282]
                n650 = call "ColorRamp.vi"("Slide"=w1282) -> ("Color"=w1281:u32)
                n651 = call "IMAQ Overlay Text"("BG Color (Transparent)"=w1281, "Font, Size & Style"=T9 {"Desired Font (Application)"=enum."Application Font", "[User-specified Font]"={"Font Name"="", "Size"=1, "Strikeout?"=FALSE, "Italic?"=FALSE, "Underline?"=FALSE, "Outline?"=FALSE, "Shadow?"=FALSE, "Bold?"=FALSE, "Rotation Angle"=0.0}, "Horizontal Alignment"=1, "Vertical Alignment"=0}, "String"="   ", "Origin"=w1283, "Image"=w1284) -> ()  [unwired: 5 in, 2 out]
              }
            }
          }
          n652 = Increment(x=w1258) -> (x+1=w1265:i32)
          n653 = Divide(x=w1258, y=w1257) -> (x/y=w1264:dbl)
          n654 = local write "img"(w1265) -> ()
          n655 = Multiply(x=w1264, y=100.0) -> (x*y=w1263:dbl)
          n656 = local write "Slide"(w1263) -> ()
          n657 = Format Into String(initial string="Overlaying Well " ("Tutorial"), w1258) -> (resulting string=w1260:string)  [unwired: 2 in, 1 out]
          n658 = Format Into String(initial string=" of ", w1257) -> (resulting string=w1261:string)  [unwired: 2 in, 1 out]
          n659 = Concatenate Strings(w1260, w1261) -> (w1259:string)
          n660 = local write "Tutorial"(w1259) -> ()
        }
        n661 = call <vilib>:"Add State(s) to Queue__JKI_lib_State_Machine.vi"("State(s) in (\"\")"=w1254) -> ("States Out"=w1253:string)  [unwired: 14 in]
      }
      frame "Overlay: Overlay Freeze Temps" {
        # "Your code here.\n(You can make a copy of, or modify, this frame)"
        n662 = local read "FreezeTemps"() -> (w1288:dbl[])
        n663 = local read "FreezeArray"() -> (w1286:bool[])
        n664 = local read "FreezeIdx"() -> (w1287:i32[])
        n665 = local read "Points"() -> (w1289:T2[])
        n666 = Unbundle By Name(w1291) -> ("img_array"=w1290:T1[])
        n667 = call "OverlayFreezeRange.vi"("FreezeIdx"=w1287, "FreezeArray"=w1286) -> ("Range"=w1285:i32)
        n668 = for {
          N -> [w1295]
          tunnel: w1287 -> [w1310] mode=indexing
          tunnel: w1290 -> [w1311]
          tunnel: w1289 -> [w1309] mode=indexing
          tunnel: w1288 -> [w1308] mode=indexing
          tunnel: w1286 -> [w1307] mode=indexing
          tunnel: w1285 -> [w1306]
          n669 = local read "img"() -> (w1305:i32)
          n670 = case shown="True" w1307 {
            tunnel: w1311 -> [_ w1320]
            tunnel: w1310 -> [_ w1312]
            tunnel: w1309 -> [_ w1318]
            tunnel: w1308 -> [_ w1315]
            tunnel: w1306 -> [_ w1314]
            frame False {
            }
            frame True {
              n671 = Divide(x=w1312, y=w1314) -> (x/y=w1317:dbl)
              n672 = Array Subset(array=w1320, index=w1312) -> (w1319:T1[])  [unwired: 1 in]
              n673 = Multiply(x=w1317, y=30.0) -> (x*y=w1313:dbl)
              n674 = for {
                tunnel: w1319 -> [w1325] mode=indexing
                tunnel: w1318 -> [w1324]
                tunnel: w1315 -> [w1323]
                workers-P: _ -> [_]
                tunnel: w1313 -> [w1322]
                n675 = call "ColorRamp.vi"("Slide"=w1322) -> ("Color"=w1321:u32)
                n676 = Format Into String(format string="%3.2f", w1323) -> (resulting string=w1328:string)  [unwired: 2 in, 1 out]
                n677 = call "IMAQ Overlay Text"("BG Color (Transparent)"=w1321, "Font, Size & Style"=T9 {"Desired Font (Application)"=enum."Application Font", "[User-specified Font]"={"Font Name"="", "Size"=6, "Strikeout?"=FALSE, "Italic?"=FALSE, "Underline?"=FALSE, "Outline?"=FALSE, "Shadow?"=FALSE, "Bold?"=FALSE, "Rotation Angle"=0.0}, "Horizontal Alignment"=1, "Vertical Alignment"=0}, "String"=w1328, "Origin"=w1324, "Image"=w1325) -> ()  [unwired: 5 in, 2 out]
              }
            }
          }
          n678 = Increment(x=w1305) -> (x+1=w1299:i32)
          n679 = Divide(x=w1305, y=w1295) -> (x/y=w1300:dbl)
          n680 = local write "img"(w1299) -> ()
          n681 = Multiply(x=w1300, y=100.0) -> (x*y=w1301:dbl)
          n682 = local write "Slide"(w1301) -> ()
          n683 = Format Into String(initial string="Overlaying Well " ("Tutorial"), w1305) -> (resulting string=w1303:string)  [unwired: 2 in, 1 out]
          n684 = Format Into String(initial string=" of ", w1295) -> (resulting string=w1302:string)  [unwired: 2 in, 1 out]
          n685 = Concatenate Strings(w1303, w1302) -> (w1304:string)
          n686 = local write "Tutorial"(w1304) -> ()
        }
        n687 = call <vilib>:"Add State(s) to Queue__JKI_lib_State_Machine.vi"("State(s) in (\"\")"=w1294) -> ("States Out"=w1293:string)  [unwired: 14 in]
      }
      frame "Overlay: Overlay Freeze Old" {
        # "Your code here.\n(You can make a copy of, or modify, this frame)"
        n688 = local read "FreezeArray"() -> (w1330:bool[])
        n689 = Unbundle By Name(w1333) -> ("img_array"=w1335:T1[])
        n690 = local read "FreezeIdx"() -> (w1331:i32[])
        n691 = Unbundle By Name(w1333) -> ("Points.Pixels"=w1332:cluster{"X":i32, "Y":i32}[][])
        n692 = local read "Points"() -> (w1334:T2[])
        n693 = call "OverlayFreezeRange.vi"("FreezeIdx"=w1331, "FreezeArray"=w1330) -> ("Range"=w1329:i32)
        n694 = for {
          N -> [w1341]
          tunnel: w1331 -> [w1356] mode=indexing
          tunnel: w1335 -> [w1359]
          tunnel: w1334 -> [w1357] mode=indexing
          workers-P: _ -> [_]
          tunnel: w1329 -> [w1354]
          tunnel: w1332 -> [w1353] mode=indexing
          tunnel: w1330 -> [w1339] mode=indexing
          n695 = local read "img"() -> (w1342:i32)
          n696 = Increment(x=w1342) -> (x+1=w1347:i32)
          n697 = Divide(x=w1356, y=w1354) -> (x/y=w1355:dbl)
          n698 = Array Subset(array=w1359, index=w1356) -> (w1358:T1[])  [unwired: 1 in]
          n699 = local write "img"(w1347) -> ()
          n700 = Multiply(x=w1355, y=30.0) -> (x*y=w1352:dbl)
          n701 = Divide(x=w1342, y=w1341) -> (x/y=w1350:dbl)
          n702 = case shown="True" w1339 {
            tunnel: w1358 -> [_ w1363]
            tunnel: w1357 -> [_ w1362]
            tunnel: w1353 -> [_ w1361]
            tunnel: w1352 -> [_ w1360]
            frame False {
            }
            frame True {
              n703 = for {
                tunnel: w1363 -> [w1364] mode=indexing
                tunnel: w1362 -> [w1368]
                tunnel: w1360 -> [w1366]
                tunnel: w1361 -> [w1367]
                n704 = call "ColorRamp.vi"("Slide"=w1366) -> ("Color"=w1365:u32)
                n705 = call "IMAQ Overlay Points"("Color"=w1365, "Array of Points"=w1367, "Point"=w1368, "Image"=w1364) -> ()  [unwired: 6 in, 2 out]
              }
            }
          }
          n706 = Multiply(x=w1350, y=100.0) -> (x*y=w1349:dbl)
          n707 = local write "Slide"(w1349) -> ()
          n708 = Format Into String(w1342) -> (resulting string=w1345:string)  [unwired: 3 in, 1 out]
          n709 = Format Into String(w1341) -> (resulting string=w1346:string)  [unwired: 3 in, 1 out]
          n710 = Concatenate Strings("Overlaying Well " ("Tutorial"), w1345, " of " ("Tutorial"), w1346) -> (w1344:string)
          n711 = local write "Tutorial"(w1344) -> ()
        }
        n712 = call <vilib>:"Add State(s) to Queue__JKI_lib_State_Machine.vi"("State(s) in (\"\")"=w1338) -> ("States Out"=w1337:string)  [unwired: 14 in]
      }
      frame "Overlay: Remove Overlays" {
        # "Your code here.\n(You can make a copy of, or modify, this frame)"
        n713 = Unbundle By Name(w1370) -> ("img_array"=w1369:T1[])
        n714 = for {
          tunnel: w1369 -> [w1374] mode=indexing
          n715 = call "IMAQ Clear Overlay"("Image"=w1374) -> ()  [unwired: 9 in, 2 out]
        }
        n716 = call <vilib>:"Add State(s) to Queue__JKI_lib_State_Machine.vi"("State(s) in (\"\")"=w1373) -> ("States Out"=w1372:string)  [unwired: 14 in]
      }
      frame "Overlay: Update Focus Well" {
        # "Your code here.\n(You can make a copy of, or modify, this frame)"
        n717 = local read "FrozenFractionGraph"() -> (w1376:dbl[][])
        n718 = local read "FreezeIdx"() -> (w1378:i32[])
        n719 = local read "Temps"() -> (w1386:dbl[][])
        n720 = local read "PartitionArray"() -> (w1381:string[])
        n721 = local read "Temps grads"() -> (w1385:dbl[][])
        n722 = local read "MeltTemps"() -> (w1377:dbl[])
        n723 = call "PCRNameArray.vi"("input cluster"=w1380) -> ("WellArray"=w1379:string[])
        n724 = local read "FreezeTemps"() -> (w1384:dbl[])
        n725 = local read "Well"() -> (w1382:i32)
        n726 = Empty Array?(array=w1386) -> (empty?=w1383:bool)
        n727 = case shown="False" w1383 {
          tunnel: w1382 -> [w1392 _]
          tunnel: w1386 -> [w1408 _]
          tunnel: w1385 -> [w1407 _]
          tunnel: w1384 -> [w1406 _]
          tunnel: w1381 -> [w1391 _]
          tunnel: w1379 -> [w1403 _]
          tunnel: w1378 -> [w1399 _]
          tunnel: w1377 -> [w1398 _]
          tunnel: w1376 -> [w1396 _]
          frame False {
            n728 = call "WellPartition_Index.vi"("PartitionArray"=w1391, "Well"=w1392) -> ("Partition Index"=w1393:i32)  [unwired: 1 out]
            n729 = Index Array(array=w1398, index=w1392) -> (element=→"MeltTemp":dbl)
            n730 = Index Array(array=w1408, index (row)=w1392) -> (element=w1401:dbl[])  [unwired: 1 in]
            n731 = Index Array(array=w1406, index=w1392) -> (element=→"FreezeTemp":dbl)
            n732 = Index Array(array=w1407, index (row)=w1392) -> (element=→"Temps single grad":dbl[])  [unwired: 1 in]
            n733 = Index Array(array=w1391, index=w1392) -> (element=w1390:string)
            "Contents" <- w1390
            n734 = Index Array(array=w1403, index=w1392) -> (element=→"Well":string)
            n735 = Index Array(array=w1399, index=w1392) -> (element=w1394:i32)
            n736 = Index Array(array=w1396, index (row)=w1393) -> (element=→"Fraction Single":dbl[])  [unwired: 1 in]
            n737 = Index Array(array=w1401, index=w1394) -> (element=→"CurTemp":dbl)
            n738 = local write "ImageIdx"(w1394) -> ()
            n739 = local write "Temps single"(w1401) -> ()
            n740 = property on="Fraction Single" class="WFGraph (strict)"("Plot.Plot Name"=w1390) -> ()  [unwired: 2 in, 2 out]
          }
          frame True {
          }
        }
        n741 = call <vilib>:"Add State(s) to Queue__JKI_lib_State_Machine.vi"("State(s) in Front (\"\")"="Image: Set Cursors" ("State(s) in Front (\"\")"), "State(s) in (\"\")"=w1389) -> ("States Out"=w1388:string)  [unwired: 13 in]
      }
    }
  }
